vi "Main.vi"(11 "Module Admin":refnum<class "Delacor_lib_QMH_Module Admin.lvclass">) -> ()   [LabVIEW 2025, in "Scripting Server.lvlib"]
doc: "This template is based off of the Queued Message Handler design pattern and the Queued Message Handler project template that ships with LabVIEW.\n\nThe main difference is that the queue is private to this module and communication between modules is performed via Broadcast and Request events.\n\nRequest events are wrapped in public API methods and are handled in the Event Handling Loop (EHL) of this VI. Any module can register for Broadcast events sent by this module. The EHL generates messages based on user interface actions.\n\nThe Message Handling Loop (MHL) processes messages generated by the EHL, or by other messages. The messages are string values, so new messages can be added easily to the Message Cases case structure in the MHL. Each message cluster can also provide an optional value for Message Data, which is a variant that can be converted to whatever message-specific data is required.\n_____\nBased on DQMH Dev Tools: Project Template 7.1.0.1503."
uses:
  Scripting Server.lvlib
  <vilib>/Delacor/Delacor QMH/Libraries/Module Admin_class/Delacor_lib_QMH_Module Admin.lvclass
  <vilib>/Delacor/Delacor QMH/Libraries/Message Queue_class/Delacor_lib_QMH_Message Queue.lvclass
  Module Data--cluster.ctl
  <vilib>/Utility/miscctls.llb/LVPointTypeDef.ctl
  <vilib>/Delacor/Delacor QMH/Libraries/Message Queue_class/Delacor_lib_QMH_Enqueue Message (Single).vi
  Stop Argument--cluster.ctl
  New VI (Reply Payload)--cluster.ctl
  New VI Argument--cluster.ctl
  Add Object Argument--cluster.ctl
  Add Object (Reply Payload)--cluster.ctl
  Connect Objects (Reply Payload)--cluster.ctl
  Connect Objects Argument--cluster.ctl
  Get Object Terminals (Reply Payload)--cluster.ctl
  Get Object Terminals Argument--cluster.ctl
  get vi error list (Reply Payload)--cluster.ctl
  get vi error list Argument--cluster.ctl
  Cleanup VI (Reply Payload)--cluster.ctl
  Cleanup VI Argument--cluster.ctl
  create_control (Reply Payload)--cluster.ctl
  create_control Argument--cluster.ctl
  Run VI (Reply Payload)--cluster.ctl
  Run VI Argument--cluster.ctl
  add_to_selection (Reply Payload)--cluster.ctl
  add_to_selection Argument--cluster.ctl
  clear_selection_list (Reply Payload)--cluster.ctl
  clear_selection_list Argument--cluster.ctl
  remove_from_selection (Reply Payload)--cluster.ctl
  remove_from_selection Argument--cluster.ctl
  enclose_selection (Reply Payload)--cluster.ctl
  enclose_selection Argument--cluster.ctl
  rename_object (Reply Payload)--cluster.ctl
  rename_object Argument--cluster.ctl
  set_value (Reply Payload)--cluster.ctl
  set_value Argument--cluster.ctl
  delete_object (Reply Payload)--cluster.ctl
  delete_object Argument--cluster.ctl
  save_vi (Reply Payload)--cluster.ctl
  save_vi Argument--cluster.ctl
  get_structure_diagram (Reply Payload)--cluster.ctl
  get_structure_diagram Argument--cluster.ctl
  add_subvi (Reply Payload)--cluster.ctl
  add_subvi Argument--cluster.ctl
  connect_to_pane (Reply Payload)--cluster.ctl
  connect_to_pane Argument--cluster.ctl
  get_object_help (Reply Payload)--cluster.ctl
  get_object_help Argument--cluster.ctl
  get_loop_conditional_terminal (Reply Payload)--cluster.ctl
  get_loop_conditional_terminal Argument--cluster.ctl
  show_conditional_terminal (Reply Payload)--cluster.ctl
  show_conditional_terminal Argument--cluster.ctl
  get_loop_iteration_terminal (Reply Payload)--cluster.ctl
  get_loop_iteration_terminal Argument--cluster.ctl
  Config Data.ctl
  Read Config Data Argument--cluster.ctl
  get_allowed_paths (Reply Payload)--cluster.ctl
  get_allowed_paths Argument--cluster.ctl
  create_project (Reply Payload)--cluster.ctl
  create_project Argument--cluster.ctl
  Set Allowed Paths Argument--cluster.ctl
  open_vi (Reply Payload)--cluster.ctl
  open_vi Argument--cluster.ctl
  New MCP RPC Message Argument--cluster.ctl
  <vilib>/jgoebel/LabVIEW MCP Server SDK/MCP Server.lvlib
  <vilib>/jgoebel/LabVIEW MCP Server SDK/onRpc.ctl
  <vilib>/jgoebel/LabVIEW MCP Server SDK/User Events.ctl
  get-available-objects (Reply Payload)--cluster.ctl
  get-available-objects Argument--cluster.ctl
  Get open VIs (Reply Payload)--cluster.ctl
  Get open VIs Argument--cluster.ctl
  Get VI Blockdiagram (Reply Payload)--cluster.ctl
  Get VI Blockdiagram Argument--cluster.ctl
  Get VI Frontpanel Picture (Reply Payload)--cluster.ctl
  Get VI Frontpanel Picture Argument--cluster.ctl
  Get Library (Reply Payload)--cluster.ctl
  Get Library Argument--cluster.ctl
panel:
  out "Log":string
  in  "Ring 2":i32(ring)=2125 items=[".NET Container"=2125, ".NET Refnum"=3441, "2D Picture"=3508, "3D Picture"=23776, "Absolute Value"=1054, "Accept TLS"=1732, "Access Rights"=1412, "ActiveX Container"=2072, "Add"=1050, "Add (with error terminals)"=3915, "Add Array Elements"=1903, "Add Entropy"=1738, "Add Private Key To TLS Configuration"=1735, "Add Trusted Certificate To TLS Configuration"=1736, "Agitator"=3831, "AllSpoll"=1960, "Always Copy"=2400, "And"=1061, "And Array Elements"=1911, "Append True/False String"=1511, "Application Refnum"=3412, "Array (block diagram constant)"=2070, "Array (classic)"=3300, "Array (modern)"=21608, "Array Interface Control"=23777, "Array Max & Min"=1907, "Array of Strings to Path"=1422, "Array Size"=1809, "Array Subset"=2044, "Array To Cluster"=1168, "Array To Spreadsheet String"=1540, "ArrayMemInfo"=2412, "Assert Structural Type Match"=2416, "Assert Structural Type Mismatch"=2464, "Atmospheric Tank (classic)"=3070, "Atmospheric Tank (modern)"=21751, "Automation Close"=8001, "Automation Open"=8000, "Automation Refnum"=3410, "Avogadro Constant (1/mol)"=23520, "Base 10 Logarithm Of e"=23512, "Bin #1"=3073, "Bin #2"=21755, "Bitpack to Array"=3135, "Bluetooth Close Connection"=9148, "Bluetooth Create Listener"=9151, "Bluetooth Discover"=9152, "Bluetooth Network Connection Refnum"=3468, "Bluetooth Open Connection"=9153, "Bluetooth Read"=9149, "Bluetooth Wait On Listener"=9147, "Bluetooth Write"=9150, "Boolean Array To Number"=1815, "Boolean To (0,1)"=1167, "Build Array"=2041, "Build Cluster Array"=2047, "Build Map"=2463, "Build Matrix"=8500, "Build Path"=1419, "Build Set"=2462, "Build Waveform"=2066, "Bundle"=2049, "Bundle By Name"=2057, "Byte Array To String"=1609, "Byte Array To UTF-8 String"=1651, "Byte Stream File Refnum"=3408, "Call By Reference"=3901, "Call Chain"=1999, "Call Library Function Node"=2062, "Call MATLAB Function"=24210, "Call Parent Class Method"=2354, "CAN Channel (block diagram constant)"=2124, "CAN Channel (classic)"=3340, "CAN Channel (modern)"=21817, "CAN Channel (system)"=21966, "CAN Interface (block diagram constant)"=2123, "CAN Interface (classic)"=3339, "CAN Interface (modern)"=21815, "CAN Interface (system)"=21964, "CAN Task (block diagram constant)"=3471, "CAN Task (classic)"=3470, "CAN Task (modern)"=21789, "CAN Task (system)"=21963, "Cancel Button (modern)"=21739, "Cancel Button (system)"=3131, "Cancel Notification"=9107, "Carriage Return Constant"=23500, "Case Structure"=2001, "Cast Unit Bases"=1079, "Check Valve"=3833, "Checkbox (classic)"=3117, "CheckBox (modern)"=21924, "Checkbox (system)"=3132, "Class Specifier Constant"=2094, "Classic Color Box"=3013, "Classic Color Ramp"=3022, "Classic Horizontal Slide Switch"=3114, "Classic Vertical Slide"=3004, "Clear Fixed-Point Overflow Status"=5562, "Close File"=8052, "Close File (deprecated)"=1405, "Close MATLAB Session"=24209, "Close Python Session"=24207, "Close Reference"=8011, "Close TLS Configuration"=1741, "Close Variable Connection"=23783, "Closure Structure"=2372, "Cluster (classic)"=3400, "Cluster (modern)"=21607, "Cluster Constant"=2071, "Cluster To Array"=1169, "Code Interface Node"=2050, "Coerce To Type"=2402, "Collection Size"=2450, "Color Box Constant"=2120, "Color Box Thin Border"=2905, "Colored Rectangle (broken?)"=3625, "Combo Box (classic)"=3304, "Combo Box (modern)"=21604, "Combo Box (system)"=21917, "Combo Box Constant"=2088, "Complex Conjugate"=1048, "Complex To Polar"=1045, "Complex To Re/Im"=1044, "Compound Arithmetic"=2200, "Compressor"=3832, "Concatenate Strings"=2040, "Conditional Disable Structure"=2064, "Constructor Node"=3904, "Control & Simulation Loop"=2099, "Control Help Window"=1353, "Control Online Help"=1355, "Control Refnum"=3419, "Convert Unit"=2059, "Conveyer"=3827, "Copy"=8053, "Copy (deprecated)"=1416, "Cosecant"=1204, "Cosine"=1201, "Cotangent"=1205, "CPU Information"=24130, "Create Folder"=8055, "Create Network Stream Endpoint"=23793, "Create Network Stream Reader Endpoint"=23811, "Create Network Stream Writer Endpoint"=23810, "Create Stream"=23796, "Create Unique Network Stream Endpoint"=23795, "Create Unique Network Stream Reader Endpoint"=23807, "Create Unique Network Stream Writer Endpoint"=23806, "Create User Event"=2073, "Current Processor ID"=24131, "Current VI's Menubar"=9000, "Current VI's Path"=1426, "DAQmx Analog Trigger Source (block diagram constant)"=2119, "DAQmx Analog Trigger Source (classic)"=3336, "DAQmx Analog Trigger Source (modern)"=21774, "DAQmx Analog Trigger Source (system)"=21951, "DAQmx Device Name (block diagram constant)"=2093, "DAQmx Device Name (classic)"=3318, "DAQmx Device Name (modern)"=21773, "DAQmx Device Name (system)"=21950, "DAQmx Global Channel (block diagram constant)"=3430, "DAQmx Global Channel (classic)"=3443, "DAQmx Global Channel (modern)"=21770, "DAQmx Global Channel (system)"=21957, "DAQmx Physical Channel (block diagram constant)"=2118, "DAQmx Physical Channel (classic)"=3335, "DAQmx Physical Channel (modern)"=21777, "DAQmx Physical Channel (system)"=21954, "DAQmx Scale Name (block diagram constant)"=2116, "DAQmx Scale Name (classic)"=3317, "DAQmx Scale Name (modern)"=21775, "DAQmx Scale Name (system)"=21952, "DAQmx Switch (block diagram constant)"=2121, "DAQmx Switch (classic)"=3337, "DAQmx Switch (modern)"=21776, "DAQmx Switch (system)"=21953, "DAQmx Task Name (block diagram constant)"=3434, "DAQmx Task Name (classic)"=3442, "DAQmx Task Name (modern)"=21778, "DAQmx Task Name (system)"=21959, "DAQmx Terminal (block diagram constant)"=2117, "DAQmx Terminal (classic)"=3319, "DAQmx Terminal (modern)"=21781, "DAQmx Terminal (system)"=21955, "Data Cache Size"=24132, "Data Log File Refnum"=3402, "Data Value Reference"=3476, "Data Value Reference Constant"=24134, "DataSocket Close"=1085, "DataSocket Open"=1084, "DataSocket Read"=1086, "DataSocket Refnum"=3417, "DataSocket Write"=1087, "Date/Time To Seconds"=1308, "Decimal Digit?"=1119, "Decimal String To Number"=1184, "Decimate 1D Array"=2046, "DecomposeLockDataValRef"=2406, "DecomposeVariant"=2404, "Decrement"=1058, "Default Directory"=1427, "Delete"=8056, "Delete (deprecated)"=1417, "Delete Data Value Reference"=2409, "Delete From Array"=3912, "Delete Menu Items"=9004, "Delete Variant Attribute"=8206, "Delete Waveform Attribute"=8209, "Deny Access"=8057, "Dequeue Element"=9113, "Destroy Stream Endpoint"=23794, "Destroy User Event"=2075, "DevClear"=1961, "DevClearList"=1962, "Device Control/Status"=1433, "Device Refnum"=3405, "Diagram Disable Structure"=2054, "Dial (classic)"=3050, "Dial (modern)"=21732, "Digital Data (classic)"=3210, "Digital Data (modern)"=21216, "Digital Waveform Graph (classic)"=3511, "Digital Waveform Graph (modern)"=21718, "Direct Variable Read"=23785, "Direct Variable Write"=23788, "Divide"=1053, "Divide (with error terminals)"=3918, "Dlg Horiz Scrollbar"=21905, "Dlg Mac Group Box"=32514, "Dlg Numeric #1"=2100, "Dlg Numeric #2"=3006, "Dlg String"=2110, "Dlg Vert Scrollbar"=21906, "Down Arrow"=3824, "Down Bow Valve (flat)"=3707, "Down Bow Valve (outline)"=3807, "Down Bow Valve (shaded)"=21767, "Down Rect Valve (flat)"=3706, "Down Rect Valve (outline)"=3806, "Down Rect Valve (shaded)"=21766, "Down Tee (flat)"=3818, "Down Tee (shaded)"=3718, "Dynamic FPGA Interface Cast"=5690, "Eased Corner Rectangle"=32513, "Element of Set?"=2454, "Elementary Charge (C)"=23517, "Empty Array?"=23063, "Empty Collection?"=2451, "Empty Path Constant"=23523, "Empty String Constant"=23503, "Empty String/Path?"=1112, "Enable Menu Tracking"=9002, "EnableLocal"=1963, "EnableRemote"=1964, "End of Line Constant"=23525, "Enqueue Element"=9111, "Enqueue Element At Opposite End"=9129, "Enum (classic)"=3023, "Enum (modern)"=21605, "Enum (system)"=3062, "Enum Constant"=2090, "EOF"=1410, "Equal To 0?"=1113, "Equal?"=1102, "Error Ring Constant"=2039, "Event Callback Refnum"=3435, "Event Data Node"=2102, "Event Structure"=2052, "Exchanger"=3828, "Exclusive Or"=1063, "Exponential"=1211, "Exponential (Arg) -1"=1222, "Expression Node"=2201, "False Constant"=2006, "Feedback Node"=2353, "FieldPoint IO Point (block diagram constant)"=3440, "FieldPoint IO Point (classic)"=3439, "FieldPoint IO Point (modern)"=21784, "FIFO Refnum"=3474, "File Dialog"=8058, "File Dialog (deprecated)"=8081, "File Path Control (classic)"=3203, "File Path Control (modern)"=21730, "File Path Control (system)"=21922, "File Path Indicator (classic)"=3204, "File Path Indicator (modern)"=21731, "File/Directory Info"=8082, "File/Directory Info (deprecated)"=1413, "FindLstn"=1965, "FindRQS"=1966, "First Call?"=1083, "Fixed-Point Overflow?"=5565, "Fixed-Point to Integer Cast"=5566, "Flat Box"=3602, "Flat Circle"=3605, "Flat Down Triangle"=3623, "Flat Frame"=3608, "Flat Left Triangle"=3620, "Flat Right Triangle"=3621, "Flat Round Button"=3102, "Flat Rounded Box"=3611, "Flat Sequence Structure"=2069, "Flat Square Button"=3103, "Flat Up Triangle"=3622, "Flatten To JSON"=24201, "Flatten To String"=1164, "Flatten To XML"=8402, "Flattened String To Variant"=8202, "Floating Point Equal?"=23064, "Flush Event Queue"=2135, "Flush File"=8059, "Flush File (deprecated)"=1406, "Flush Queue"=9114, "Flush Stream"=23808, "For Loop"=2002, "Fork"=2194, "Format Date/Time String"=8100, "Format Into File"=2083, "Format Into String"=2081, "Format Value"=1512, "Formula Node"=2004, "FPGA Refnum to Session"=2322, "Fract/Exp String To Number"=1187, "Framed Color Box (classic)"=3008, "Framed Color Box (modern)"=21019, "Free Label"=2321, "Furnace"=3829, "Gauge (classic)"=3040, "Gauge (modern)"=21009, "Gauge for Simon"=32600, "Generate Front Panel Activity"=1329, "Generate Occurrence"=1700, "Generate User Event"=2074, "Generate User-Defined Trace Event"=2250, "Get Control Values by Index"=24204, "Get Datalog Position"=8061, "Get Date/Time In Seconds"=1303, "Get Date/Time String"=1600, "Get Drag Drop Data"=9154, "Get File Position"=8062, "Get File Size"=8063, "Get Fixed-Point Components"=11163, "Get Help Window Status"=1354, "Get Matrix Diagonal"=8501, "Get Matrix Elements"=8502, "Get Menu Item Info"=9005, "Get Menu Selection"=9001, "Get Menu Short Cut Info"=9007, "Get Notifier Status"=9103, "Get Number of Records"=8064, "Get Permissions"=8065, "Get Queue Status"=9110, "Get Submatrix"=8503, "Get Type and Creator"=8066, "Get Variant Attribute"=8205, "Get Volume Info"=8067, "Get Waveform Attribute"=8208, "Get Waveform Components"=2067, "Global Variable"=2060, "GPIB Clear"=1954, "GPIB Initialization"=1957, "GPIB Misc"=1956, "GPIB Read"=1951, "GPIB Serial Poll"=1955, "GPIB Status"=1959, "GPIB Trigger"=1953, "GPIB Wait"=1958, "GPIB Write"=1950, "Gravitational Constant (N m2/kg2)"=23519, "Greater Or Equal To 0?"=1114, "Greater Or Equal?"=1103, "Greater Than 0?"=1117, "Greater?"=1110, "Handle Peek"=1604, "Handle Poke"=1605, "Hex Digit?"=1123, "Hexadecimal String To Number"=1185, "Hopper #1"=21754, "Hopper #2"=3072, "Horiz Line"=3821, "Horiz Pipe (flat)"=3810, "Horiz Pipe (shaded)"=3710, "Horizontal Button Box"=3636, "Horizontal Fill Slide (classic)"=3012, "Horizontal Fill Slide (modern)"=21100, "Horizontal Gradient Oval"=32502, "Horizontal Gradient Rectangle"=32504, "Horizontal Gradient Rounded Rectangle"=32507, "Horizontal Graduated Bar"=21106, "Horizontal Pointer Slide (classic)"=3011, "Horizontal Pointer Slide (modern)"=21101, "Horizontal Pointer Slide (system)"=21902, "Horizontal Progress Bar (modern)"=21102, "Horizontal Progress Bar (system)"=21910, "Horizontal Scrollbar"=21110, "Horizontal Slide (classic)"=3010, "Horizontal Slide (system)"=21904, "Horizontal Smooth Box"=3633, "Horizontal Splitter Bar"=21861, "Horizontal Splitter Bar (Classic)"=21863, "Horizontal Splitter Bar (NXG Style)"=21867, "Horizontal Splitter Bar (System)"=21865, "Horizontal Switch"=3108, "Horizontal Tank"=3071, "Horizontal Toggle Switch (classic)"=3110, "Horizontal Toggle Switch (modern)"=21700, "Hyperbolic Cosecant"=23053, "Hyperbolic Cosine"=1215, "Hyperbolic Cotangent"=23055, "Hyperbolic Secant"=23054, "Hyperbolic Sine"=1214, "Hyperbolic Tangent"=1216, "IMAQ Session"=3415, "Implies"=1080, "In Place Element Structure"=2360, "In Range and Coerce"=1127, "Include Fixed-Point Overflow Status"=5564, "Increment"=1057, "Index & Bundle Cluster Array"=2056, "Index Array"=2042, "Index String Array"=1531, "Initialize Array"=2053, "Inline C Node"=2104, "Insert Into Array"=3911, "Insert Into Map"=2456, "Insert Into Set"=2452, "Insert Menu Items"=9003, "Integer to Fixed-Point Cast"=5567, "Intensity Chart (classic)"=3509, "Intensity Chart (modern)"=21719, "Intensity Graph (classic)"=3510, "Intensity Graph (modern)"=21720, "Interleave 1D Arrays"=2045, "Interpolate 1D Array"=1905, "Inverse Cosecant"=23050, "Inverse Cosine"=1207, "Inverse Cotangent"=23052, "Inverse Hyperbolic Cosecant"=23056, "Inverse Hyperbolic Cosine"=1218, "Inverse Hyperbolic Cotangent"=23058, "Inverse Hyperbolic Secant"=23057, "Inverse Hyperbolic Sine"=1217, "Inverse Hyperbolic Tangent"=1219, "Inverse Secant"=23051, "Inverse Sine"=1206, "Inverse Tangent"=1208, "Inverse Tangent (2 Input)"=1228, "Invoke Node"=3900, "IP To String"=1710, "IrDA Close Connection"=9144, "IrDA Create Listener"=9140, "IrDA Discover"=9141, "IrDA Network Connection Refnum"=3450, "IrDA Open Connection"=9142, "IrDA Read"=9145, "IrDA Wait On Listener"=9143, "IrDA Write"=9146, "IsDebuggingActive"=2403, "IVI Delete Session"=8103, "IVI Logical Name (block diagram constant)"=3420, "IVI Logical Name (classic)"=3414, "IVI Logical Name (modern)"=21736, "IVI New Session"=8102, "Join"=2195, "Join Numbers"=1171, "Junction"=2197, "Knob (classic)"=3005, "Knob (modern)"=21000, "Label (modern)"=21960, "Label (system)"=21961, "Labeled Oblong Button"=3125, "Labeled Rectangular Button"=3124, "Labeled Round Button"=3122, "Labeled Square Button"=3123, "LabVIEW Object"=3457, "Leak Variant Value Reference"=2410, "LED Button"=3116, "Left Arrow"=3826, "Left Bow Valve (flat)"=3701, "Left Bow Valve (outline)"=3801, "Left Bow Valve (shaded)"=21761, "Left Down Elbow (flat)"=3811, "Left Down Elbow (shaded)"=3711, "Left Pump (flat)"=3813, "Left Pump (shaded)"=3713, "Left Rect Valve (flat)"=3700, "Left Rect Valve (outline)"=3800, "Left Rect Valve (shaded)"=21760, "Left Tee (flat)"=3809, "Left Tee (shaded)"=3709, "Left Up Elbow (flat)"=3808, "Left Up Elbow (shaded)"=3708, "Less Or Equal To 0?"=1115, "Less Or Equal?"=1104, "Less Than 0?"=1118, "Less?"=1111, "Lexical Class"=1126, "Line (chiseled, system)"=3632, "Line (chiseled, thick)"=3630, "Line (chiseled, thin)"=3627, "Line (thick)"=3629, "Line (thin)"=3626, "Line Feed Constant"=23501, "Line with Arrow (thick)"=3631, "Line with Arrow (thin)"=3628, "List Directory"=1418, "List Folder"=8083, "Listbox (classic)"=21806, "Listbox (modern)"=21792, "Listbox (system)"=21805, "Listbox Symbol Ring Constant"=2038, "Load Certificates Into Memory"=1734, "Load Private Key Into Memory"=1733, "Local Variable"=2061, "Lock Range"=1411, "Logarithm Base 10"=1210, "Logarithm Base 2"=1225, "Logarithm Base X"=1224, "Logical Shift"=1081, "Look In Map"=2458, "Lookup Channel Probe"=9155, "Lossy Enqueue Element"=9130, "Lowered Box (thick)"=3635, "Lowered Rounded Box"=3638, "Machine Epsilon"=23528, "Make TLS Configuration Immutable"=1737, "MakeAddr"=1967, "Mantissa & Exponent"=1150, "Map"=3488, "Map Constant"=2461, "Match First String"=1532, "Match Pattern"=1535, "Match True/False String"=1533, "MathScript Call By Reference"=3906, "MathScript Node"=2357, "MATLAB script"=9020, "MATLAB Session Refnum"=3490, "Matrix Size"=8507, "Max & Min"=1108, "Menu Refnum"=3413, "Menu Ring (classic)"=3018, "Menu Ring (modern)"=21600, "Menu-Popup Ring"=3017, "Merge Errors"=2147, "Merge Signals"=2350, "Meter (classic)"=3030, "Meter (modern)"=21008, "Mixed Checkbox (system)"=21333, "Mixed Signal Graph"=21721, "Molar Gas Constant (J/(mol K))"=23522, "Motion Resource (block diagram constant)"=3449, "Motion Resource (classic)"=3448, "Motion Resource (modern)"=21787, "Motor (flat)"=3820, "Motor (shaded)"=3720, "Move"=8068, "Move (deprecated)"=1415, "Multi-Segment Pipe"=23780, "Multicolumn Listbox (classic)"=21799, "Multicolumn Listbox (modern)"=21791, "Multicolumn Listbox (system)"=21798, "Multiply"=1052, "Multiply (with error terminals)"=3917, "Multiply Array Elements"=1904, "Multirate Structure"=2199, "Natural Logarithm"=1209, "Natural Logarithm (Arg +1)"=1221, "Natural Logarithm Base"=23510, "Natural Logarithm Of 10"=23513, "Natural Logarithm Of 2"=23514, "Natural Logarithm Of Pi"=23508, "Negate"=1069, "Negative Infinity"=23509, "New Data Value Reference"=2408, "New Directory"=1402, "New File"=1404, "New TLS Configuration"=1730, "New VI"=8014, "New VI Object"=8015, "Not"=1064, "Not A Number/Path/Refnum?"=1128, "Not A Path Constant"=23524, "Not a Refnum Constant"=23526, "Not a Shared Variable"=23527, "Not And"=1071, "Not Equal To 0?"=1116, "Not Equal?"=1105, "Not Exclusive Or"=1073, "Not Or"=1072, "Notifier Refnum"=3423, "Number of Cache Levels"=24133, "Number To Boolean Array"=1814, "Number To Decimal String"=1180, "Number To Engineering String"=1183, "Number To Exponential String"=1505, "Number To Fractional String"=1506, "Number To Hexadecimal String"=1181, "Number To Octal String"=1182, "Numeric Constant"=2005, "Numeric Control (classic)"=3000, "Numeric Control (modern)"=21003, "Numeric Control (system)"=21919, "Numeric Indicator (classic)"=3001, "Numeric Indicator (modern)"=21004, "Obtain Notifier"=9101, "Obtain Queue"=9108, "Occurrence Refnum"=3406, "Octal Digit?"=1129, "Octal String To Number"=1186, "OK Button (modern)"=21738, "OK Button (system)"=3130, "Old VISA Open"=1921, "OLE Variant"=3150, "One Button Dialog"=1340, "Open and Verify Variable Connection"=23790, "Open Application Reference"=8012, "Open Device"=1430, "Open Dynamic Bitfile Reference"=5691, "Open File"=1403, "Open MATLAB Session"=24208, "Open Python Session"=24206, "Open Tank (flat classic)"=21752, "Open Tank (shaded classic)"=3074, "Open Variable Connection"=23779, "Open Variable Connection in Background"=23791, "Open VI Object Reference"=8013, "Open VI Reference"=8010, "Open/Create/Replace Datalog"=8054, "Open/Create/Replace File"=8050, "Or"=1062, "Or Array Elements"=1910, "Oval with Shadow"=32509, "Package Matrix"=23001, "PassControl"=1968, "Path Constant"=2009, "Path to Array of Strings"=1423, "Path To String"=1077, "Path Type"=1421, "Pi"=23504, "Pi Divided By 2"=23506, "Pi Multiplied By 2"=23505, "Pick Line"=1510, "Pict Ring (classic)"=3015, "Pict Ring (modern)"=21602, "Pict Ring (system)"=21925, "PixMap"=3505, "PixMap (warning: dangerous)"=3507, "Planck's Constant (J/Hz)"=23516, "Platform Flat Square Button"=3134, "Plug-In Control"=21820, "Polar To Complex"=1047, "Polar To Re/Im"=23061, "Positive Infinity"=23515, "Power Of 10"=1212, "Power Of 2"=1223, "Power Of X"=1213, "PPoll"=1969, "PPollConfig"=1970, "PPollUnconfig"=1971, "Preallocated Read from Binary File"=24135, "Preserve Run-Time Class"=8018, "Pressure Tank (flat)"=3075, "Pressure Tank (shaded)"=21753, "Preview Queue Element"=9112, "Printable?"=1124, "Property Node"=1920, "Pulldown Menu Ring"=3061, "Push Button"=21001, "Python Node"=24205, "Python Session Refnum"=3486, "Queue Refnum"=3424, "Quit LabVIEW"=1352, "Quotient & Remainder"=1056, "Race Structure"=2371, "Radio Button (system)"=3133, "Radio Buttons (classic)"=22003, "Radio Buttons (modern)"=22001, "Radio Buttons (system)"=22002, "Raised Box (classic)"=3600, "Raised Box (modern)"=3637, "Raised Circle"=3603, "Raised Down Triangle"=3615, "Raised Frame"=3606, "Raised Left Triangle"=3612, "Raised Right Triangle"=3613, "Raised Rounded Box"=3609, "Raised Up Triangle"=3614, "Random Number (0-1)"=1070, "RcvRespMsg"=1972, "Re-accept TLS"=1739, "Re/Im To Complex"=1046, "Re/Im To Polar"=23060, "Read Datalog"=8069, "Read Device"=1432, "Read File"=1407, "Read from Binary File"=8051, "Read from Text File"=8070, "Read Map Max & Min Keys"=2459, "Read Multiple Elements from Stream"=23803, "Read Set Max & Min"=2455, "Read Single Element from Stream"=23797, "Read Variable"=23781, "Read Variable with Timeout"=23786, "ReadStatus"=1973, "Receive"=1974, "ReceiveSetup"=1975, "Recessed Box"=3601, "Recessed Circle"=3604, "Recessed Down Triangle"=3619, "Recessed Frame (modern)"=3607, "Recessed Frame (system)"=3624, "Recessed Left Triangle"=3616, "Recessed Menu Ring"=3019, "Recessed Right Triangle"=3617, "Recessed Rounded Box"=3610, "Recessed Up Triangle"=3618, "Reciprocal"=1059, "Reciprocal Of e"=23511, "Reciprocal Of Pi"=23507, "RecomposeUnlockDataValRef (warning: dangerous)"=2407, "RecomposeVariant (warning: dangerous)"=2405, "Rectangular Stop Button"=3128, "Refnum to Path"=1424, "Refnum to Session"=2306, "Region"=2196, "Register Event Callback"=2078, "Register For Events"=2065, "Register Session"=2319, "Release Notifier"=9102, "Release Queue"=9109, "Remove Fixed-Point Overflow Status"=5563, "Remove From Map"=2457, "Remove From Set"=2453, "Replace Array Subset"=3910, "Replace Substring"=3913, "Request Deallocation"=1610, "ResetSys"=1976, "Reshape Array"=2055, "Resize Matrix"=8508, "Resource Index"=1088, "Reverse 1D Array"=1900, "Reverse String"=1537, "Right Arrow"=3825, "Right Bow Valve (flat)"=3705, "Right Bow Valve (outline)"=3805, "Right Bow Valve (shaded)"=21765, "Right Down Elbow (flat)"=3817, "Right Down Elbow (shaded)"=3717, "Right Pump (flat)"=3819, "Right Pump (shaded)"=3719, "Right Rect Valve (flat)"=3704, "Right Rect Valve (outline)"=3804, "Right Rect Valve (shaded)"=21764, "Right Tee (flat)"=3815, "Right Tee (shaded)"=3715, "Right Up Elbow (flat)"=3814, "Right Up Elbow (shaded)"=3714, "Rocker"=21002, "Rotary Feeder"=3830, "Rotate"=1082, "Rotate 1D Array"=1906, "Rotate Left With Carry"=1606, "Rotate Right With Carry"=1607, "Rotate String"=1536, "Round Button"=3100, "Round LED (classic)"=3120, "Round LED (modern)"=21012, "Round Light"=3104, "Round Push Button"=3118, "Round Push Button (profile)"=3112, "Round Radio Button"=3106, "Round Stop Button"=3127, "Round To Nearest"=1055, "Round Toward +Infinity"=1076, "Round Toward -Infinity"=1075, "Rounded Rectangle with Shadow"=32508, "RT FIFO Create"=24000, "RT FIFO Delete"=24003, "RT FIFO Read"=24001, "RT FIFO Write"=24002, "Rydberg Constant (1/m)"=23521, "Scale By Power Of 2"=1074, "Scan From File"=2082, "Scan From String"=2080, "Scan String For Tokens"=8101, "Scan Value"=1534, "Scanned Variable Read"=23784, "Scanned Variable Write"=23787, "Search 1D Array"=1901, "Search and Replace String"=3914, "Search Variable Container"=23802, "Search/Split String"=1538, "Secant"=1203, "Seconds To Date/Time"=1309, "Seek"=1409, "Select"=1516, "Send"=1977, "Send Notification"=9104, "SendCmds"=1978, "SendDataBytes"=1979, "SendIFC"=1980, "SendList"=1981, "SendLLO"=1982, "SendSetup"=1983, "Session to Refnum"=2307, "Set"=3487, "Set Constant"=2460, "Set Control Values by Index"=24203, "Set Datalog Position"=8072, "Set File Position"=8073, "Set File Size"=8074, "Set Matrix Diagonal"=8504, "Set Matrix Elements"=8505, "Set Menu Item Info"=9006, "Set Number of Records"=8075, "Set Occurrence"=1702, "Set Permissions"=8076, "Set Submatrix"=8506, "Set Type and Creator"=8077, "Set Variant Attribute"=8204, "Set Waveform Attribute"=8207, "SetRWLS"=1984, "SetTimeOut"=1985, "Shared Variable"=23778, "Shared Variable Constant"=3473, "Shared Variable Control (classic)"=3472, "Shared Variable Control (modern)"=21814, "Shared Variable to String"=1831, "Sign"=1049, "Simple Horizontal Slide"=3003, "Simple Numeric"=2900, "Simple String"=2115, "Simple Vertical Slide"=3002, "Sinc"=1227, "Sine"=1200, "Sine & Cosine"=1220, "Size Handle"=1603, "Slide Switch"=21011, "Smoothed Oval"=32500, "Smoothed Rounded Rectangle"=32505, "Sort 1D Array"=1120, "Sort Array of String"=23065, "Speed Of Light In Vacuum (m/sec)"=23518, "Spin Control (system)"=21900, "Split 1D Array"=1908, "Split Button"=21020, "Split Number"=1170, "Split Signals"=2351, "Spreadsheet String To Array"=1539, "Square"=23059, "Square Button"=3101, "Square LED (classic)"=3121, "Square LED (modern)"=21013, "Square Light"=3105, "Square Push Button"=3119, "Square Push Button (profile)"=3113, "Square Radio Button"=3107, "Square Root"=1060, "Stacked Sequence Structure"=2000, "Start TLS"=1731, "State"=2198, "State Diagram"=2051, "Static VI Reference"=2084, "Stop"=1350, "Stop Button"=21230, "String Constant"=2007, "String Control (classic)"=3200, "String Control (modern)"=21701, "String Control (system)"=21920, "String Indicator (classic)"=3201, "String Indicator (modern)"=21702, "String Length"=1502, "String Subset"=1503, "String To Byte Array"=1608, "String To IP"=1711, "String To Path"=1078, "String to Shared Variable"=1830, "Strip Path"=1420, "SubPanel"=21810, "SubPanel (Classic)"=21811, "SubPanel (NXG Style)"=21824, "SubPanel (System)"=21823, "Subtract"=1051, "Subtract (with error terminals)"=3916, "Swap Bytes"=1162, "Swap Values"=2401, "Swap Vector Element"=1912, "Swap Words"=1163, "Tab Constant"=23502, "Tab Control (classic)"=3330, "Tab Control (modern)"=3332, "Tab Control (NXG Style)"=32700, "Tab Control (system)"=3331, "Table (classic)"=21796, "Table (modern)"=21790, "Table (system)"=21797, "Tag Attribute Ring"=2063, "Tangent"=1202, "Tank (classic)"=3020, "Tank (modern)"=21006, "Target Structure"=2370, "TCP Close Connection"=1713, "TCP Create Listener"=1717, "TCP Flattened Read"=1718, "TCP Flattened Write"=1719, "TCP Flex Read"=1720, "TCP Flex Write"=1721, "TCP Network Connection Refnum"=3407, "TCP Open Connection"=1715, "TCP Read"=1716, "TCP Wait On Listener"=1712, "TCP Write"=1714, "TDMS Advanced Asynchronous Read (Data Ref)"=2151, "TDMS Advanced Asynchronous Write (Data Ref)"=2150, "TDMS Close"=24113, "TDMS Configure Asynchronous Reads (Data Ref)"=2153, "TDMS Configure Asynchronous Writes (Data Ref)"=2152, "TDMS Defragment"=24119, "TDMS Delete Data"=2159, "TDMS File"=3477, "TDMS Flush"=24117, "TDMS Get Asynchronous Read Status (Data Ref)"=2155, "TDMS Get Asynchronous Write Status (Data Ref)"=2154, "TDMS Get Properties"=24115, "TDMS In Memory Close"=2157, "TDMS In Memory Open"=2156, "TDMS In Memory Read Bytes"=2158, "TDMS List Contents"=24116, "TDMS Open"=24112, "TDMS Read"=24111, "TDMS Refnum To File ID"=24120, "TDMS Set Properties"=24114, "TDMS Write"=24110, "TDMS Write IP"=24118, "Temporary Directory"=1435, "TestSRQ"=1986, "TestSys"=1987, "Text & Pict Ring (classic)"=3016, "Text & Pict Ring (modern)"=21603, "Text Button"=21015, "Text Ring (block diagram constant)"=2008, "Text Ring (classic)"=3014, "Text Ring (modern)"=21601, "Text Ring (system)"=3060, "Text to UTF-8"=23066, "Thermometer (classic)"=3021, "Thermometer (modern)"=21007, "Threshold 1D Array"=1909, "Tick Count (ms)"=1300, "Time Stamp (block diagram constant)"=2068, "Time Stamp Control (classic)"=5555, "Time Stamp Control (modern)"=21913, "Time Stamp Control (system)"=21967, "Time Stamp Indicator (classic)"=5556, "Time Stamp Indicator (modern)"=21914, "Timed Loop"=5570, "Timed Sequence"=5573, "TLS configuration"=3489, "TLS Connection?"=1740, "To Byte Integer"=1140, "To Double Precision Complex"=1152, "To Double Precision Float"=1147, "To Extended Precision Complex"=1154, "To Extended Precision Float"=1149, "To Fixed-Point"=5561, "To Long Integer"=1142, "To Lower Case"=1189, "To More Generic Class"=8017, "To More Specific Class"=8016, "To OLE Variant"=8002, "To Probe String"=2413, "To Quad Integer"=1155, "To Single Precision Complex"=1151, "To Single Precision Float"=1146, "To Time Stamp"=5560, "To Unsigned Byte Integer"=1143, "To Unsigned Long Integer"=1145, "To Unsigned Quad Integer"=1156, "To Unsigned Word Integer"=1144, "To Upper Case"=1188, "To Variant"=8201, "To Word Integer"=1141, "Traditional DAQ Channel (block diagram constant)"=2085, "Traditional DAQ Channel (classic)"=3320, "Traditional DAQ Channel (modern)"=21733, "Transpose 1D Array"=23068, "Transpose 2D Array"=1902, "Transpose Matrix"=8509, "Tree (classic)"=21819, "Tree (modern)"=21793, "Tree (system)"=21794, "Trigger"=1988, "TriggerList"=1989, "Two Button Dialog"=1341, "Type and Creator"=1434, "Type Cast"=1166, "Type Error"=2415, "Type Must Be Array"=2417, "Type Must Be Cluster"=2418, "Type Of"=2414, "Type Specialization Structure"=2373, "UDP Close"=1726, "UDP Multicast Open"=1727, "UDP Network Connection Refnum"=3418, "UDP Open"=1723, "UDP Read"=1724, "UDP Write"=1725, "Unbitpack from Array"=3136, "Unbundle"=2048, "Unbundle By Name"=2058, "Unflatten From JSON"=24202, "Unflatten From String"=1165, "Unflatten From XML"=8401, "Unleak Variant Value Reference"=2411, "Unpackage Matrix"=23000, "Unregister For Events"=2076, "Unregister Session"=2320, "Up Arrow"=3823, "Up Bow Valve (flat)"=3703, "Up Bow Valve (outline)"=3803, "Up Bow Valve (shaded)"=21763, "Up Rect Valve (flat)"=3702, "Up Rect Valve (outline)"=21762, "Up Rect Valve (shaded)"=3802, "Up Tee (flat)"=3812, "Up Tee (shaded)"=3712, "User Defined Refnum"=3428, "User Defined Refnum Tag (block diagram constant)"=3426, "User Defined Refnum Tag (classic)"=3429, "User Defined Refnum Tag (modern)"=21745, "User Defined Refnum Tag Flatten (classic)"=3454, "User Defined Refnum Tag Flatten (modern)"=21747, "User Defined Tag (block diagram constant)"=2114, "User Defined Tag (classic)"=3329, "User Defined Tag (modern)"=21749, "User Item"=3506, "UTF-8 String To Byte Array"=1650, "UTF-8 to Text"=23067, "Variable Class Specifier Constant"=2106, "Variable Name Constant"=3478, "Variant"=3310, "Variant To Data"=8003, "Variant To Flattened String"=8203, "Vert Line"=3822, "Vert Pipe (flat)"=3816, "Vert Pipe (shaded)"=3716, "Vert Rocker"=21740, "Vertical Fill Slide (classic)"=3009, "Vertical Fill Slide (modern)"=21014, "Vertical Gradient Oval"=32501, "Vertical Gradient Rectangle"=32503, "Vertical Gradient Rounded Rectangle"=32506, "Vertical Graduated Bar"=21107, "Vertical Pointer Slide (classic)"=3007, "Vertical Pointer Slide (modern)"=21017, "Vertical Pointer Slide (system)"=21901, "Vertical Progress Bar (modern)"=21104, "Vertical Progress Bar (system)"=21909, "Vertical Scrollbar"=21111, "Vertical Slide (system)"=21903, "Vertical Slide Switch (classic)"=3115, "Vertical Slide Switch (modern)"=21741, "Vertical Smooth Box"=3634, "Vertical Splitter Bar"=21860, "Vertical Splitter Bar (Classic)"=21862, "Vertical Splitter Bar (NXG Style)"=21866, "Vertical Splitter Bar (System)"=21864, "Vertical Switch"=3109, "Vertical Toggle Switch (classic)"=3111, "Vertical Toggle Switch (modern)"=21005, "VI Library"=1425, "VI Refnum"=3422, "VI Server Reference"=2091, "VISA Assert Interrupt Signal"=2309, "VISA Assert Trigger"=1929, "VISA Assert Utility Signal"=2310, "VISA Clear"=1927, "VISA Close"=1922, "VISA Disable Event"=1940, "VISA Discard Events"=1941, "VISA Enable Event"=1942, "VISA Find Resource"=1923, "VISA Flush I/O Buffer"=2302, "VISA GPIB Command"=2315, "VISA GPIB Control ATN"=2316, "VISA GPIB Control REN"=2304, "VISA GPIB Pass Control"=2317, "VISA GPIB Send IFC"=2318, "VISA In 16"=1930, "VISA In 32"=1944, "VISA In 64"=2140, "VISA In 8"=1936, "VISA Lock"=1993, "VISA Map Address"=1932, "VISA Map Trigger"=2311, "VISA Memory Allocation"=1997, "VISA Memory Allocation Ex"=2146, "VISA Memory Free"=1998, "VISA Move"=2303, "VISA Move In 16"=1948, "VISA Move In 32"=1991, "VISA Move In 64"=2144, "VISA Move In 8"=1946, "VISA Move Out 16"=1949, "VISA Move Out 32"=1992, "VISA Move Out 64"=2145, "VISA Move Out 8"=1947, "VISA Open"=2308, "VISA Out 16"=1931, "VISA Out 32"=1945, "VISA Out 64"=2141, "VISA Out 8"=1937, "VISA Peek 16"=1934, "VISA Peek 32"=1995, "VISA Peek 64"=2142, "VISA Peek 8"=1938, "VISA Poke 16"=1935, "VISA Poke 32"=1996, "VISA Poke 64"=2143, "VISA Poke 8"=1939, "VISA Read"=1925, "VISA Read STB"=1928, "VISA Read To File"=2313, "VISA Refnum to Session"=2300, "VISA Resource Name"=3421, "VISA resource name (classic)"=3409, "VISA resource name (modern)"=21737, "VISA Set I/O Buffer Size"=2301, "VISA Status Description"=1924, "VISA Unlock"=1994, "VISA Unmap Address"=1933, "VISA Unmap Trigger"=2312, "VISA USB Control In"=2086, "VISA USB Control Out"=2087, "VISA VXI Cmd or Query"=2305, "VISA Wait on Event"=1943, "VISA Write"=1926, "VISA Write From File"=2314, "Volume Info"=1414, "Wait (ms)"=1302, "Wait For Activity"=1722, "Wait For Front Panel Activity"=1328, "Wait for GPIB RQS"=1952, "Wait on Notification"=9105, "Wait on Notification from Multiple"=9106, "Wait on Notification from Multiple with Notifier History"=9132, "Wait on Notification with Notifier History"=9131, "Wait on Occurrence"=1701, "Wait Until Next ms Multiple"=1327, "WaitSRQ"=1990, "Waveform Chart"=21010, "Waveform Chart (classic)"=3501, "Waveform Chart (modern)"=21717, "Waveform Graph (classic)"=3504, "Waveform Graph (modern)"=21703, "While Loop #1"=2003, "While Loop #2"=2352, "White Space?"=1125, "Write Datalog"=8079, "Write Device"=1431, "Write File"=1408, "Write Multiple Elements to Stream"=23804, "Write Single Element to Stream"=23798, "Write to Binary File"=8078, "Write to Text File"=8080, "Write Variable"=23782, "Write Variable with Timeout"=23789, "XY Graph (classic)"=3500, "XY Graph (modern)"=21716, "Y-th Root of X"=23062]
  out "error out":errorcluster
  out "Status":string
  in  "Simulate MHL Error":bool
  in  "Simulate EHL Error":bool
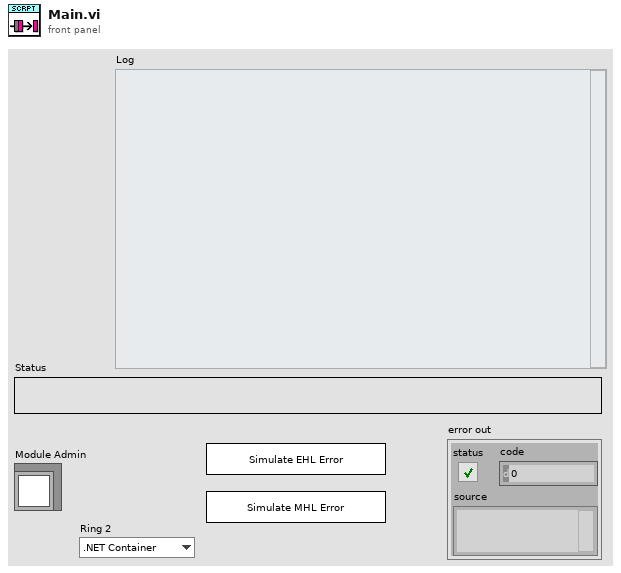
[diagram p1: front panel]
types:
  T1 = typedef "MCP Server.lvlib/User Events.ctl" = cluster{"onError":refnum<user-event>, "onRpc":refnum<user-event>}
  T2 = typedef "Scripting Server.lvlib/Request Events--cluster.ctl" = cluster{"Stop Module":refnum<user-event>, "Show Panel":refnum<user-event>, "Hide Panel":refnum<user-event>, "Get Module Execution Status":refnum<user-event>, "Show Diagram":refnum<user-event>, "New VI":refnum<user-event>, "Add Object":refnum<user-event>, "Connect Objects":refnum<user-event>, "Get Object Terminals":refnum<user-event>, "get vi error list":refnum<user-event>, "Cleanup VI":refnum<user-event>, "create_control":refnum<user-event>, "Run VI":refnum<user-event>, "add_to_selection":refnum<user-event>, "clear_selection_list":refnum<user-event>, "remove_from_selection":refnum<user-event>, "enclose_selection":refnum<user-event>, "rename_object":refnum<user-event>, "set_value":refnum<user-event>, "delete_object":refnum<user-event>, "save_vi":refnum<user-event>, "get_structure_diagram":refnum<user-event>, "add_subvi":refnum<user-event>, "connect_to_pane":refnum<user-event>, "get_object_help":refnum<user-event>, "get_loop_conditional_terminal":refnum<user-event>, "show_conditional_terminal":refnum<user-event>, "get_loop_iteration_terminal":refnum<user-event>, "Read Config Data":refnum<user-event>, "get_allowed_paths":refnum<user-event>, "create_project":refnum<user-event>, "Set Allowed Paths":refnum<user-event>, "open_vi":refnum<user-event>, "Private.Register MCP Events":refnum<user-event>, "New MCP RPC Message":refnum<user-event>, "get-available-objects":refnum<user-event>, "Get open VIs":refnum<user-event>, "Get VI Blockdiagram":refnum<user-event>, "Get VI Frontpanel Picture":refnum<user-event>, "Get Library":refnum<user-event>}
  T3 = typedef "Scripting Server.lvlib/Module Data--cluster.ctl" = cluster{"Status":string, "Current ID":i32, "References":variant, "Config Data":T4, "MCP id":i32, "Log":string}
  T4 = typedef "Scripting Server.lvlib/Config Data.ctl" = cluster{"Allowed Paths":string[]}
  T5 = enum32{"invalid lock state", "Not Locked", "Locked (No Password)", "Password-protected"}
  T6 = typedef "Scripting Server.lvlib/Stop Argument--cluster.ctl" = cluster{"Origin":string, "Exit via Stop Module Req?":bool, "Wait for Module to stop?":bool}
  T7 = typedef "Scripting Server.lvlib/New VI Argument--cluster.ctl" = cluster{"Open Frontpanel":bool, "Wait Notifier":refnum<notifier>, "wait for reply":bool}
  T8 = typedef "Scripting Server.lvlib/Add Object Argument--cluster.ctl" = cluster{"VI Reference":i32, "Object Name":string, "Wait Notifier":refnum<notifier>, "wait for reply":bool, "position_x":i32, "position_y":i32}
  T9 = typedef "Scripting Server.lvlib/Connect Objects Argument--cluster.ctl" = cluster{"vi reference":i32, "from object reference":i32, "to object reference":i32, "from object terminal index":i32, "to object terminal index":i32, "Wait Notifier":refnum<notifier>, "wait for reply":bool}
  T10 = typedef "Scripting Server.lvlib/Get Object Terminals Argument--cluster.ctl" = cluster{"object id":i32, "Wait Notifier":refnum<notifier>, "wait for reply":bool}
  T11 = typedef "Scripting Server.lvlib/get vi error list Argument--cluster.ctl" = cluster{"vi id":i32, "Wait Notifier":refnum<notifier>, "wait for reply":bool}
  T12 = typedef "Scripting Server.lvlib/Cleanup VI Argument--cluster.ctl" = cluster{"vi reference":i32, "Wait Notifier":refnum<notifier>, "wait for reply":bool}
  T13 = typedef "Scripting Server.lvlib/create_control Argument--cluster.ctl" = cluster{"Object ID":i32, "Terminal Index":i32, "Constant":bool, "Wait Notifier":refnum<notifier>, "wait for reply":bool, "Value":string}
  T14 = typedef "Scripting Server.lvlib/Run VI Argument--cluster.ctl" = cluster{"VI ID":i32, "open_frontpanel":bool, "Wait Notifier":refnum<notifier>, "wait for reply":bool}
  T15 = typedef "Scripting Server.lvlib/add_to_selection Argument--cluster.ctl" = cluster{"object_id":i32, "Wait Notifier":refnum<notifier>, "wait for reply":bool, "vi_id":i32}
  T16 = typedef "Scripting Server.lvlib/clear_selection_list Argument--cluster.ctl" = cluster{"Wait Notifier":refnum<notifier>, "wait for reply":bool, "vi_id":i32}
  T17 = typedef "Scripting Server.lvlib/remove_from_selection Argument--cluster.ctl" = cluster{"vi_id":i32, "object_id":i32, "Wait Notifier":refnum<notifier>, "wait for reply":bool}
  T18 = typedef "Scripting Server.lvlib/enclose_selection Argument--cluster.ctl" = cluster{"vi_id":i32, "structure_type":string, "Wait Notifier":refnum<notifier>, "wait for reply":bool}
  T19 = typedef "Scripting Server.lvlib/rename_object Argument--cluster.ctl" = cluster{"new_label_name":string, "label_visible":bool, "Wait Notifier":refnum<notifier>, "wait for reply":bool, "object_id":i32}
  T20 = typedef "Scripting Server.lvlib/set_value Argument--cluster.ctl" = cluster{"object_id":i32, "value":string, "Wait Notifier":refnum<notifier>, "wait for reply":bool}
  T21 = typedef "Scripting Server.lvlib/delete_object Argument--cluster.ctl" = cluster{"object_id":i32, "Wait Notifier":refnum<notifier>, "wait for reply":bool}
  T22 = typedef "Scripting Server.lvlib/save_vi Argument--cluster.ctl" = cluster{"vi_id":i32, "path":string, "Wait Notifier":refnum<notifier>, "wait for reply":bool}
  T23 = typedef "Scripting Server.lvlib/get_structure_diagram Argument--cluster.ctl" = cluster{"structure_id":i32, "index":i32, "Wait Notifier":refnum<notifier>, "wait for reply":bool}
  T24 = typedef "Scripting Server.lvlib/add_subvi Argument--cluster.ctl" = cluster{"diagram_id":i32, "subvi_path":string, "Wait Notifier":refnum<notifier>, "wait for reply":bool, "position_x":i32, "position_y":i32}
  T25 = typedef "Scripting Server.lvlib/connect_to_pane Argument--cluster.ctl" = cluster{"control_id":i32, "connector_pane_index":i32, "Wait Notifier":refnum<notifier>, "wait for reply":bool}
  T26 = typedef "Scripting Server.lvlib/get_object_help Argument--cluster.ctl" = cluster{"object_id":i32, "Wait Notifier":refnum<notifier>, "wait for reply":bool}
  T27 = typedef "Scripting Server.lvlib/get_loop_conditional_terminal Argument--cluster.ctl" = cluster{"loop_id":i32, "Wait Notifier":refnum<notifier>, "wait for reply":bool}
  T28 = typedef "Scripting Server.lvlib/show_conditional_terminal Argument--cluster.ctl" = cluster{"loop_id":i32, "show":bool, "Wait Notifier":refnum<notifier>, "wait for reply":bool}
  T29 = typedef "Scripting Server.lvlib/get_loop_iteration_terminal Argument--cluster.ctl" = cluster{"loop_id":i32, "Wait Notifier":refnum<notifier>, "wait for reply":bool}
  T30 = typedef "Scripting Server.lvlib/Read Config Data Argument--cluster.ctl" = cluster{"Boolean":bool}
  T31 = typedef "Scripting Server.lvlib/get_allowed_paths Argument--cluster.ctl" = cluster{"Wait Notifier":refnum<notifier>, "wait for reply":bool}
  T32 = typedef "Scripting Server.lvlib/create_project Argument--cluster.ctl" = cluster{"File Path":string, "Wait Notifier":refnum<notifier>, "wait for reply":bool}
  T33 = typedef "Scripting Server.lvlib/Set Allowed Paths Argument--cluster.ctl" = cluster{"Working Directory Folder Path":path[]}
  T34 = typedef "Scripting Server.lvlib/open_vi Argument--cluster.ctl" = cluster{"vi_path":string, "Wait Notifier":refnum<notifier>, "wait for reply":bool}
  T35 = typedef "Scripting Server.lvlib/New MCP RPC Message Argument--cluster.ctl" = cluster{"request":string, "response":string}
  T36 = typedef "Scripting Server.lvlib/get-available-objects Argument--cluster.ctl" = cluster{"Wait Notifier":refnum<notifier>, "wait for reply":bool}
  T37 = typedef "Scripting Server.lvlib/Get open VIs Argument--cluster.ctl" = cluster{"Wait Notifier":refnum<notifier>, "wait for reply":bool}
  T38 = typedef "Scripting Server.lvlib/Get VI Blockdiagram Argument--cluster.ctl" = cluster{"VI ID":i32, "Wait Notifier":refnum<notifier>, "wait for reply":bool}
  T39 = typedef "Scripting Server.lvlib/Get VI Frontpanel Picture Argument--cluster.ctl" = cluster{"VI ID":i32, "Wait Notifier":refnum<notifier>, "wait for reply":bool}
  T40 = typedef "Scripting Server.lvlib/Get Library Argument--cluster.ctl" = cluster{"Library Path":string, "Wait Notifier":refnum<notifier>, "wait for reply":bool}
  T41 = typedef "LVPointTypeDef.ctl" = cluster{"Horizontal":i16, "Vertical":i16}
  T42 = enum32{"Invalid", "Standard", "Closed", "Hidden", "Minimized", "Maximized"}
  T43 = typedef "Scripting Server.lvlib/New VI (Reply Payload)--cluster.ctl" = cluster{"VI Reference":i32, "Result":string, "error":errorcluster}
  T44 = typedef "Scripting Server.lvlib/Add Object (Reply Payload)--cluster.ctl" = cluster{"error":errorcluster, "Object ID":i32, "Result":string}
  T45 = typedef "Scripting Server.lvlib/Connect Objects (Reply Payload)--cluster.ctl" = cluster{"result":string, "error":errorcluster}
  T46 = typedef "Scripting Server.lvlib/Get Object Terminals (Reply Payload)--cluster.ctl" = cluster{"terminals description":string, "error":errorcluster}
  T47 = typedef "Scripting Server.lvlib/get vi error list (Reply Payload)--cluster.ctl" = cluster{"error list":string, "error":errorcluster}
  T48 = typedef "Scripting Server.lvlib/create_control (Reply Payload)--cluster.ctl" = cluster{"Object ID":i32, "error":errorcluster}
  T49 = typedef "Scripting Server.lvlib/Run VI (Reply Payload)--cluster.ctl" = cluster{"error":errorcluster}
  T50 = typedef "Scripting Server.lvlib/add_to_selection (Reply Payload)--cluster.ctl" = cluster{"Current Selection":i32[], "error":errorcluster}
  T51 = typedef "Scripting Server.lvlib/clear_selection_list (Reply Payload)--cluster.ctl" = cluster{"error":errorcluster}
  T52 = typedef "Scripting Server.lvlib/remove_from_selection (Reply Payload)--cluster.ctl" = cluster{"current_selection":i32[], "error":errorcluster}
  T53 = typedef "Scripting Server.lvlib/enclose_selection (Reply Payload)--cluster.ctl" = cluster{"object_id":i32, "error":errorcluster}
  T54 = typedef "Scripting Server.lvlib/rename_object (Reply Payload)--cluster.ctl" = cluster{"error":errorcluster}
  T55 = typedef "Scripting Server.lvlib/set_value (Reply Payload)--cluster.ctl" = cluster{"error":errorcluster}
  T56 = typedef "Scripting Server.lvlib/delete_object (Reply Payload)--cluster.ctl" = cluster{"error":errorcluster}
  T57 = typedef "Scripting Server.lvlib/save_vi (Reply Payload)--cluster.ctl" = cluster{"path_out":string, "error":errorcluster}
  T58 = typedef "Scripting Server.lvlib/get_structure_diagram (Reply Payload)--cluster.ctl" = cluster{"diagram_id":i32, "error":errorcluster}
  T59 = typedef "Scripting Server.lvlib/add_subvi (Reply Payload)--cluster.ctl" = cluster{"subvi_id":i32, "error":errorcluster}
  T60 = typedef "Scripting Server.lvlib/connect_to_pane (Reply Payload)--cluster.ctl" = cluster{"error":errorcluster}
  T61 = typedef "Scripting Server.lvlib/get_object_help (Reply Payload)--cluster.ctl" = cluster{"help_string":string, "error":errorcluster}
  T62 = typedef "Scripting Server.lvlib/get_allowed_paths (Reply Payload)--cluster.ctl" = cluster{"Allowed Paths":string, "error":errorcluster}
  T63 = typedef "Scripting Server.lvlib/get-available-objects (Reply Payload)--cluster.ctl" = cluster{"available objects":string, "error":errorcluster}
  T64 = typedef "Scripting Server.lvlib/Cleanup VI (Reply Payload)--cluster.ctl" = cluster{"result":string, "error":errorcluster}
  T65 = typedef "Scripting Server.lvlib/get_loop_conditional_terminal (Reply Payload)--cluster.ctl" = cluster{"conditional_terminal_id":i32, "error":errorcluster}
  T66 = typedef "Scripting Server.lvlib/show_conditional_terminal (Reply Payload)--cluster.ctl" = cluster{"error":errorcluster}
  T67 = typedef "Scripting Server.lvlib/get_loop_iteration_terminal (Reply Payload)--cluster.ctl" = cluster{"iteration_terminal_id":i32, "error":errorcluster}
  T68 = typedef "Scripting Server.lvlib/create_project (Reply Payload)--cluster.ctl" = cluster{"project_id":i32, "error":errorcluster}
  T69 = typedef "Scripting Server.lvlib/open_vi (Reply Payload)--cluster.ctl" = cluster{"vi_id":string, "error":errorcluster}
  T70 = typedef "Scripting Server.lvlib/Get Library (Reply Payload)--cluster.ctl" = cluster{"Library Content":string, "error":errorcluster}
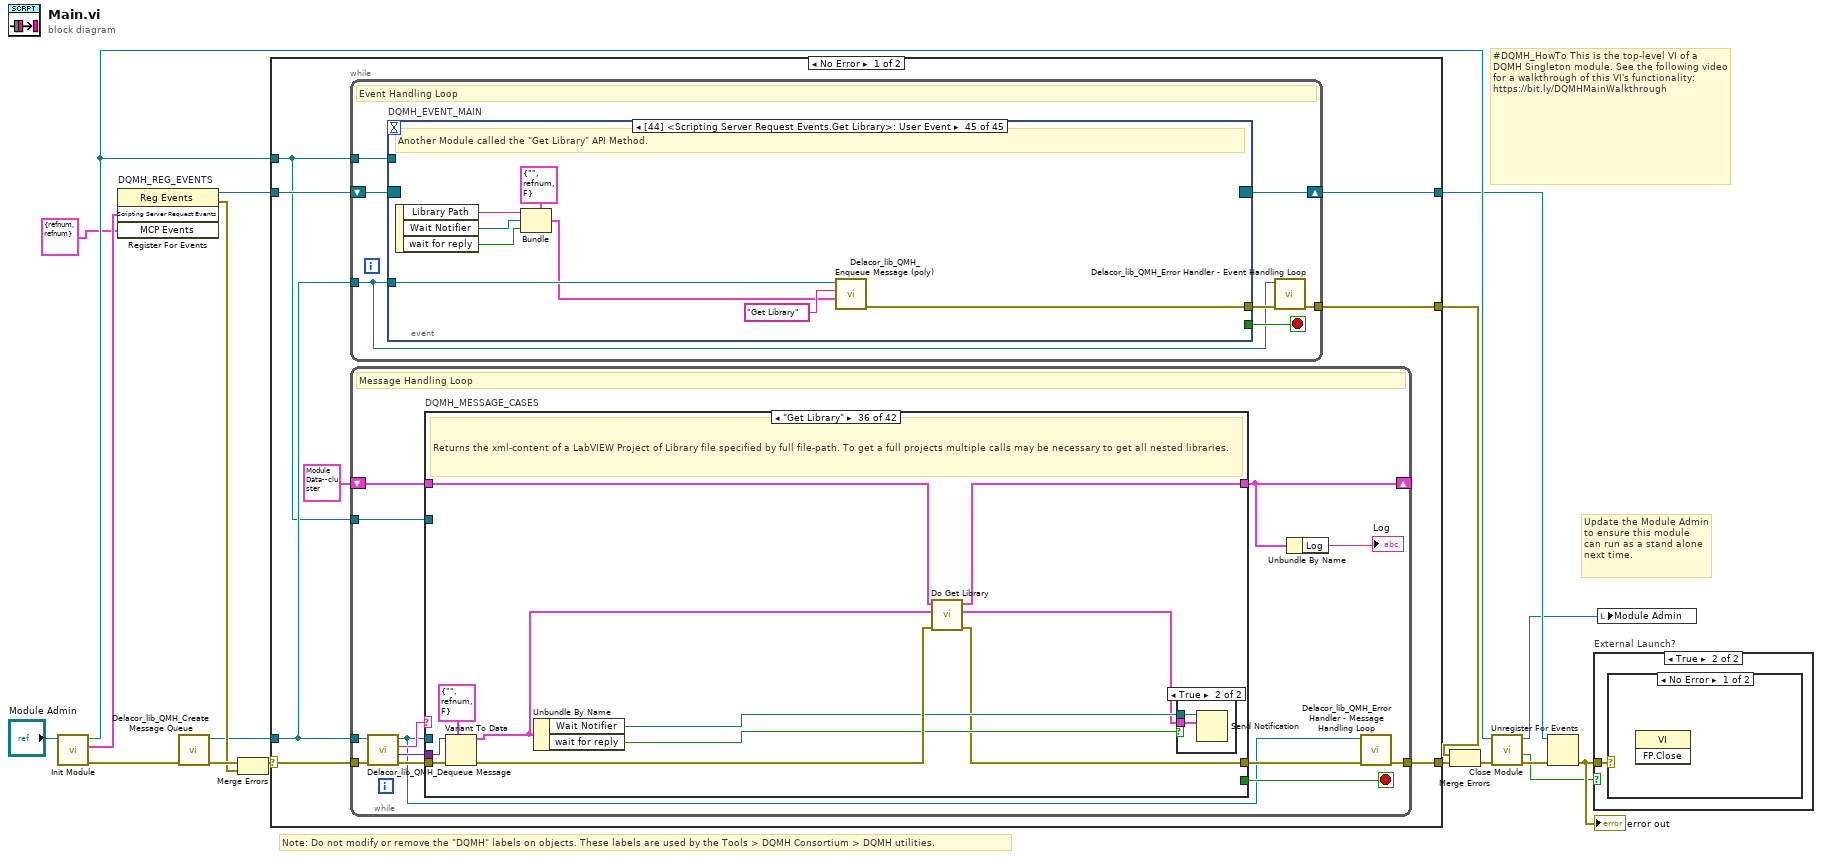
[diagram p0: block diagram]
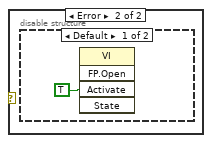
[diagram p3: hidden frame]
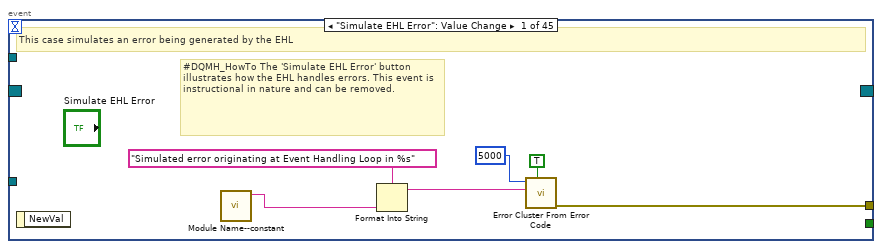
[diagram p5: hidden frame]
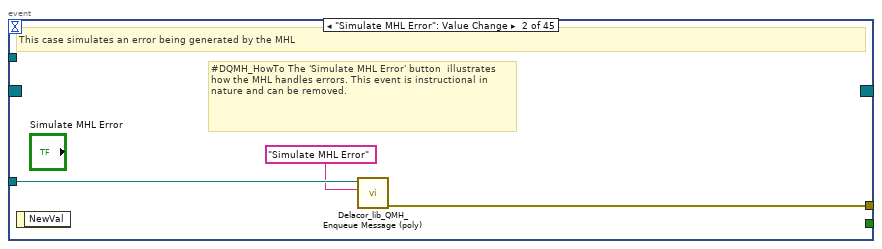
[diagram p6: hidden frame]
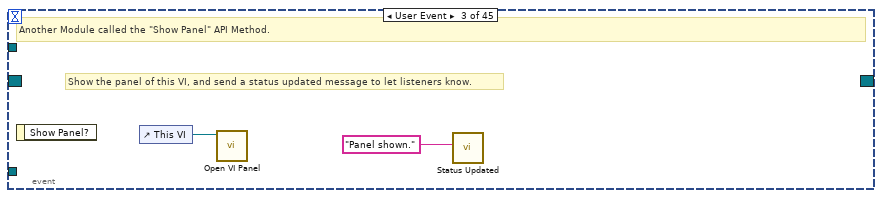
[diagram p7: hidden frame]
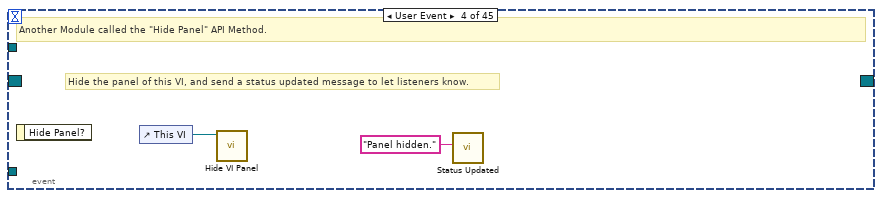
[diagram p8: hidden frame]
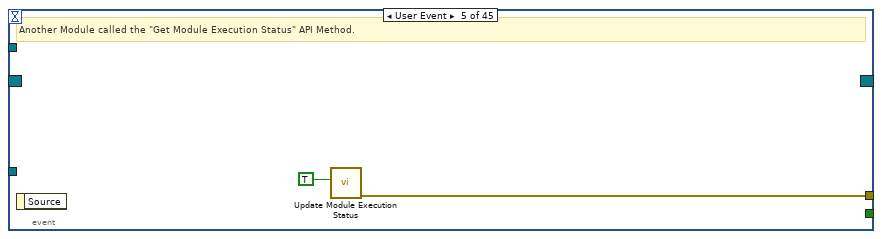
[diagram p9: hidden frame]
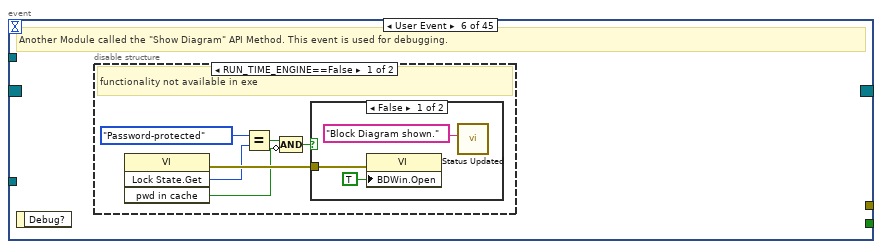
[diagram p10: hidden frame]
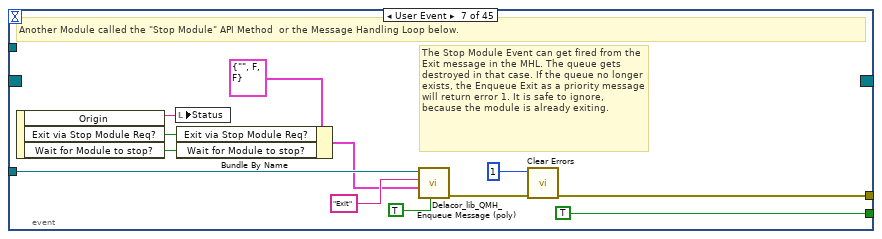
[diagram p13: hidden frame]
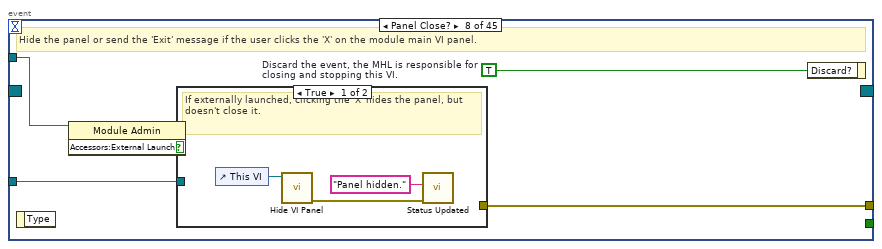
[diagram p14: hidden frame]
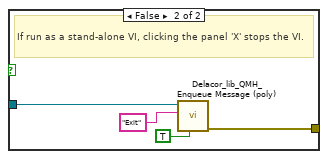
[diagram p15: hidden frame]
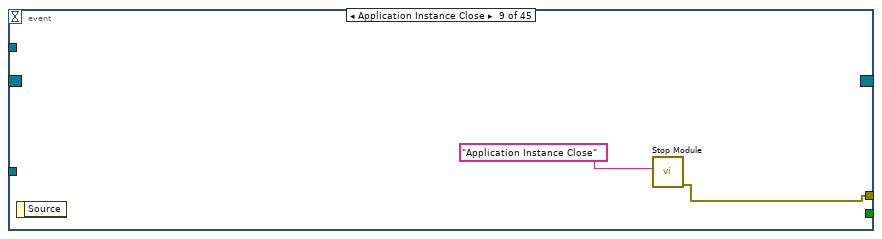
[diagram p16: hidden frame]
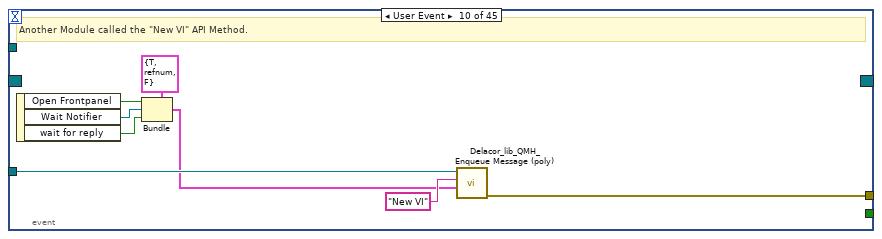
[diagram p17: hidden frame]
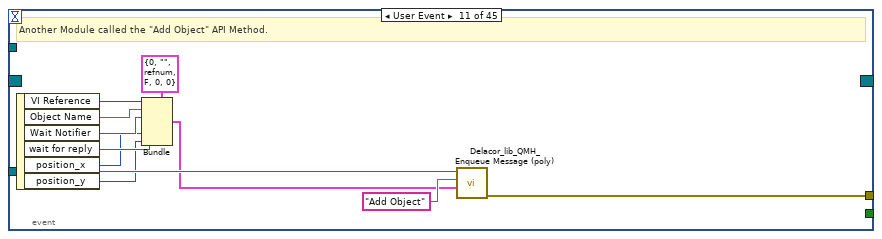
[diagram p18: hidden frame]
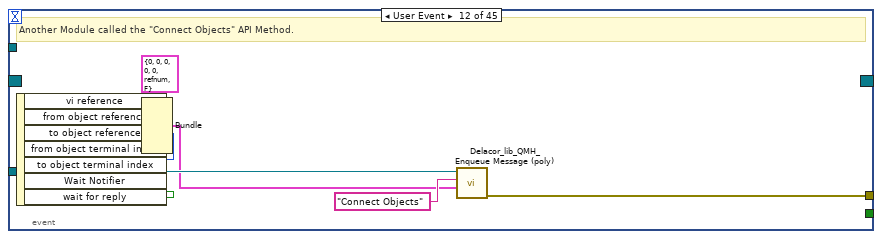
[diagram p19: hidden frame]
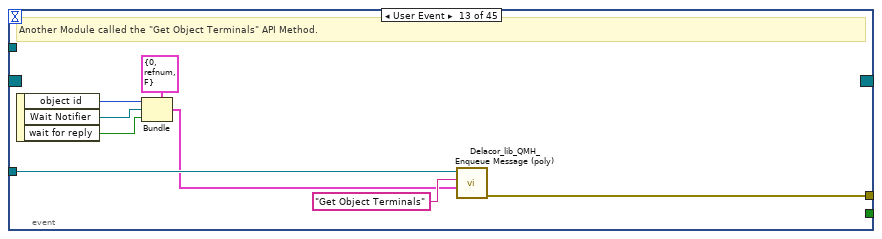
[diagram p20: hidden frame]
diagram:
  # "#DQMH_HowTo This is the top-level VI of a DQMH Singleton module. See the following video for a walkthrough of this VI's functionality: https://bit.ly/DQMHMainWalkthrough"
  # "Note: Do not modify or remove the \"DQMH\" labels on objects. These labels are used by the Tools > DQMH Consortium > DQMH utilities."
  # "Update the Module Admin to ensure this module can run as a stand alone next time."
  n1 = call "Init Module.vi"("Singleton Module Admin in"="Module Admin") -> ("error out"=w17:errorcluster, "Scripting Server Request Events"=w6:T2, "Singleton Module Admin out"=w9:refnum<class "Delacor_lib_QMH_Module Admin.lvclass">)  [unwired: 8 in]
  n2 = register-events "DQMH_REG_EVENTS"(w6, T1 {"onError"=refnum, "onRpc"=refnum} ("MCP Events")) -> (reference out=w7:refnum<event-registration>, error out=w10:errorcluster)  [unwired: 2 in]
  n3 = call <vilib>:"Delacor_lib_QMH_Create Message Queue.vi"("error in"=w17) -> ("error out"=w12:errorcluster, "Message Queue"=w5:refnum<class "Delacor_lib_QMH_Message Queue.lvclass">)  [unwired: 9 in]
  n4 = Merge Errors(w12, w10) -> (w11:errorcluster)
  n5 = case shown="No Error" w11 {
    selector: w11 -> [w24 w943]
    tunnel: [w26 w942] -> w18
    tunnel: [w23 w941] -> w8
    tunnel: w7 -> [w21 w941]
    tunnel: w5 -> [w20 w936]
    tunnel: [w25 _] -> w15
    tunnel: w9 -> [w19 w937]
    frame No Error {
      n6 = while {
        tunnel: w20 -> [w27]
        shift-right: [w30] -> w23
        shift-left: w21 -> [w31]
        tunnel: [w32] -> w25
        tunnel: w19 -> [w28]
        stop <- w29 stop-if-true
        # "Event Handling Loop"
        n7 = event "DQMH_EVENT_MAIN" shown="[44] <Scripting Server Request Events.Get Library>: User Event" {
          selector: w31 -> [_ _ _ _ _ _ _ _ _ _ _ _ _ _ _ _ _ _ _ _ _ _ _ _ _ _ _ _ _ _ _ _ _ _ _ _ _ w327 _ _ _ _ _ _ _]
          dyn-events: [_ _ _ _ _ _ _ _ _ _ _ _ _ _ _ _ _ _ _ _ _ _ _ _ _ _ _ _ _ _ _ _ _ _ _ _ _ w326 _ _ _ _ _ _ _] -> w30
          timeout: _ -> [_ _ _ _ _ _ _ _ _ _ _ _ _ _ _ _ _ _ _ _ _ _ _ _ _ _ _ _ _ _ _ _ _ _ _ _ _ _ _ _ _ _ _ _ _]
          tunnel: [_ _ _ _ _ _ TRUE ("Discard?") _ _ _ _ _ _ _ _ _ _ _ _ _ _ _ _ _ _ _ _ _ _ _ _ _ _ _ _ _ _ _ _ _ _ _ _ _ _] -> w29
          tunnel: w27 -> [_ w41 _ _ _ _ w65 w72 _ w91 w102 w114 w122 w130 w138 w148 w157 w166 w174 w183 w192 w202 w211 w219 w228 w237 w246 w255 w263 w271 w280 w288 w294 w301 w309 w315 w323 _ w334 w341 w348 w355 w363 w371 w379]
          tunnel: [w39 w42 _ _ w48 _ w68 w74 w83 w84 w96 w103 w115 w123 w131 w139 w149 w159 w168 w175 w184 w194 w203 w212 w220 w229 w238 w247 w256 w264 w272 w281 w289 w295 w302 w310 w316 w325 w328 w335 w342 w349 w356 w364 w372] -> w33
          tunnel: w28 -> [_ _ _ _ _ _ _ w71 _ _ _ _ _ _ _ _ _ _ _ _ _ _ _ _ _ _ _ _ _ _ _ _ _ _ _ _ _ _ _ _ _ _ _ _ _]
          event "Simulate EHL Error": Value Change {
            # "#DQMH_HowTo The 'Simulate EHL Error' button  illustrates how the EHL handles errors. This event is instructional in nature and can be removed."
            # "This case simulates an error being generated by the EHL"
            n8 = event-data() -> ()  [unwired: 1 in, 1 out]
            n9 = call "Module Name--constant.vi"() -> ("Module Name"=w36:string)  [unwired: 11 in]
            n10 = Format Into String(format string="Simulated error originating at Event Handling Loop in %s", w36) -> (resulting string=w37:string)  [unwired: 2 in, 1 out]
            n11 = call <vilib>:"Error Cluster From Error Code.vi"("show call chain? (False)"=TRUE, "error message (\"\")"=w37, "error code (0)"=5000) -> ("error out"=w39:errorcluster)  [unwired: 6 in]
          }
          event "Simulate MHL Error": Value Change {
            # "#DQMH_HowTo The 'Simulate MHL Error' button  illustrates how the MHL handles errors. This event is instructional in nature and can be removed."
            # "This case simulates an error being generated by the MHL"
            n12 = event-data() -> ()  [unwired: 1 in, 1 out]
            n13 = call-poly <vilib>:"Delacor_lib_QMH_Enqueue Message (poly).vi"("Message"="Simulate MHL Error", "Message Queue in"=w41) -> ("error out"=w42:errorcluster)  [unwired: 8 in, 1 out]
          }
          event User Event {
            # "Show the panel of this VI, and send a status updated message to let listeners know."
            # "Another Module called the \"Show Panel\" API Method."
            n14 = event-data() -> ()  [unwired: 1 in, 1 out]
            n15 = control-ref of="This VI"() -> (w44:refnum<vi>)
            n16 = call "Open VI Panel.vi"("VI"=w44) -> ()  [unwired: 10 in, 1 out]
            n17 = call "Status Updated.vi"("Status"="Panel shown." ("format string")) -> ()  [unwired: 10 in, 1 out]
          }
          event User Event {
            # "Hide the panel of this VI, and send a status updated message to let listeners know."
            # "Another Module called the \"Hide Panel\" API Method."
            n18 = event-data() -> ()  [unwired: 1 in, 1 out]
            n19 = control-ref of="This VI"() -> (w46:refnum<vi>)
            n20 = call "Hide VI Panel.vi"("VI"=w46) -> ()  [unwired: 10 in, 1 out]
            n21 = call "Status Updated.vi"("Status"="Panel hidden." ("format string")) -> ()  [unwired: 10 in, 1 out]
          }
          event User Event {
            # "Another Module called the \"Get Module Execution Status\" API Method."
            n22 = event-data() -> ()  [unwired: 1 in, 1 out]
            n23 = call "Update Module Execution Status.vi"("Running?"=TRUE) -> ("error out"=w48:errorcluster)  [unwired: 10 in]
          }
          event User Event {
            # "Another Module called the \"Show Diagram\" API Method. This event is used for debugging."
            n24 = event-data() -> ()  [unwired: 1 in, 1 out]
            n25 = disable-structure shown="RUN_TIME_ENGINE==False" {
              frame condition #0 (active) {
                # "functionality not available in exe"
                n26 = invoke on="Invoke Node" class="VI" method="Lock State.Get"() -> (error out=w54:errorcluster, "Get Lock State"=w53:T5, "pwd in cache"=w50:bool)  [unwired: 4 in, 1 out]
                n27 = Equal?(x=T5."Password-protected", y=w53) -> (x = y?=w51:bool)
                n28 = Compound Arithmetic op=AND(w51, invert w50) -> (w49:bool)
                n29 = case shown="False" w49 {
                  tunnel: w54 -> [w57 _]
                  frame False {
                    n30 = property on="Property Node" class="VI"(error in=w57, "BDWin.Open"=TRUE ("Block Diagram Window:Open")) -> ()  [unwired: 1 in, 2 out]
                    n31 = call "Status Updated.vi"("Status"="Block Diagram shown." ("format string")) -> ()  [unwired: 10 in, 1 out]
                  }
                  frame True {
                    # "Password-protected VI, and the password is not in the cache. Do not show the diagram."
                  }
                }
              }
              frame condition #1 {
              }
            }
          }
          event User Event {
            # "The Stop Module Event can get fired from the Exit message in the MHL. The queue gets destroyed in that case. If the queue no longer exists, the Enqueue Exit as a priority message will return error 1. It is safe to ignore, because the module is already exiting."
            # "Another Module called the \"Stop Module\" API Method  or the Message Handling Loop below."
            n32 = event-data() -> ("Origin"=w64:string, "Exit via Stop Module Req?"=w60:bool, "Wait for Module to stop?"=w59:bool)  [unwired: 1 in]
            n33 = local write "Status"(w64) -> ()
            n34 = Bundle By Name(cluster=T6 {"Origin"="", "Exit via Stop Module Req?"=FALSE, "Wait for Module to stop?"=FALSE} ("Stop Argument"), "Exit via Stop Module Req?"=w60, "Wait for Module to stop?"=w59) -> (w58:T6)
            n35 = call-poly <vilib>:"Delacor_lib_QMH_Enqueue Message (poly).vi"("Priority Message? (F)"=TRUE, "Message Data"=w58, "Message"="Exit", "Message Queue in"=w65) -> ("error out"=w69:errorcluster)  [unwired: 6 in, 1 out]
            n36 = call <vilib>:"Clear Errors.vi"("error in (no error)"=w69, "specific error code to clear (0: all)"=1) -> ("error out"=w68:errorcluster)  [unwired: 4 in, 1 out]
          }
          event Panel Close? {
            w73 = TRUE  # Discard the event, the MHL is responsible for closing and stopping this VI.
            # "Hide the panel or send the 'Exit' message if the user clicks the 'X' on the module main VI panel."
            n37 = event-data() -> ()  [unwired: 1 in, 1 out]
            n38 = property on="Property Node" class="Module Admin"(reference=w71) -> ("Accessors:External Launch"=w70:bool)  [unwired: 1 in, 2 out]
            n39 = case shown="True" w70 {
              tunnel: w72 -> [_ w80]
              tunnel: [_ w81] -> w74
              frame True {
                # "If externally launched, clicking the 'X' hides the panel, but doesn't close it."
                n40 = control-ref of="This VI"() -> (w77:refnum<vi>)
                n41 = call "Hide VI Panel.vi"("VI"=w77) -> ("error out"=w75:errorcluster)  [unwired: 10 in]
                n42 = call "Status Updated.vi"("error in"=w75, "Status"="Panel hidden." ("format string")) -> ()  [unwired: 9 in, 1 out]
              }
              frame False {
                # "If run as a stand-alone VI, clicking the panel 'X' stops the VI."
                n43 = call-poly <vilib>:"Delacor_lib_QMH_Enqueue Message (poly).vi"("Priority Message? (F)"=TRUE, "Message"="Exit", "Message Queue in"=w80) -> ("error out"=w81:errorcluster)  [unwired: 7 in, 1 out]
              }
            }
            n44 = event-data ("Event Filter Node")("Discard?"=w73) -> ()  [unwired: 1 in, 1 out]
          }
          event Application Instance Close {
            n45 = event-data() -> ()  [unwired: 1 in, 1 out]
            n46 = call "Stop Module.vi"("Origin"="Application Instance Close") -> ("error out"=w83:errorcluster)  [unwired: 10 in]
          }
          event User Event {
            # "Another Module called the \"New VI\" API Method."
            n47 = event-data() -> ("Open Frontpanel"=w87:bool, "Wait Notifier"=w86:refnum<notifier>, "wait for reply"=w85:bool)  [unwired: 1 in]
            n48 = Bundle(cluster=T7 {"Open Frontpanel"=TRUE, "Wait Notifier"=refnum, "wait for reply"=FALSE} ("New VI Argument"), "Open Frontpanel"=w87, "Wait Notifier"=w86, "wait for reply"=w85) -> (w88:T7)
            n49 = call-poly <vilib>:"Delacor_lib_QMH_Enqueue Message (poly).vi"("Message Data"=w88, "Message"="New VI", "Message Queue in"=w91) -> ("error out"=w84:errorcluster)  [unwired: 7 in, 1 out]
          }
          event User Event {
            # "Another Module called the \"Add Object\" API Method."
            n50 = event-data() -> ("VI Reference"=w98:i32, "Object Name"=w97:string, "Wait Notifier"=w95:refnum<notifier>, "wait for reply"=w94:bool, "position_x"=w93:i32, "position_y"=w92:i32)  [unwired: 1 in]
            n51 = Bundle(cluster=T8 {"VI Reference"=0, "Object Name"="", "Wait Notifier"=refnum, "wait for reply"=FALSE, "position_x"=0, "position_y"=0} ("Add Object Argument"), "VI Reference"=w98, "Object Name"=w97, "Wait Notifier"=w95, "wait for reply"=w94, "position_x"=w93, "position_y"=w92) -> (w99:T8)
            n52 = call-poly <vilib>:"Delacor_lib_QMH_Enqueue Message (poly).vi"("Message Data"=w99, "Message"="Add Object", "Message Queue in"=w102) -> ("error out"=w96:errorcluster)  [unwired: 7 in, 1 out]
          }
          event User Event {
            # "Another Module called the \"Connect Objects\" API Method."
            n53 = event-data() -> ("vi reference"=w110:i32, "from object reference"=w109:i32, "to object reference"=w108:i32, "from object terminal index"=w107:i32, "to object terminal index"=w106:i32, "Wait Notifier"=w105:refnum<notifier>, "wait for reply"=w104:bool)  [unwired: 1 in]
            n54 = Bundle(cluster=T9 {"vi reference"=0, "from object reference"=0, "to object reference"=0, "from object terminal index"=0, "to object terminal index"=0, "Wait Notifier"=refnum, "wait for reply"=FALSE} ("Connect Objects Argument"), "vi reference"=w110, "from object reference"=w109, "to object reference"=w108, "from object terminal index"=w107, "to object terminal index"=w106, "Wait Notifier"=w105, "wait for reply"=w104) -> (w111:T9)
            n55 = call-poly <vilib>:"Delacor_lib_QMH_Enqueue Message (poly).vi"("Message Data"=w111, "Message"="Connect Objects", "Message Queue in"=w114) -> ("error out"=w103:errorcluster)  [unwired: 7 in, 1 out]
          }
          event User Event {
            # "Another Module called the \"Get Object Terminals\" API Method."
            n56 = event-data() -> ("object id"=w118:i32, "Wait Notifier"=w117:refnum<notifier>, "wait for reply"=w116:bool)  [unwired: 1 in]
            n57 = Bundle(cluster=T10 {"object id"=0, "Wait Notifier"=refnum, "wait for reply"=FALSE} ("Get Object Terminals Argument"), "object id"=w118, "Wait Notifier"=w117, "wait for reply"=w116) -> (w119:T10)
            n58 = call-poly <vilib>:"Delacor_lib_QMH_Enqueue Message (poly).vi"("Message Data"=w119, "Message"="Get Object Terminals", "Message Queue in"=w122) -> ("error out"=w115:errorcluster)  [unwired: 7 in, 1 out]
          }
          event User Event {
            # "Another Module called the \"get vi error list\" API Method."
            n59 = event-data() -> ("vi id"=w126:i32, "Wait Notifier"=w125:refnum<notifier>, "wait for reply"=w124:bool)  [unwired: 1 in]
            n60 = Bundle(cluster=T11 {"vi id"=0, "Wait Notifier"=refnum, "wait for reply"=FALSE} ("get vi error list Argument"), "vi id"=w126, "Wait Notifier"=w125, "wait for reply"=w124) -> (w127:T11)
            n61 = call-poly <vilib>:"Delacor_lib_QMH_Enqueue Message (poly).vi"("Message Data"=w127, "Message"="get vi error list", "Message Queue in"=w130) -> ("error out"=w123:errorcluster)  [unwired: 7 in, 1 out]
          }
          event User Event {
            # "Another Module called the \"Cleanup VI\" API Method."
            n62 = event-data() -> ("vi reference"=w134:i32, "Wait Notifier"=w133:refnum<notifier>, "wait for reply"=w132:bool)  [unwired: 1 in]
            n63 = Bundle(cluster=T12 {"vi reference"=0, "Wait Notifier"=refnum, "wait for reply"=FALSE} ("Cleanup VI Argument"), "vi reference"=w134, "Wait Notifier"=w133, "wait for reply"=w132) -> (w135:T12)
            n64 = call-poly <vilib>:"Delacor_lib_QMH_Enqueue Message (poly).vi"("Message Data"=w135, "Message"="Cleanup VI", "Message Queue in"=w138) -> ("error out"=w131:errorcluster)  [unwired: 7 in, 1 out]
          }
          event User Event {
            # "Another Module called the \"create_control\" API Method."
            n65 = event-data() -> ("Object ID"=w144:i32, "Terminal Index"=w143:i32, "Constant"=w142:bool, "Wait Notifier"=w141:refnum<notifier>, "wait for reply"=w140:bool)  [unwired: 1 in]
            n66 = Bundle(cluster=T13 {"Object ID"=0, "Terminal Index"=0, "Constant"=FALSE, "Wait Notifier"=refnum, "wait for reply"=FALSE, "Value"=""} ("create_control Argument"), "Object ID"=w144, "Terminal Index"=w143, "Constant"=w142, "Wait Notifier"=w141, "wait for reply"=w140) -> (w145:T13)  [unwired: 1 in]
            n67 = call-poly <vilib>:"Delacor_lib_QMH_Enqueue Message (poly).vi"("Message Data"=w145, "Message"="create_control", "Message Queue in"=w148) -> ("error out"=w139:errorcluster)  [unwired: 7 in, 1 out]
          }
          event User Event {
            # "Another Module called the \"Run VI\" API Method."
            n68 = event-data() -> ("VI ID"=w153:i32, "open_frontpanel"=w152:bool, "Wait Notifier"=w151:refnum<notifier>, "wait for reply"=w150:bool)  [unwired: 1 in]
            n69 = Bundle(cluster=T14 {"VI ID"=0, "open_frontpanel"=FALSE, "Wait Notifier"=refnum, "wait for reply"=FALSE} ("Run VI Argument"), "VI ID"=w153, "open_frontpanel"=w152, "Wait Notifier"=w151, "wait for reply"=w150) -> (w154:T14)
            n70 = call-poly <vilib>:"Delacor_lib_QMH_Enqueue Message (poly).vi"("Message Data"=w154, "Message"="Run VI", "Message Queue in"=w157) -> ("error out"=w149:errorcluster)  [unwired: 7 in, 1 out]
          }
          event User Event {
            # "Another Module called the \"add_to_selection\" API Method."
            n71 = event-data() -> ("object_id"=w162:i32, "Wait Notifier"=w161:refnum<notifier>, "wait for reply"=w160:bool, "vi_id"=w158:i32)  [unwired: 1 in]
            n72 = Bundle(cluster=T15 {"object_id"=0, "Wait Notifier"=refnum, "wait for reply"=FALSE, "vi_id"=0} ("add_to_selection Argument"), "object_id"=w162, "Wait Notifier"=w161, "wait for reply"=w160, "vi_id"=w158) -> (w163:T15)
            n73 = call-poly <vilib>:"Delacor_lib_QMH_Enqueue Message (poly).vi"("Message Data"=w163, "Message"="add_to_selection", "Message Queue in"=w166) -> ("error out"=w159:errorcluster)  [unwired: 7 in, 1 out]
          }
          event User Event {
            # "Another Module called the \"clear_selection_list\" API Method."
            n74 = event-data() -> ("Wait Notifier"=w170:refnum<notifier>, "wait for reply"=w169:bool, "vi_id"=w167:i32)  [unwired: 1 in]
            n75 = Bundle(cluster=T16 {"Wait Notifier"=refnum, "wait for reply"=FALSE, "vi_id"=0} ("clear_selection_list Argument"), "Wait Notifier"=w170, "wait for reply"=w169, "vi_id"=w167) -> (w171:T16)
            n76 = call-poly <vilib>:"Delacor_lib_QMH_Enqueue Message (poly).vi"("Message Data"=w171, "Message"="clear_selection_list", "Message Queue in"=w174) -> ("error out"=w168:errorcluster)  [unwired: 7 in, 1 out]
          }
          event User Event {
            # "Another Module called the \"remove_from_selection\" API Method."
            n77 = event-data() -> ("vi_id"=w179:i32, "object_id"=w178:i32, "Wait Notifier"=w177:refnum<notifier>, "wait for reply"=w176:bool)  [unwired: 1 in]
            n78 = Bundle(cluster=T17 {"vi_id"=0, "object_id"=0, "Wait Notifier"=refnum, "wait for reply"=FALSE} ("remove_from_selection Argument"), "vi_id"=w179, "object_id"=w178, "Wait Notifier"=w177, "wait for reply"=w176) -> (w180:T17)
            n79 = call-poly <vilib>:"Delacor_lib_QMH_Enqueue Message (poly).vi"("Message Data"=w180, "Message"="remove_from_selection", "Message Queue in"=w183) -> ("error out"=w175:errorcluster)  [unwired: 7 in, 1 out]
          }
          event User Event {
            # "Another Module called the \"enclose_selection\" API Method."
            n80 = event-data() -> ("vi_id"=w188:i32, "structure_type"=w187:string, "Wait Notifier"=w186:refnum<notifier>, "wait for reply"=w185:bool)  [unwired: 1 in]
            n81 = Bundle(cluster=T18 {"vi_id"=0, "structure_type"="", "Wait Notifier"=refnum, "wait for reply"=FALSE} ("enclose_selection Argument"), "vi_id"=w188, "structure_type"=w187, "Wait Notifier"=w186, "wait for reply"=w185) -> (w189:T18)
            n82 = call-poly <vilib>:"Delacor_lib_QMH_Enqueue Message (poly).vi"("Message Data"=w189, "Message"="enclose_selection", "Message Queue in"=w192) -> ("error out"=w184:errorcluster)  [unwired: 7 in, 1 out]
          }
          event User Event {
            # "Another Module called the \"rename_object\" API Method."
            n83 = event-data() -> ("new_label_name"=w198:string, "label_visible"=w197:bool, "Wait Notifier"=w196:refnum<notifier>, "wait for reply"=w195:bool, "object_id"=w193:i32)  [unwired: 1 in]
            n84 = Bundle(cluster=T19 {"new_label_name"="", "label_visible"=FALSE, "Wait Notifier"=refnum, "wait for reply"=FALSE, "object_id"=0} ("rename_object Argument"), "new_label_name"=w198, "label_visible"=w197, "Wait Notifier"=w196, "wait for reply"=w195, "object_id"=w193) -> (w199:T19)
            n85 = call-poly <vilib>:"Delacor_lib_QMH_Enqueue Message (poly).vi"("Message Data"=w199, "Message"="rename_object", "Message Queue in"=w202) -> ("error out"=w194:errorcluster)  [unwired: 7 in, 1 out]
          }
          event User Event {
            # "Another Module called the \"set_value\" API Method."
            n86 = event-data() -> ("object_id"=w207:i32, "value"=w206:string, "Wait Notifier"=w205:refnum<notifier>, "wait for reply"=w204:bool)  [unwired: 1 in]
            n87 = Bundle(cluster=T20 {"object_id"=0, "value"="", "Wait Notifier"=refnum, "wait for reply"=FALSE} ("set_value Argument"), "object_id"=w207, "value"=w206, "Wait Notifier"=w205, "wait for reply"=w204) -> (w208:T20)
            n88 = call-poly <vilib>:"Delacor_lib_QMH_Enqueue Message (poly).vi"("Message Data"=w208, "Message"="set_value", "Message Queue in"=w211) -> ("error out"=w203:errorcluster)  [unwired: 7 in, 1 out]
          }
          event User Event {
            # "Another Module called the \"delete_object\" API Method."
            n89 = event-data() -> ("object_id"=w215:i32, "Wait Notifier"=w214:refnum<notifier>, "wait for reply"=w213:bool)  [unwired: 1 in]
            n90 = Bundle(cluster=T21 {"object_id"=0, "Wait Notifier"=refnum, "wait for reply"=FALSE} ("delete_object Argument"), "object_id"=w215, "Wait Notifier"=w214, "wait for reply"=w213) -> (w216:T21)
            n91 = call-poly <vilib>:"Delacor_lib_QMH_Enqueue Message (poly).vi"("Message Data"=w216, "Message"="delete_object", "Message Queue in"=w219) -> ("error out"=w212:errorcluster)  [unwired: 7 in, 1 out]
          }
          event User Event {
            # "Another Module called the \"save_vi\" API Method."
            n92 = event-data() -> ("vi_id"=w224:i32, "path"=w223:string, "Wait Notifier"=w222:refnum<notifier>, "wait for reply"=w221:bool)  [unwired: 1 in]
            n93 = Bundle(cluster=T22 {"vi_id"=0, "path"="", "Wait Notifier"=refnum, "wait for reply"=FALSE} ("save_vi Argument"), "vi_id"=w224, "path"=w223, "Wait Notifier"=w222, "wait for reply"=w221) -> (w225:T22)
            n94 = call-poly <vilib>:"Delacor_lib_QMH_Enqueue Message (poly).vi"("Message Data"=w225, "Message"="save_vi", "Message Queue in"=w228) -> ("error out"=w220:errorcluster)  [unwired: 7 in, 1 out]
          }
          event User Event {
            # "Another Module called the \"get_structure_diagram\" API Method."
            n95 = event-data() -> ("structure_id"=w233:i32, "index"=w232:i32, "Wait Notifier"=w231:refnum<notifier>, "wait for reply"=w230:bool)  [unwired: 1 in]
            n96 = Bundle(cluster=T23 {"structure_id"=0, "index"=0, "Wait Notifier"=refnum, "wait for reply"=FALSE} ("get_structure_diagram Argument"), "structure_id"=w233, "index"=w232, "Wait Notifier"=w231, "wait for reply"=w230) -> (w234:T23)
            n97 = call-poly <vilib>:"Delacor_lib_QMH_Enqueue Message (poly).vi"("Message Data"=w234, "Message"="get_structure_diagram", "Message Queue in"=w237) -> ("error out"=w229:errorcluster)  [unwired: 7 in, 1 out]
          }
          event User Event {
            # "Another Module called the \"add_subvi\" API Method."
            n98 = event-data() -> ("diagram_id"=w242:i32, "subvi_path"=w241:string, "Wait Notifier"=w240:refnum<notifier>, "wait for reply"=w239:bool)  [unwired: 1 in]
            n99 = Bundle(cluster=T24 {"diagram_id"=0, "subvi_path"="", "Wait Notifier"=refnum, "wait for reply"=FALSE, "position_x"=0, "position_y"=0} ("add_subvi Argument"), "diagram_id"=w242, "subvi_path"=w241, "Wait Notifier"=w240, "wait for reply"=w239) -> (w243:T24)  [unwired: 2 in]
            n100 = call-poly <vilib>:"Delacor_lib_QMH_Enqueue Message (poly).vi"("Message Data"=w243, "Message"="add_subvi", "Message Queue in"=w246) -> ("error out"=w238:errorcluster)  [unwired: 7 in, 1 out]
          }
          event User Event {
            # "Another Module called the \"connect_to_pane\" API Method."
            n101 = event-data() -> ("control_id"=w251:i32, "connector_pane_index"=w250:i32, "Wait Notifier"=w249:refnum<notifier>, "wait for reply"=w248:bool)  [unwired: 1 in]
            n102 = Bundle(cluster=T25 {"control_id"=0, "connector_pane_index"=0, "Wait Notifier"=refnum, "wait for reply"=FALSE} ("connect_to_pane Argument"), "control_id"=w251, "connector_pane_index"=w250, "Wait Notifier"=w249, "wait for reply"=w248) -> (w252:T25)
            n103 = call-poly <vilib>:"Delacor_lib_QMH_Enqueue Message (poly).vi"("Message Data"=w252, "Message"="connect_to_pane", "Message Queue in"=w255) -> ("error out"=w247:errorcluster)  [unwired: 7 in, 1 out]
          }
          event User Event {
            # "Another Module called the \"get_object_help\" API Method."
            n104 = event-data() -> ("object_id"=w259:i32, "Wait Notifier"=w258:refnum<notifier>, "wait for reply"=w257:bool)  [unwired: 1 in]
            n105 = Bundle(cluster=T26 {"object_id"=0, "Wait Notifier"=refnum, "wait for reply"=FALSE} ("get_object_help Argument"), "object_id"=w259, "Wait Notifier"=w258, "wait for reply"=w257) -> (w260:T26)
            n106 = call-poly <vilib>:"Delacor_lib_QMH_Enqueue Message (poly).vi"("Message Data"=w260, "Message"="get_object_help", "Message Queue in"=w263) -> ("error out"=w256:errorcluster)  [unwired: 7 in, 1 out]
          }
          event User Event {
            # "Another Module called the \"get_loop_conditional_terminal\" API Method."
            n107 = event-data() -> ("loop_id"=w267:i32, "Wait Notifier"=w266:refnum<notifier>, "wait for reply"=w265:bool)  [unwired: 1 in]
            n108 = Bundle(cluster=T27 {"loop_id"=0, "Wait Notifier"=refnum, "wait for reply"=FALSE} ("get_loop_conditional_terminal Argument"), "loop_id"=w267, "Wait Notifier"=w266, "wait for reply"=w265) -> (w268:T27)
            n109 = call-poly <vilib>:"Delacor_lib_QMH_Enqueue Message (poly).vi"("Message Data"=w268, "Message"="get_loop_conditional_terminal", "Message Queue in"=w271) -> ("error out"=w264:errorcluster)  [unwired: 7 in, 1 out]
          }
          event User Event {
            # "Another Module called the \"show_conditional_terminal\" API Method."
            n110 = event-data() -> ("loop_id"=w276:i32, "show"=w275:bool, "Wait Notifier"=w274:refnum<notifier>, "wait for reply"=w273:bool)  [unwired: 1 in]
            n111 = Bundle(cluster=T28 {"loop_id"=0, "show"=FALSE, "Wait Notifier"=refnum, "wait for reply"=FALSE} ("show_conditional_terminal Argument"), "loop_id"=w276, "show"=w275, "Wait Notifier"=w274, "wait for reply"=w273) -> (w277:T28)
            n112 = call-poly <vilib>:"Delacor_lib_QMH_Enqueue Message (poly).vi"("Message Data"=w277, "Message"="show_conditional_terminal", "Message Queue in"=w280) -> ("error out"=w272:errorcluster)  [unwired: 7 in, 1 out]
          }
          event User Event {
            # "Another Module called the \"get_loop_iteration_terminal\" API Method."
            n113 = event-data() -> ("loop_id"=w284:i32, "Wait Notifier"=w283:refnum<notifier>, "wait for reply"=w282:bool)  [unwired: 1 in]
            n114 = Bundle(cluster=T29 {"loop_id"=0, "Wait Notifier"=refnum, "wait for reply"=FALSE} ("get_loop_iteration_terminal Argument"), "loop_id"=w284, "Wait Notifier"=w283, "wait for reply"=w282) -> (w285:T29)
            n115 = call-poly <vilib>:"Delacor_lib_QMH_Enqueue Message (poly).vi"("Message Data"=w285, "Message"="get_loop_iteration_terminal", "Message Queue in"=w288) -> ("error out"=w281:errorcluster)  [unwired: 7 in, 1 out]
          }
          event User Event {
            # "Another Module called the \"Read Config Data\" API Method."
            n116 = event-data() -> ("Boolean"=w290:bool)  [unwired: 1 in]
            n117 = Bundle(cluster=T30 {"Boolean"=FALSE} ("Read Config Data Argument"), "Boolean"=w290) -> (w291:T30)
            n118 = call-poly <vilib>:"Delacor_lib_QMH_Enqueue Message (poly).vi"("Message Data"=w291, "Message"="Read Config Data", "Message Queue in"=w294) -> ("error out"=w289:errorcluster)  [unwired: 7 in, 1 out]
          }
          event User Event {
            # "Another Module called the \"get_allowed_paths\" API Method."
            n119 = event-data() -> ("Wait Notifier"=w297:refnum<notifier>, "wait for reply"=w296:bool)  [unwired: 1 in]
            n120 = Bundle(cluster=T31 {"Wait Notifier"=refnum, "wait for reply"=FALSE} ("get_allowed_paths Argument"), "Wait Notifier"=w297, "wait for reply"=w296) -> (w298:T31)
            n121 = call-poly <vilib>:"Delacor_lib_QMH_Enqueue Message (poly).vi"("Message Data"=w298, "Message"="get_allowed_paths", "Message Queue in"=w301) -> ("error out"=w295:errorcluster)  [unwired: 7 in, 1 out]
          }
          event User Event {
            # "Another Module called the \"create_project\" API Method."
            n122 = event-data() -> ("File Path"=w305:string, "Wait Notifier"=w304:refnum<notifier>, "wait for reply"=w303:bool)  [unwired: 1 in]
            n123 = Bundle(cluster=T32 {"File Path"="", "Wait Notifier"=refnum, "wait for reply"=FALSE} ("create_project Argument"), "File Path"=w305, "Wait Notifier"=w304, "wait for reply"=w303) -> (w306:T32)
            n124 = call-poly <vilib>:"Delacor_lib_QMH_Enqueue Message (poly).vi"("Message Data"=w306, "Message"="create_project", "Message Queue in"=w309) -> ("error out"=w302:errorcluster)  [unwired: 7 in, 1 out]
          }
          event User Event {
            # "Another Module called the \"Set Allowed Paths\" API Method."
            n125 = event-data() -> ("Working Directory Folder Path"=w311:path[])  [unwired: 1 in]
            n126 = Bundle(cluster=T33 {"Working Directory Folder Path"=[]} ("Set Working Directory Argument"), "Working Directory Folder Path"=w311) -> (w312:T33)
            n127 = call-poly <vilib>:"Delacor_lib_QMH_Enqueue Message (poly).vi"("Message Data"=w312, "Message"="Set Working Directory", "Message Queue in"=w315) -> ("error out"=w310:errorcluster)  [unwired: 7 in, 1 out]
          }
          event User Event {
            # "Another Module called the \"open_vi\" API Method."
            n128 = event-data() -> ("vi_path"=w319:string, "Wait Notifier"=w318:refnum<notifier>, "wait for reply"=w317:bool)  [unwired: 1 in]
            n129 = Bundle(cluster=T34 {"vi_path"="", "Wait Notifier"=refnum, "wait for reply"=FALSE} ("open_vi Argument"), "vi_path"=w319, "Wait Notifier"=w318, "wait for reply"=w317) -> (w320:T34)
            n130 = call-poly <vilib>:"Delacor_lib_QMH_Enqueue Message (poly).vi"("Message Data"=w320, "Message"="open_vi", "Message Queue in"=w323) -> ("error out"=w316:errorcluster)  [unwired: 7 in, 1 out]
          }
          event User Event {
            # "This module called the \"Private.Register MCP Events\" private request."
            n131 = event-data() -> ("MCP Events"=w324:T1)  [unwired: 1 in]
            n132 = register-events(reference=w327, w324) -> (reference out=w326:refnum<event-registration>, error out=w325:errorcluster)  [unwired: 2 in]
          }
          event User Event {
            # "Another Module called the \"New MCP RPC Message\" API Method."
            n133 = event-data() -> ("request"=w330:string, "response"=w329:string)  [unwired: 1 in]
            n134 = Bundle(cluster=T35 {"request"="", "response"=""} ("New MCP RPC Message Argument"), "request"=w330, "response"=w329) -> (w331:T35)
            n135 = call-poly <vilib>:"Delacor_lib_QMH_Enqueue Message (poly).vi"("Message Data"=w331, "Message"="New MCP RPC Message", "Message Queue in"=w334) -> ("error out"=w328:errorcluster)  [unwired: 7 in, 1 out]
          }
          event User Event {
            # "Another Module called the \"New MCP RPC Message\" API Method."
            n136 = event-data() -> ("request"=w337:string, "response"=w336:string)  [unwired: 1 in]
            n137 = Bundle(cluster=T35 {"request"="", "response"=""} ("New MCP RPC Message Argument"), "request"=w337, "response"=w336) -> (w338:T35)
            n138 = call-poly <vilib>:"Delacor_lib_QMH_Enqueue Message (poly).vi"("Message Data"=w338, "Message"="New MCP RPC Message", "Message Queue in"=w341) -> ("error out"=w335:errorcluster)  [unwired: 7 in, 1 out]
          }
          event User Event {
            # "Another Module called the \"get-available-objects\" API Method."
            n139 = event-data() -> ("Wait Notifier"=w344:refnum<notifier>, "wait for reply"=w343:bool)  [unwired: 1 in]
            n140 = Bundle(cluster=T36 {"Wait Notifier"=refnum, "wait for reply"=FALSE} ("get-available-objects Argument"), "Wait Notifier"=w344, "wait for reply"=w343) -> (w345:T36)
            n141 = call-poly <vilib>:"Delacor_lib_QMH_Enqueue Message (poly).vi"("Message Data"=w345, "Message"="get-available-objects", "Message Queue in"=w348) -> ("error out"=w342:errorcluster)  [unwired: 7 in, 1 out]
          }
          event User Event {
            # "Another Module called the \"Get open VIs\" API Method."
            n142 = event-data() -> ("Wait Notifier"=w351:refnum<notifier>, "wait for reply"=w350:bool)  [unwired: 1 in]
            n143 = Bundle(cluster=T37 {"Wait Notifier"=refnum, "wait for reply"=FALSE} ("Get open VIs Argument"), "Wait Notifier"=w351, "wait for reply"=w350) -> (w352:T37)
            n144 = call-poly <vilib>:"Delacor_lib_QMH_Enqueue Message (poly).vi"("Message Data"=w352, "Message"="Get open VIs", "Message Queue in"=w355) -> ("error out"=w349:errorcluster)  [unwired: 7 in, 1 out]
          }
          event User Event {
            # "Another Module called the \"Get VI Blockdiagram\" API Method."
            n145 = event-data() -> ("VI ID"=w359:i32, "Wait Notifier"=w358:refnum<notifier>, "wait for reply"=w357:bool)  [unwired: 1 in]
            n146 = Bundle(cluster=T38 {"VI ID"=0, "Wait Notifier"=refnum, "wait for reply"=FALSE} ("Get VI Blockdiagram Argument"), "VI ID"=w359, "Wait Notifier"=w358, "wait for reply"=w357) -> (w360:T38)
            n147 = call-poly <vilib>:"Delacor_lib_QMH_Enqueue Message (poly).vi"("Message Data"=w360, "Message"="Get VI Blockdiagram", "Message Queue in"=w363) -> ("error out"=w356:errorcluster)  [unwired: 7 in, 1 out]
          }
          event User Event {
            # "Another Module called the \"Get VI Frontpanel Picture\" API Method."
            n148 = event-data() -> ("VI ID"=w367:i32, "Wait Notifier"=w366:refnum<notifier>, "wait for reply"=w365:bool)  [unwired: 1 in]
            n149 = Bundle(cluster=T39 {"VI ID"=0, "Wait Notifier"=refnum, "wait for reply"=FALSE} ("Get VI Frontpanel Picture Argument"), "VI ID"=w367, "Wait Notifier"=w366, "wait for reply"=w365) -> (w368:T39)
            n150 = call-poly <vilib>:"Delacor_lib_QMH_Enqueue Message (poly).vi"("Message Data"=w368, "Message"="Get VI Frontpanel Picture", "Message Queue in"=w371) -> ("error out"=w364:errorcluster)  [unwired: 7 in, 1 out]
          }
          event User Event {
            # "Another Module called the \"Get Library\" API Method."
            n151 = event-data() -> ("Library Path"=w375:string, "Wait Notifier"=w374:refnum<notifier>, "wait for reply"=w373:bool)  [unwired: 1 in]
            n152 = Bundle(cluster=T40 {"Library Path"="", "Wait Notifier"=refnum, "wait for reply"=FALSE} ("Get Library Argument"), "Library Path"=w375, "Wait Notifier"=w374, "wait for reply"=w373) -> (w376:T40)
            n153 = call-poly <vilib>:"Delacor_lib_QMH_Enqueue Message (poly).vi"("Message Data"=w376, "Message"="Get Library", "Message Queue in"=w379) -> ("error out"=w372:errorcluster)  [unwired: 7 in, 1 out]
          }
        }
        n154 = call-dynamic "Delacor_lib_QMH_Error Handler - Event Handling Loop.vi"("error in"=w33, "Message Queue in"=w27) -> ("dup error in"=w32:errorcluster)  [unwired: 8 in, 1 out]
      }
      n155 = while {
        tunnel: w20 -> [w382]
        shift-right: [w381] -> _
        shift-left: T3 {"Status"="", "Current ID"=0, "References"=variant, "Config Data"={"Allowed Paths"=[]}, "MCP id"=0, "Log"=""} ("Data Cluster") -> [w390]
        tunnel: w24 -> [w392]
        tunnel: [w385] -> w26
        tunnel: w19 -> [w386]
        stop <- w389 stop-if-true
        # "Message Handling Loop"
        n156 = call-dynamic "Delacor_lib_QMH_Dequeue Message.vi"("error in"=w392, "Message Queue in"=w382) -> ("error out"=w391:errorcluster, "Message Data"=w387:variant, "Message"=w388:string, "Message Queue out"=w383:refnum<class "Delacor_lib_QMH_Message Queue.lvclass">)  [unwired: 6 in]
        n157 = case "DQMH_MESSAGE_CASES" shown="\"Get Library\"" w388 {
          selector: w388 -> [_ _ _ _ _ _ _ _ _ _ _ _ _ _ _ _ _ _ _ _ _ _ _ _ _ _ _ _ _ _ _ _ _ _ _ _ _ _ _ _ _ w931]
          tunnel: w383 -> [_ _ _ _ _ _ _ _ _ _ _ _ _ _ _ _ _ _ _ _ _ _ _ _ _ _ _ _ _ _ _ _ _ _ _ _ _ _ _ w895 w920 _]
          tunnel: w391 -> [w413 w417 w432 w449 w463 w478 w493 w505 w520 w534 w548 w562 w576 w591 w605 w619 w633 w649 w664 w679 w693 w708 w721 w734 w747 w760 w772 w788 w799 w810 w826 w838 w848 w856 w864 w875 w880 w882 w891 w902 w925 w934]
          tunnel: [w411 w417 w423 w437 w452 w466 w481 w496 w508 w523 w537 w551 w565 w581 w594 w608 w622 w638 w652 w667 w682 w697 w713 w726 w739 w755 w761 w780 w797 w802 w825 w828 w844 w850 w858 w869 w879 w882 w890 w898 w909 w935] -> w384
          tunnel: w390 -> [w402 w416 w421 w438 w453 w477 w492 w504 w519 w533 w547 w561 w575 w590 w604 w618 w632 w648 w663 w678 w692 w707 w720 w733 w746 w753 w764 w787 w798 w809 w820 w837 w842 w855 w863 w866 w878 w881 w888 w897 w912 w932]
          tunnel: [w393 w416 w422 w442 w456 w469 w484 w498 w512 w525 w540 w554 w567 w580 w597 w610 w625 w639 w656 w671 w685 w700 w711 w724 w737 w751 w764 w779 w793 w801 w821 w837 w843 w849 w857 w865 w878 w881 w888 w897 w912 w932] -> w381
          tunnel: [_ _ _ _ _ _ _ _ _ _ _ _ _ _ _ _ _ _ _ _ _ _ _ _ _ _ _ _ _ _ _ _ _ _ _ _ _ _ _ _ w919 _] -> w389
          tunnel: w387 -> [_ _ w430 w448 w462 w476 w491 w503 w518 w532 w546 w560 w574 w589 w603 w617 w631 w646 w662 w677 w691 w706 w718 w731 w744 _ w771 w785 w796 w807 w824 w835 w846 w853 w861 w873 _ _ _ w896 w918 _]
          tunnel: w386 -> [w403 _ _ _ _ _ _ _ _ _ _ _ _ _ _ _ _ _ _ _ _ _ _ _ _ _ _ _ _ _ _ _ _ _ _ _ _ _ _ w894 w913 _]
          frame "Initialize" {
            w397 = "Initial Message" ("Initial Message")
            # "Initialize - Any operation that needs to be done before the module can receive messages. Synchronize Caller Events.vi will inform Start Module.vi that the module has launched and is ready to receive messages. Module Did Init.vi will broadcast that the module initialized."
            n158 = call "Synchronize Caller Events.vi"("error in"=w413, "Singleton Module Admin in"=w403) -> ("error out"=w412:errorcluster, "Singleton Module Admin out"=w398:refnum<class "Delacor_lib_QMH_Module Admin.lvclass">)  [unwired: 8 in]
            n159 = property on="Property Node" class="Module Admin"(reference=w398) -> ("Accessors:External Launch"=w407:bool)  [unwired: 1 in, 2 out]
            n160 = Select(t=T42."Hidden" ("State"), s=w407, f=T42."Standard" ("State")) -> (s? t:f=w404:T42)
            n161 = call "Module Name--constant.vi"() -> ("Module Name"=w410:string)  [unwired: 11 in]
            n162 = property on="Property Node" class="VI"("Front Panel.Title"=w410) -> (reference out=w409:refnum<vi>, error out=w415:errorcluster)  [unwired: 2 in]
            n163 = invoke on="Invoke Node" class="VI" method="FP.Open"(reference=w409, error in=w415, "State"=w404) -> (reference out=w408:refnum<vi>, error out=w414:errorcluster)  [unwired: 2 in, 3 out]
            n164 = Bundle By Name(cluster=w402, "Status"=w397) -> (w401:T3)
            n165 = invoke on="Invoke Node" class="VI" method="FP.Center"(reference=w408, error in=w414) -> ()  [unwired: 1 in, 3 out]
            n166 = property on="Pane" class="Pane"("Origin"=T41 {"Horizontal"=0, "Vertical"=0}) -> ()  [unwired: 2 in, 2 out]
            n167 = call "Init MCP.vi"("error in (no error)"=w412, "Data Cluster in"=w401) -> ("error out"=w394:errorcluster, "Data Cluster out"=w393:T3)  [unwired: 8 in]
            n168 = call "Read Config Data.vi"("error in"=w394) -> ("error out"=w395:errorcluster)  [unwired: 10 in]
            n169 = call "Module Name--constant.vi"() -> ("Module Name"=w399:string)  [unwired: 11 in]
            n170 = call "Module Did Init.vi"("error in"=w395, "Initialized?"=TRUE, "Origin"=w399) -> ("error out"=w411:errorcluster)  [unwired: 8 in]
            "Status" <- w397
          }
          frame "---Module Specific---" {
            # "Separator -- The following cases handle messages specific to this Module."
          }
          frame "New VI" {
            # "Creates a new VI in the LabVIEW IDE. The VI Reference is stored and returned. This Reference can later be used to e.g. add modifications to the VI."
            n171 = Variant To Data(error in=w432, type=T7 {"Open Frontpanel"=TRUE, "Wait Notifier"=refnum, "wait for reply"=FALSE} ("New VI Argument"), Variant=w430) -> (data=w428:T7, error out=w431:errorcluster)
            n172 = Unbundle By Name(w428) -> ("Open Frontpanel"=w419:bool, "Wait Notifier"=w427:refnum<notifier>, "wait for reply"=w426:bool)
            n173 = call "Create New VI.vi"("Open Frontpanel"=w419, "Data Cluster in"=w421) -> ("message"=w420:string, "ID"=w418:i32, "Data Cluster out"=w422:T3)  [unwired: 7 in]
            n174 = Bundle By Name(cluster=T43 {"VI Reference"=0, "Result"="", "error"={"status"=FALSE, "code"=0, "source"=""}} ("New VI (Reply Payload)"), "Result"=w420, "VI Reference"=w418) -> (w425:T43)
            n175 = Merge Errors(w431) -> (w423:errorcluster)
            n176 = case "DQMH_FIRE_NOTIFIER" shown="True" w426 {
              tunnel: w427 -> [_ w434]
              tunnel: w425 -> [_ w433]
              frame False {
              }
              frame True {
                n177 = Send Notification(notification=w433, notifier=w434) -> ()  [unwired: 1 in, 2 out]
              }
            }
          }
          frame "Add Object" {
            # "Adds an object to the block diagram or frontpanel of the referenced vi. Get a VI reference from \"New VI\".\nAllowed object names are:\n.NET Container\n.NET Refnum\n2D Picture\n3D Picture\nAbsolute Value\nAccept TLS\nAccess Rights\nActiveX Container\nAdd\nAdd (with error terminals)\nAdd Array Elements\nAdd Entropy\nAdd Private Key To TLS Configuration\nAdd Trusted Certificate To TLS Configuration\nAgitator\nAllSpoll\nAlways Copy\nAnd\nAnd Array Elements\nAppend True/False String\nApplication Refnum\nArray (block diagram constant)\nArray (classic)\nArray (modern)\nArray Interface Control\nArray Max & Min\nArray of Strings to Path\nArray Size\nArray Subset\nArray To Cluster\nArray To Spreadsheet String\nArrayMemInfo\nAssert Structural Type Match\nAssert Structural Type Mismatch\nAtmospheric Tank (classic)\nAtmospheric Tank (modern)\nAutomation Close\nAutomation Open\nAutomation Refnum\nAvogadro Constant (1/mol)\nBase 10 Logarithm Of e\nBin #1\nBin #2\nBitpack to Array\nBluetooth Close Connection\nBluetooth Create Listener\nBluetooth Discover\nBluetooth Network Connection Refnum\nBluetooth Open Connection\nBluetooth Read\nBluetooth Wait On Listener\nBluetooth Write\nBoolean Array To Number\nBoolean To (0,1)\nBuild Array\nBuild Cluster Array\nBuild Map\nBuild Matrix\nBuild Path\nBuild Set\nBuild Waveform\nBundle\nBundle By Name\nByte Array To String\nByte Array To UTF-8 String\nByte Stream File Refnum\nCall By Reference\nCall Chain\nCall Library Function Node\nCall MATLAB Function\nCall Parent Class Method\nCAN Channel (block diagram constant)\nCAN Channel (classic)\nCAN Channel (modern)\nCAN Channel (system)\nCAN Interface (block diagram constant)\nCAN Interface (classic)\nCAN Interface (modern)\nCAN Interface (system)\nCAN Task (block diagram constant)\nCAN Task (classic)\nCAN Task (modern)\nCAN Task (system)\nCancel Button (modern)\nCancel Button (system)\nCancel Notification\nCarriage Return Constant\nCase Structure\nCast Unit Bases\nCheck Valve\nCheckbox (classic)\nCheckBox (modern)\nCheckbox (system)\nClass Specifier Constant\nClassic Color Box\nClassic Color Ramp\nClassic Horizontal Slide Switch\nClassic Vertical Slide\nClear Fixed-Point Overflow Status\nClose File\nClose File (deprecated)\nClose MATLAB Session\nClose Python Session\nClose Reference\nClose TLS Configuration\nClose Variable Connection\nClosure Structure\nCluster (classic)\nCluster (modern)\nCluster Constant\nCluster To Array\nCode Interface Node\nCoerce To Type\nCollection Size\nColor Box Constant\nColor Box Thin Border\nColored Rectangle (broken?)\nCombo Box (classic)\nCombo Box (modern)\nCombo Box (system)\nCombo Box Constant\nComplex Conjugate\nComplex To Polar\nComplex To Re/Im\nCompound Arithmetic\nCompressor\nConcatenate Strings\nConditional Disable Structure\nConstructor Node\nControl & Simulation Loop\nControl Help Window\nControl Online Help\nControl Refnum\nConvert Unit\nConveyer\nCopy\nCopy (deprecated)\nCosecant\nCosine\nCotangent\nCPU Information\nCreate Folder\nCreate Network Stream Endpoint\nCreate Network Stream Reader Endpoint\nCreate Network Stream Writer Endpoint\nCreate Stream\nCreate Unique Network Stream Endpoint\nCreate Unique Network Stream Reader Endpoint\nCreate Unique Network Stream Writer Endpoint\nCreate User Event\nCurrent Processor ID\nCurrent VI's Menubar\nCurrent VI's Path\nDAQmx Analog Trigger Source (block diagram constant)\nDAQmx Analog Trigger Source (classic)\nDAQmx Analog Trigger Source (modern)\nDAQmx Analog Trigger Source (system)\nDAQmx Device Name (block diagram constant)\nDAQmx Device Name (classic)\nDAQmx Device Name (modern)\nDAQmx Device Name (system)\nDAQmx Global Channel (block diagram constant)\nDAQmx Global Channel (classic)\nDAQmx Global Channel (modern)\nDAQmx Global Channel (system)\nDAQmx Physical Channel (block diagram constant)\nDAQmx Physical Channel (classic)\nDAQmx Physical Channel (modern)\nDAQmx Physical Channel (system)\nDAQmx Scale Name (block diagram constant)\nDAQmx Scale Name (classic)\nDAQmx Scale Name (modern)\nDAQmx Scale Name (system)\nDAQmx Switch (block diagram constant)\nDAQmx Switch (classic)\nDAQmx Switch (modern)\nDAQmx Switch (system)\nDAQmx Task Name (block diagram constant)\nDAQmx Task Name (classic)\nDAQmx Task Name (modern)\nDAQmx Task Name (system)\nDAQmx Terminal (block diagram constant)\nDAQmx Terminal (classic)\nDAQmx Terminal (modern)\nDAQmx Terminal (system)\nData Cache Size\nData Log File Refnum\nData Value Reference\nData Value Reference Constant\nDataSocket Close\nDataSocket Open\nDataSocket Read\nDataSocket Refnum\nDataSocket Write\nDate/Time To Seconds\nDecimal Digit?\nDecimal String To Number\nDecimate 1D Array\nDecomposeLockDataValRef\nDecomposeVariant\nDecrement\nDefault Directory\nDelete\nDelete (deprecated)\nDelete Data Value Reference\nDelete From Array\nDelete Menu Items\nDelete Variant Attribute\nDelete Waveform Attribute\nDeny Access\nDequeue Element\nDestroy Stream Endpoint\nDestroy User Event\nDevClear\nDevClearList\nDevice Control/Status\nDevice Refnum\nDiagram Disable Structure\nDial (classic)\nDial (modern)\nDigital Data (classic)\nDigital Data (modern)\nDigital Waveform Graph (classic)\nDigital Waveform Graph (modern)\nDirect Variable Read\nDirect Variable Write\nDivide\nDivide (with error terminals)\nDlg Horiz Scrollbar\nDlg Mac Group Box\nDlg Numeric #1\nDlg Numeric #2\nDlg String\nDlg Vert Scrollbar\nDown Arrow\nDown Bow Valve (flat)\nDown Bow Valve (outline)\nDown Bow Valve (shaded)\nDown Rect Valve (flat)\nDown Rect Valve (outline)\nDown Rect Valve (shaded)\nDown Tee (flat)\nDown Tee (shaded)\nDynamic FPGA Interface Cast\nEased Corner Rectangle\nElement of Set?\nElementary Charge (C)\nEmpty Array?\nEmpty Collection?\nEmpty Path Constant\nEmpty String Constant\nEmpty String/Path?\nEnable Menu Tracking\nEnableLocal\nEnableRemote\nEnd of Line Constant\nEnqueue Element\nEnqueue Element At Opposite End\nEnum (classic)\nEnum (modern)\nEnum (system)\nEnum Constant\nEOF\nEqual To 0?\nEqual?\nError Ring Constant\nEvent Callback Refnum\nEvent Data Node\nEvent Structure\nExchanger\nExclusive Or\nExponential\nExponential (Arg) -1\nExpression Node\nFalse Constant\nFeedback Node\nFieldPoint IO Point (block diagram constant)\nFieldPoint IO Point (classic)\nFieldPoint IO Point (modern)\nFIFO Refnum\nFile Dialog\nFile Dialog (deprecated)\nFile Path Control (classic)\nFile Path Control (modern)\nFile Path Control (system)\nFile Path Indicator (classic)\nFile Path Indicator (modern)\nFile/Directory Info\nFile/Directory Info (deprecated)\nFindLstn\nFindRQS\nFirst Call?\nFixed-Point Overflow?\nFixed-Point to Integer Cast\nFlat Box\nFlat Circle\nFlat Down Triangle\nFlat Frame\nFlat Left Triangle\nFlat Right Triangle\nFlat Round Button\nFlat Rounded Box\nFlat Sequence Structure\nFlat Square Button\nFlat Up Triangle\nFlatten To JSON\nFlatten To String\nFlatten To XML\nFlattened String To Variant\nFloating Point Equal?\nFlush Event Queue\nFlush File\nFlush File (deprecated)\nFlush Queue\nFlush Stream\nFor Loop\nFork\nFormat Date/Time String\nFormat Into File\nFormat Into String\nFormat Value\nFormula Node\nFPGA Refnum to Session\nFract/Exp String To Number\nFramed Color Box (classic)\nFramed Color Box (modern)\nFree Label\nFurnace\nGauge (classic)\nGauge (modern)\nGauge for Simon\nGenerate Front Panel Activity\nGenerate Occurrence\nGenerate User Event\nGenerate User-Defined Trace Event\nGet Control Values by Index\nGet Datalog Position\nGet Date/Time In Seconds\nGet Date/Time String\nGet Drag Drop Data\nGet File Position\nGet File Size\nGet Fixed-Point Components\nGet Help Window Status\nGet Matrix Diagonal\nGet Matrix Elements\nGet Menu Item Info\nGet Menu Selection\nGet Menu Short Cut Info\nGet Notifier Status\nGet Number of Records\nGet Permissions\nGet Queue Status\nGet Submatrix\nGet Type and Creator\nGet Variant Attribute\nGet Volume Info\nGet Waveform Attribute\nGet Waveform Components\nGlobal Variable\nGPIB Clear\nGPIB Initialization\nGPIB Misc\nGPIB Read\nGPIB Serial Poll\nGPIB Status\nGPIB Trigger\nGPIB Wait\nGPIB Write\nGravitational Constant (N m2/kg2)\nGreater Or Equal To 0?\nGreater Or Equal?\nGreater Than 0?\nGreater?\nHandle Peek\nHandle Poke\nHex Digit?\nHexadecimal String To Number\nHopper #1\nHopper #2\nHoriz Line\nHoriz Pipe (flat)\nHoriz Pipe (shaded)\nHorizontal Button Box\nHorizontal Fill Slide (classic)\nHorizontal Fill Slide (modern)\nHorizontal Gradient Oval\nHorizontal Gradient Rectangle\nHorizontal Gradient Rounded Rectangle\nHorizontal Graduated Bar\nHorizontal Pointer Slide (classic)\nHorizontal Pointer Slide (modern)\nHorizontal Pointer Slide (system)\nHorizontal Progress Bar (modern)\nHorizontal Progress Bar (system)\nHorizontal Scrollbar\nHorizontal Slide (classic)\nHorizontal Slide (system)\nHorizontal Smooth Box\nHorizontal Splitter Bar\nHorizontal Splitter Bar (Classic)\nHorizontal Splitter Bar (NXG Style)\nHorizontal Splitter Bar (System)\nHorizontal Switch\nHorizontal Tank\nHorizontal Toggle Switch (classic)\nHorizontal Toggle Switch (modern)\nHyperbolic Cosecant\nHyperbolic Cosine\nHyperbolic Cotangent\nHyperbolic Secant\nHyperbolic Sine\nHyperbolic Tangent\nIMAQ Session\nImplies\nIn Place Element Structure\nIn Range and Coerce\nInclude Fixed-Point Overflow Status\nIncrement\nIndex & Bundle Cluster Array\nIndex Array\nIndex String Array\nInitialize Array\nInline C Node\nInsert Into Array\nInsert Into Map\nInsert Into Set\nInsert Menu Items\nInteger to Fixed-Point Cast\nIntensity Chart (classic)\nIntensity Chart (modern)\nIntensity Graph (classic)\nIntensity Graph (modern)\nInterleave 1D Arrays\nInterpolate 1D Array\nInverse Cosecant\nInverse Cosine\nInverse Cotangent\nInverse Hyperbolic Cosecant\nInverse Hyperbolic Cosine\nInverse Hyperbolic Cotangent\nInverse Hyperbolic Secant\nInverse Hyperbolic Sine\nInverse Hyperbolic Tangent\nInverse Secant\nInverse Sine\nInverse Tangent\nInverse Tangent (2 Input)\nInvoke Node\nIP To String\nIrDA Close Connection\nIrDA Create Listener\nIrDA Discover\nIrDA Network Connection Refnum\nIrDA Open Connection\nIrDA Read\nIrDA Wait On Listener\nIrDA Write\nIsDebuggingActive\nIVI Delete Session\nIVI Logical Name (block diagram constant)\nIVI Logical Name (classic)\nIVI Logical Name (modern)\nIVI New Session\nJoin\nJoin Numbers\nJunction\nKnob (classic)\nKnob (modern)\nLabel (modern)\nLabel (system)\nLabeled Oblong Button\nLabeled Rectangular Button\nLabeled Round Button\nLabeled Square Button\nLabVIEW Object\nLeak Variant Value Reference\nLED Button\nLeft Arrow\nLeft Bow Valve (flat)\nLeft Bow Valve (outline)\nLeft Bow Valve (shaded)\nLeft Down Elbow (flat)\nLeft Down Elbow (shaded)\nLeft Pump (flat)\nLeft Pump (shaded)\nLeft Rect Valve (flat)\nLeft Rect Valve (outline)\nLeft Rect Valve (shaded)\nLeft Tee (flat)\nLeft Tee (shaded)\nLeft Up Elbow (flat)\nLeft Up Elbow (shaded)\nLess Or Equal To 0?\nLess Or Equal?\nLess Than 0?\nLess?\nLexical Class\nLine (chiseled, system)\nLine (chiseled, thick)\nLine (chiseled, thin)\nLine (thick)\nLine (thin)\nLine Feed Constant\nLine with Arrow (thick)\nLine with Arrow (thin)\nList Directory\nList Folder\nListbox (classic)\nListbox (modern)\nListbox (system)\nListbox Symbol Ring Constant\nLoad Certificates Into Memory\nLoad Private Key Into Memory\nLocal Variable\nLock Range\nLogarithm Base 10\nLogarithm Base 2\nLogarithm Base X\nLogical Shift\nLook In Map\nLookup Channel Probe\nLossy Enqueue Element\nLowered Box (thick)\nLowered Rounded Box\nMachine Epsilon\nMake TLS Configuration Immutable\nMakeAddr\nMantissa & Exponent\nMap\nMap Constant\nMatch First String\nMatch Pattern\nMatch True/False String\nMathScript Call By Reference\nMathScript Node\nMATLAB script\nMATLAB Session Refnum\nMatrix Size\nMax & Min\nMenu Refnum\nMenu Ring (classic)\nMenu Ring (modern)\nMenu-Popup Ring\nMerge Errors\nMerge Signals\nMeter (classic)\nMeter (modern)\nMixed Checkbox (system)\nMixed Signal Graph\nMolar Gas Constant (J/(mol K))\nMotion Resource (block diagram constant)\nMotion Resource (classic)\nMotion Resource (modern)\nMotor (flat)\nMotor (shaded)\nMove\nMove (deprecated)\nMulti-Segment Pipe\nMulticolumn Listbox (classic)\nMulticolumn Listbox (modern)\nMulticolumn Listbox (system)\nMultiply\nMultiply (with error terminals)\nMultiply Array Elements\nMultirate Structure\nNatural Logarithm\nNatural Logarithm (Arg +1)\nNatural Logarithm Base\nNatural Logarithm Of 10\nNatural Logarithm Of 2\nNatural Logarithm Of Pi\nNegate\nNegative Infinity\nNew Data Value Reference\nNew Directory\nNew File\nNew TLS Configuration\nNew VI\nNew VI Object\nNot\nNot A Number/Path/Refnum?\nNot A Path Constant\nNot a Refnum Constant\nNot a Shared Variable\nNot And\nNot Equal To 0?\nNot Equal?\nNot Exclusive Or\nNot Or\nNotifier Refnum\nNumber of Cache Levels\nNumber To Boolean Array\nNumber To Decimal String\nNumber To Engineering String\nNumber To Exponential String\nNumber To Fractional String\nNumber To Hexadecimal String\nNumber To Octal String\nNumeric Constant\nNumeric Control (classic)\nNumeric Control (modern)\nNumeric Control (system)\nNumeric Indicator (classic)\nNumeric Indicator (modern)\nObtain Notifier\nObtain Queue\nOccurrence Refnum\nOctal Digit?\nOctal String To Number\nOK Button (modern)\nOK Button (system)\nOld VISA Open\nOLE Variant\nOne Button Dialog\nOpen and Verify Variable Connection\nOpen Application Reference\nOpen Device\nOpen Dynamic Bitfile Reference\nOpen File\nOpen MATLAB Session\nOpen Python Session\nOpen Tank (flat classic)\nOpen Tank (shaded classic)\nOpen Variable Connection\nOpen Variable Connection in Background\nOpen VI Object Reference\nOpen VI Reference\nOpen/Create/Replace Datalog\nOpen/Create/Replace File\nOr\nOr Array Elements\nOval with Shadow\nPackage Matrix\nPassControl\nPath Constant\nPath to Array of Strings\nPath To String\nPath Type\nPi\nPi Divided By 2\nPi Multiplied By 2\nPick Line\nPict Ring (classic)\nPict Ring (modern)\nPict Ring (system)\nPixMap\nPixMap (warning: dangerous)\nPlanck's Constant (J/Hz)\nPlatform Flat Square Button\nPlug-In Control\nPolar To Complex\nPolar To Re/Im\nPositive Infinity\nPower Of 10\nPower Of 2\nPower Of X\nPPoll\nPPollConfig\nPPollUnconfig\nPreallocated Read from Binary File\nPreserve Run-Time Class\nPressure Tank (flat)\nPressure Tank (shaded)\nPreview Queue Element\nPrintable?\nProperty Node\nPulldown Menu Ring\nPush Button\nPython Node\nPython Session Refnum\nQueue Refnum\nQuit LabVIEW\nQuotient & Remainder\nRace Structure\nRadio Button (system)\nRadio Buttons (classic)\nRadio Buttons (modern)\nRadio Buttons (system)\nRaised Box (classic)\nRaised Box (modern)\nRaised Circle\nRaised Down Triangle\nRaised Frame\nRaised Left Triangle\nRaised Right Triangle\nRaised Rounded Box\nRaised Up Triangle\nRandom Number (0-1)\nRcvRespMsg\nRe-accept TLS\nRe/Im To Complex\nRe/Im To Polar\nRead Datalog\nRead Device\nRead File\nRead from Binary File\nRead from Text File\nRead Map Max & Min Keys\nRead Multiple Elements from Stream\nRead Set Max & Min\nRead Single Element from Stream\nRead Variable\nRead Variable with Timeout\nReadStatus\nReceive\nReceiveSetup\nRecessed Box\nRecessed Circle\nRecessed Down Triangle\nRecessed Frame (modern)\nRecessed Frame (system)\nRecessed Left Triangle\nRecessed Menu Ring\nRecessed Right Triangle\nRecessed Rounded Box\nRecessed Up Triangle\nReciprocal\nReciprocal Of e\nReciprocal Of Pi\nRecomposeUnlockDataValRef (warning: dangerous)\nRecomposeVariant (warning: dangerous)\nRectangular Stop Button\nRefnum to Path\nRefnum to Session\nRegion\nRegister Event Callback\nRegister For Events\nRegister Session\nRelease Notifier\nRelease Queue\nRemove Fixed-Point Overflow Status\nRemove From Map\nRemove From Set\nReplace Array Subset\nReplace Substring\nRequest Deallocation\nResetSys\nReshape Array\nResize Matrix\nResource Index\nReverse 1D Array\nReverse String\nRight Arrow\nRight Bow Valve (flat)\nRight Bow Valve (outline)\nRight Bow Valve (shaded)\nRight Down Elbow (flat)\nRight Down Elbow (shaded)\nRight Pump (flat)\nRight Pump (shaded)\nRight Rect Valve (flat)\nRight Rect Valve (outline)\nRight Rect Valve (shaded)\nRight Tee (flat)\nRight Tee (shaded)\nRight Up Elbow (flat)\nRight Up Elbow (shaded)\nRocker\nRotary Feeder\nRotate\nRotate 1D Array\nRotate Left With Carry\nRotate Right With Carry\nRotate String\nRound Button\nRound LED (classic)\nRound LED (modern)\nRound Light\nRound Push Button\nRound Push Button (profile)\nRound Radio Button\nRound Stop Button\nRound To Nearest\nRound Toward +Infinity\nRound Toward -Infinity\nRounded Rectangle with Shadow\nRT FIFO Create\nRT FIFO Delete\nRT FIFO Read\nRT FIFO Write\nRydberg Constant (1/m)\nScale By Power Of 2\nScan From File\nScan From String\nScan String For Tokens\nScan Value\nScanned Variable Read\nScanned Variable Write\nSearch 1D Array\nSearch and Replace String\nSearch Variable Container\nSearch/Split String\nSecant\nSeconds To Date/Time\nSeek\nSelect\nSend\nSend Notification\nSendCmds\nSendDataBytes\nSendIFC\nSendList\nSendLLO\nSendSetup\nSession to Refnum\nSet\nSet Constant\nSet Control Values by Index\nSet Datalog Position\nSet File Position\nSet File Size\nSet Matrix Diagonal\nSet Matrix Elements\nSet Menu Item Info\nSet Number of Records\nSet Occurrence\nSet Permissions\nSet Submatrix\nSet Type and Creator\nSet Variant Attribute\nSet Waveform Attribute\nSetRWLS\nSetTimeOut\nShared Variable\nShared Variable Constant\nShared Variable Control (classic)\nShared Variable Control (modern)\nShared Variable to String\nSign\nSimple Horizontal Slide\nSimple Numeric\nSimple String\nSimple Vertical Slide\nSinc\nSine\nSine & Cosine\nSize Handle\nSlide Switch\nSmoothed Oval\nSmoothed Rounded Rectangle\nSort 1D Array\nSort Array of String\nSpeed Of Light In Vacuum (m/sec)\nSpin Control (system)\nSplit 1D Array\nSplit Button\nSplit Number\nSplit Signals\nSpreadsheet String To Array\nSquare\nSquare Button\nSquare LED (classic)\nSquare LED (modern)\nSquare Light\nSquare Push Button\nSquare Push Button (profile)\nSquare Radio Button\nSquare Root\nStacked Sequence Structure\nStart TLS\nState\nState Diagram\nStatic VI Reference\nStop\nStop Button\nString Constant\nString Control (classic)\nString Control (modern)\nString Control (system)\nString Indicator (classic)\nString Indicator (modern)\nString Length\nString Subset\nString To Byte Array\nString To IP\nString To Path\nString to Shared Variable\nStrip Path\nSubPanel\nSubPanel (Classic)\nSubPanel (NXG Style)\nSubPanel (System)\nSubtract\nSubtract (with error terminals)\nSwap Bytes\nSwap Values\nSwap Vector Element\nSwap Words\nTab Constant\nTab Control (classic)\nTab Control (modern)\nTab Control (NXG Style)\nTab Control (system)\nTable (classic)\nTable (modern)\nTable (system)\nTag Attribute Ring\nTangent\nTank (classic)\nTank (modern)\nTarget Structure\nTCP Close Connection\nTCP Create Listener\nTCP Flattened Read\nTCP Flattened Write\nTCP Flex Read\nTCP Flex Write\nTCP Network Connection Refnum\nTCP Open Connection\nTCP Read\nTCP Wait On Listener\nTCP Write\nTDMS Advanced Asynchronous Read (Data Ref)\nTDMS Advanced Asynchronous Write (Data Ref)\nTDMS Close\nTDMS Configure Asynchronous Reads (Data Ref)\nTDMS Configure Asynchronous Writes (Data Ref)\nTDMS Defragment\nTDMS Delete Data\nTDMS File\nTDMS Flush\nTDMS Get Asynchronous Read Status (Data Ref)\nTDMS Get Asynchronous Write Status (Data Ref)\nTDMS Get Properties\nTDMS In Memory Close\nTDMS In Memory Open\nTDMS In Memory Read Bytes\nTDMS List Contents\nTDMS Open\nTDMS Read\nTDMS Refnum To File ID\nTDMS Set Properties\nTDMS Write\nTDMS Write IP\nTemporary Directory\nTestSRQ\nTestSys\nText & Pict Ring (classic)\nText & Pict Ring (modern)\nText Button\nText Ring (block diagram constant)\nText Ring (classic)\nText Ring (modern)\nText Ring (system)\nText to UTF-8\nThermometer (classic)\nThermometer (modern)\nThreshold 1D Array\nTick Count (ms)\nTime Stamp (block diagram constant)\nTime Stamp Control (classic)\nTime Stamp Control (modern)\nTime Stamp Control (system)\nTime Stamp Indicator (classic)\nTime Stamp Indicator (modern)\nTimed Loop\nTimed Sequence\nTLS configuration\nTLS Connection?\nTo Byte Integer\nTo Double Precision Complex\nTo Double Precision Float\nTo Extended Precision Complex\nTo Extended Precision Float\nTo Fixed-Point\nTo Long Integer\nTo Lower Case\nTo More Generic Class\nTo More Specific Class\nTo OLE Variant\nTo Probe String\nTo Quad Integer\nTo Single Precision Complex\nTo Single Precision Float\nTo Time Stamp\nTo Unsigned Byte Integer\nTo Unsigned Long Integer\nTo Unsigned Quad Integer\nTo Unsigned Word Integer\nTo Upper Case\nTo Variant\nTo Word Integer\nTraditional DAQ Channel (block diagram constant)\nTraditional DAQ Channel (classic)\nTraditional DAQ Channel (modern)\nTranspose 1D Array\nTranspose 2D Array\nTranspose Matrix\nTree (classic)\nTree (modern)\nTree (system)\nTrigger\nTriggerList\nTwo Button Dialog\nType and Creator\nType Cast\nType Error\nType Must Be Array\nType Must Be Cluster\nType Of\nType Specialization Structure\nUDP Close\nUDP Multicast Open\nUDP Network Connection Refnum\nUDP Open\nUDP Read\nUDP Write\nUnbitpack from Array\nUnbundle\nUnbundle By Name\nUnflatten From JSON\nUnflatten From String\nUnflatten From XML\nUnleak Variant Value Reference\nUnpackage Matrix\nUnregister For Events\nUnregister Session\nUp Arrow\nUp Bow Valve (flat)\nUp Bow Valve (outline)\nUp Bow Valve (shaded)\nUp Rect Valve (flat)\nUp Rect Valve (outline)\nUp Rect Valve (shaded)\nUp Tee (flat)\nUp Tee (shaded)\nUser Defined Refnum\nUser Defined Refnum Tag (block diagram constant)\nUser Defined Refnum Tag (classic)\nUser Defined Refnum Tag (modern)\nUser Defined Refnum Tag Flatten (classic)\nUser Defined Refnum Tag Flatten (modern)\nUser Defined Tag (block diagram constant)\nUser Defined Tag (classic)\nUser Defined Tag (modern)\nUser Item\nUTF-8 String To Byte Array\nUTF-8 to Text\nVariable Class Specifier Constant\nVariable Name Constant\nVariant\nVariant To Data\nVariant To Flattened String\nVert Line\nVert Pipe (flat)\nVert Pipe (shaded)\nVert Rocker\nVertical Fill Slide (classic)\nVertical Fill Slide (modern)\nVertical Gradient Oval\nVertical Gradient Rectangle\nVertical Gradient Rounded Rectangle\nVertical Graduated Bar\nVertical Pointer Slide (classic)\nVertical Pointer Slide (modern)\nVertical Pointer Slide (system)\nVertical Progress Bar (modern)\nVertical Progress Bar (system)\nVertical Scrollbar\nVertical Slide (system)\nVertical Slide Switch (classic)\nVertical Slide Switch (modern)\nVertical Smooth Box\nVertical Splitter Bar\nVertical Splitter Bar (Classic)\nVertical Splitter Bar (NXG Style)\nVertical Splitter Bar (System)\nVertical Switch\nVertical Toggle Switch (classic)\nVertical Toggle Switch (modern)\nVI Library\nVI Refnum\nVI Server Reference\nVISA Assert Interrupt Signal\nVISA Assert Trigger\nVISA Assert Utility Signal\nVISA Clear\nVISA Close\nVISA Disable Event\nVISA Discard Events\nVISA Enable Event\nVISA Find Resource\nVISA Flush I/O Buffer\nVISA GPIB Command\nVISA GPIB Control ATN\nVISA GPIB Control REN\nVISA GPIB Pass Control\nVISA GPIB Send IFC\nVISA In 16\nVISA In 32\nVISA In 64\nVISA In 8\nVISA Lock\nVISA Map Address\nVISA Map Trigger\nVISA Memory Allocation\nVISA Memory Allocation Ex\nVISA Memory Free\nVISA Move\nVISA Move In 16\nVISA Move In 32\nVISA Move In 64\nVISA Move In 8\nVISA Move Out 16\nVISA Move Out 32\nVISA Move Out 64\nVISA Move Out 8\nVISA Open\nVISA Out 16\nVISA Out 32\nVISA Out 64\nVISA Out 8\nVISA Peek 16\nVISA Peek 32\nVISA Peek 64\nVISA Peek 8\nVISA Poke 16\nVISA Poke 32\nVISA Poke 64\nVISA Poke 8\nVISA Read\nVISA Read STB\nVISA Read To File\nVISA Refnum to Session\nVISA Resource Name\nVISA resource name (classic)\nVISA resource name (modern)\nVISA Set I/O Buffer Size\nVISA Status Description\nVISA Unlock\nVISA Unmap Address\nVISA Unmap Trigger\nVISA USB Control In\nVISA USB Control Out\nVISA VXI Cmd or Query\nVISA Wait on Event\nVISA Write\nVISA Write From File\nVolume Info\nWait (ms)\nWait For Activity\nWait For Front Panel Activity\nWait for GPIB RQS\nWait on Notification\nWait on Notification from Multiple\nWait on Notification from Multiple with Notifier History\nWait on Notification with Notifier History\nWait on Occurrence\nWait Until Next ms Multiple\nWaitSRQ\nWaveform Chart\nWaveform Chart (classic)\nWaveform Chart (modern)\nWaveform Graph (classic)\nWaveform Graph (modern)\nWhile Loop #1\nWhile Loop #2\nWhite Space?\nWrite Datalog\nWrite Device\nWrite File\nWrite Multiple Elements to Stream\nWrite Single Element to Stream\nWrite to Binary File\nWrite to Text File\nWrite Variable\nWrite Variable with Timeout\nXY Graph (classic)\nXY Graph (modern)\nY-th Root of X"
            n178 = Variant To Data(error in=w449, type=T8 {"VI Reference"=0, "Object Name"="", "Wait Notifier"=refnum, "wait for reply"=FALSE, "position_x"=0, "position_y"=0} ("Add Object Argument"), Variant=w448) -> (data=w435:T8, error out=w437:errorcluster)
            n179 = Unbundle By Name(w435) -> ("Wait Notifier"=w446:refnum<notifier>, "wait for reply"=w445:bool)
            n180 = control-ref of="Ring 2"() -> (w439:refnum<vi>)
            n181 = call "add vi object.vi"("Ring in"=w439, "error in (no error)"=w437, "Add Object Argument"=w435, "Data Cluster in"=w438) -> ("error out"=w441:errorcluster, "Result"=w440:string, "object_id"=w436:i32, "Data Cluster out"=w442:T3)  [unwired: 4 in]
            n182 = Bundle By Name(cluster=T44 {"error"={"status"=FALSE, "code"=0, "source"=""}, "Object ID"=0, "Result"=""} ("Add Object (Reply Payload)"), "error"=w441, "Result"=w440, "Object ID"=w436) -> (w444:T44)
            n183 = case "DQMH_FIRE_NOTIFIER" shown="True" w445 {
              tunnel: w446 -> [_ w451]
              tunnel: w444 -> [_ w450]
              frame False {
              }
              frame True {
                n184 = Send Notification(notification=w450, notifier=w451) -> ()  [unwired: 1 in, 2 out]
              }
            }
          }
          frame "Connect Objects" {
            # "Connects two terminals of two objects with a wire on the block diagram of a labview vi. To get a new VI use \"new vi\" to add objects to a vi use \"add object\"."
            n185 = Variant To Data(error in=w463, type=T9 {"vi reference"=0, "from object reference"=0, "to object reference"=0, "from object terminal index"=0, "to object terminal index"=0, "Wait Notifier"=refnum, "wait for reply"=FALSE} ("Connect Objects Argument"), Variant=w462) -> (data=w454:T9, error out=w452:errorcluster)
            n186 = Unbundle By Name(w454) -> ("Wait Notifier"=w460:refnum<notifier>, "wait for reply"=w459:bool)
            n187 = call "Wire Two Objects.vi"("error in (no error)"=w452, "input cluster"=w454, "Data Cluster in"=w453) -> ("error out"=w455:errorcluster, "Data Cluster out"=w456:T3)  [unwired: 7 in]
            n188 = Bundle By Name(cluster=T45 {"result"="", "error"={"status"=FALSE, "code"=0, "source"=""}} ("Connect Objects (Reply Payload)"), "error"=w455) -> (w458:T45)
            n189 = case "DQMH_FIRE_NOTIFIER" shown="True" w459 {
              tunnel: w460 -> [_ w465]
              tunnel: w458 -> [_ w464]
              frame False {
              }
              frame True {
                n190 = Send Notification(notification=w464, notifier=w465) -> ()  [unwired: 1 in, 2 out]
              }
            }
          }
          frame "Get Object Terminals" {
            # "Returns the Terminals Names and/or descriptions as a string as well as their Index to be used in other functions like connect objects."
            n191 = Variant To Data(error in=w478, type=T10 {"object id"=0, "Wait Notifier"=refnum, "wait for reply"=FALSE} ("Get Object Terminals Argument"), Variant=w476) -> (data=w470:T10, error out=w466:errorcluster)
            n192 = Unbundle By Name(w470) -> ("Wait Notifier"=w474:refnum<notifier>, "wait for reply"=w473:bool)
            n193 = call "get terminal info.vi"("error in (no error)"=w466, "Get Object Terminals Argument"=w470, "Data Cluster in"=w477) -> ("error out"=w468:errorcluster, "String"=w467:string, "Data Cluster out"=w469:T3)  [unwired: 6 in]
            n194 = Bundle By Name(cluster=T46 {"terminals description"="", "error"={"status"=FALSE, "code"=0, "source"=""}} ("Get Object Terminals (Reply Payload)"), "terminals description"=w467, "error"=w468) -> (w472:T46)
            n195 = case "DQMH_FIRE_NOTIFIER" shown="True" w473 {
              tunnel: w474 -> [_ w480]
              tunnel: w472 -> [_ w479]
              frame False {
              }
              frame True {
                n196 = Send Notification(notification=w479, notifier=w480) -> ()  [unwired: 1 in, 2 out]
              }
            }
          }
          frame "get vi error list" {
            # "Returns the current error list (list you see when clicking the run arrow) in a text format giving information about what on the block diagram needs to be fixed. Use this to see if your actions worked."
            n197 = Variant To Data(error in=w493, type=T11 {"vi id"=0, "Wait Notifier"=refnum, "wait for reply"=FALSE} ("get vi error list Argument"), Variant=w491) -> (data=w485:T11, error out=w481:errorcluster)
            n198 = Unbundle By Name(w485) -> ("Wait Notifier"=w489:refnum<notifier>, "wait for reply"=w488:bool)  [unwired: 1 out]
            n199 = call "generate vi error list.vi"("error in (no error)"=w481, "get vi error list Argument"=w485, "Data Cluster in"=w492) -> ("error out"=w482:errorcluster, "Error Description"=w483:string, "Data Cluster out"=w484:T3)  [unwired: 6 in]
            n200 = Bundle By Name(cluster=T47 {"error list"="", "error"={"status"=FALSE, "code"=0, "source"=""}} ("get vi error list (Reply Payload)"), "error list"=w483, "error"=w482) -> (w487:T47)
            n201 = case "DQMH_FIRE_NOTIFIER" shown="True" w488 {
              tunnel: w489 -> [_ w495]
              tunnel: w487 -> [_ w494]
              frame False {
              }
              frame True {
                n202 = Send Notification(notification=w494, notifier=w495) -> ()  [unwired: 1 in, 2 out]
              }
            }
          }
          frame "Cleanup VI" {
            # "Cleans up the block diagram of a vi referenced by reference number."
            n203 = Variant To Data(error in=w505, type=T12 {"vi reference"=0, "Wait Notifier"=refnum, "wait for reply"=FALSE} ("Cleanup VI Argument"), Variant=w503) -> (data=w497:T12, error out=w496:errorcluster)
            n204 = Unbundle By Name(w497) -> ("Wait Notifier"=w501:refnum<notifier>, "wait for reply"=w500:bool)
            n205 = call "clean up vis blockdiagram.vi"("error in (no error)"=w496, "Cleanup VI Argument"=w497, "Data Cluster in"=w504) -> ("Cleanup VI (Reply Payload)"=w499:T64, "Data Cluster out"=w498:T3)  [unwired: 6 in, 1 out]
            n206 = case "DQMH_FIRE_NOTIFIER" shown="True" w500 {
              tunnel: w501 -> [_ w507]
              tunnel: w499 -> [_ w506]
              frame False {
              }
              frame True {
                n207 = Send Notification(notification=w506, notifier=w507) -> ()  [unwired: 1 in, 2 out]
              }
            }
          }
          frame "create_control" {
            # "Creates a control or indicator on the terminal specified by Object ID and Terminal Index, depending on if it's a in- or output of the node. If Constant is set to True, it can only be used on node inputs and will create a constant.\nIt will return the reference to the created control or indicator, that is a reference to the frontpanel element. If constant is True it returns a reference to the block diagram object (constant)."
            n208 = Variant To Data(error in=w520, type=T13 {"Object ID"=0, "Terminal Index"=0, "Constant"=FALSE, "Wait Notifier"=refnum, "wait for reply"=FALSE, "Value"=""} ("create_control Argument"), Variant=w518) -> (data=w511:T13, error out=w508:errorcluster)
            n209 = Unbundle By Name(w511) -> ("Wait Notifier"=w516:refnum<notifier>, "wait for reply"=w515:bool)  [unwired: 3 out]
            n210 = call "Do Create Control.vi"("error in (no error)"=w508, "create_control Argument"=w511, "Data Cluster in"=w519) -> ("error out"=w509:errorcluster, "new reference"=w510:i32, "Data Cluster out"=w512:T3)  [unwired: 6 in]
            n211 = Bundle By Name(cluster=T48 {"Object ID"=0, "error"={"status"=FALSE, "code"=0, "source"=""}} ("create_control (Reply Payload)"), "Object ID"=w510, "error"=w509) -> (w514:T48)
            n212 = case "DQMH_FIRE_NOTIFIER" shown="True" w515 {
              tunnel: w516 -> [_ w522]
              tunnel: w514 -> [_ w521]
              frame False {
              }
              frame True {
                n213 = Send Notification(notification=w521, notifier=w522) -> ()  [unwired: 1 in, 2 out]
              }
            }
          }
          frame "Run VI" {
            # "Runs a VI specified by VI ID and brings the frontpanel to foreground if open_frontpanel is set to True."
            n214 = Variant To Data(error in=w534, type=T14 {"VI ID"=0, "open_frontpanel"=FALSE, "Wait Notifier"=refnum, "wait for reply"=FALSE} ("Run VI Argument"), Variant=w532) -> (data=w526:T14, error out=w523:errorcluster)
            n215 = Unbundle By Name(w526) -> ("Wait Notifier"=w530:refnum<notifier>, "wait for reply"=w529:bool)
            n216 = call "Do Run VI.vi"("error in (no error)"=w523, "Run VI Argument"=w526, "Data Cluster in"=w533) -> ("error out"=w524:errorcluster, "Data Cluster out"=w525:T3)  [unwired: 7 in]
            n217 = Bundle By Name(cluster=T49 {"error"={"status"=FALSE, "code"=0, "source"=""}} ("Run VI (Reply Payload)"), "error"=w524) -> (w528:T49)
            n218 = case "DQMH_FIRE_NOTIFIER" shown="True" w529 {
              tunnel: w530 -> [_ w536]
              tunnel: w528 -> [_ w535]
              frame False {
              }
              frame True {
                n219 = Send Notification(notification=w535, notifier=w536) -> ()  [unwired: 1 in, 2 out]
              }
            }
          }
          frame "add_to_selection" {
            # "Adds an object specified by object_id to the selection list. Use this to copy & paste or enclose a selection. Use clear_selection or remove_from_selection to remove the object from the list. Make sure to check if the selection list looks good."
            n220 = Variant To Data(error in=w548, type=T15 {"object_id"=0, "Wait Notifier"=refnum, "wait for reply"=FALSE, "vi_id"=0} ("add_to_selection Argument"), Variant=w546) -> (data=w539:T15, error out=w537:errorcluster)
            n221 = Unbundle By Name(w539) -> ("Wait Notifier"=w544:refnum<notifier>, "wait for reply"=w543:bool)
            n222 = call "Do Add To Selection.vi"("error in (no error)"=w537, "add_to_selection Argument"=w539, "Data Cluster in"=w547) -> ("error out"=w538:errorcluster, "Data Cluster out"=w540:T3)  [unwired: 7 in]
            n223 = Bundle By Name(cluster=T50 {"Current Selection"=[], "error"={"status"=FALSE, "code"=0, "source"=""}} ("add_to_selection (Reply Payload)"), "error"=w538) -> (w542:T50)
            n224 = case "DQMH_FIRE_NOTIFIER" shown="True" w543 {
              tunnel: w544 -> [_ w550]
              tunnel: w542 -> [_ w549]
              frame False {
              }
              frame True {
                n225 = Send Notification(notification=w549, notifier=w550) -> ()  [unwired: 1 in, 2 out]
              }
            }
          }
          frame "clear_selection_list" {
            # "Clears all elements in the selection list. Use this before making a new selection."
            n226 = Variant To Data(error in=w562, type=T16 {"Wait Notifier"=refnum, "wait for reply"=FALSE, "vi_id"=0} ("clear_selection_list Argument"), Variant=w560) -> (data=w553:T16, error out=w551:errorcluster)
            n227 = Unbundle By Name(w553) -> ("Wait Notifier"=w558:refnum<notifier>, "wait for reply"=w557:bool)
            n228 = call "Do Clear Selection List.vi"("error in (no error)"=w551, "input cluster"=w553, "Data Cluster in"=w561) -> ("error out"=w552:errorcluster, "Data Cluster out"=w554:T3)  [unwired: 7 in]
            n229 = Bundle By Name(cluster=T51 {"error"={"status"=FALSE, "code"=0, "source"=""}} ("clear_selection_list (Reply Payload)"), "error"=w552) -> (w556:T51)
            n230 = case "DQMH_FIRE_NOTIFIER" shown="True" w557 {
              tunnel: w558 -> [_ w564]
              tunnel: w556 -> [_ w563]
              frame False {
              }
              frame True {
                n231 = Send Notification(notification=w563, notifier=w564) -> ()  [unwired: 1 in, 2 out]
              }
            }
          }
          frame "remove_from_selection" {
            # "Removes the object specified by object_id from the current selection list and returns the resulting new list."
            n232 = Variant To Data(error in=w576, type=T17 {"vi_id"=0, "object_id"=0, "Wait Notifier"=refnum, "wait for reply"=FALSE} ("remove_from_selection Argument"), Variant=w574) -> (data=w568:T17, error out=w565:errorcluster)
            n233 = Unbundle By Name(w568) -> ("Wait Notifier"=w572:refnum<notifier>, "wait for reply"=w571:bool)
            n234 = call "Do Remove From Selection.vi"("error in (no error)"=w565, "remove_from_selection Argument"=w568, "Data Cluster in"=w575) -> ("error out"=w566:errorcluster, "Data Cluster out"=w567:T3)  [unwired: 7 in]
            n235 = Bundle By Name(cluster=T52 {"current_selection"=[], "error"={"status"=FALSE, "code"=0, "source"=""}} ("remove_from_selection (Reply Payload)"), "error"=w566) -> (w570:T52)
            n236 = case "DQMH_FIRE_NOTIFIER" shown="True" w571 {
              tunnel: w572 -> [_ w578]
              tunnel: w570 -> [_ w577]
              frame False {
              }
              frame True {
                n237 = Send Notification(notification=w577, notifier=w578) -> ()  [unwired: 1 in, 2 out]
              }
            }
          }
          frame "enclose_selection" {
            # "Use this function to efficiently generate Loops or other structures around existing code. This is the quickest way to create loops including tunnles and wiring, wire the objects first, then create a loop around them, tunnles will be there automatically. Use the add_to_selection, remove_from_selection and clear_selection_list tools to change the current selection, connect_objects to connect them, then call this tool to create a structure around them.\nAllowed values for structure_type are:\nWhile Loop\nFor Loop\nCase Structure\nSequence Structure\nEvent Structure"
            n238 = Variant To Data(error in=w591, type=T18 {"vi_id"=0, "structure_type"="", "Wait Notifier"=refnum, "wait for reply"=FALSE} ("enclose_selection Argument"), Variant=w589) -> (data=w579:T18, error out=w581:errorcluster)
            n239 = Unbundle By Name(w579) -> ("Wait Notifier"=w587:refnum<notifier>, "wait for reply"=w586:bool)  [unwired: 2 out]
            n240 = call "Do Enclose Selection.vi"("error in (no error)"=w581, "enclose_selection Argument"=w579, "Data Cluster in"=w590) -> ("error out"=w582:errorcluster, "object_id"=w583:i32, "Data Cluster out"=w580:T3)  [unwired: 6 in]
            n241 = Bundle By Name(cluster=T53 {"object_id"=0, "error"={"status"=FALSE, "code"=0, "source"=""}} ("enclose_selection (Reply Payload)"), "object_id"=w583, "error"=w582) -> (w585:T53)
            n242 = case "DQMH_FIRE_NOTIFIER" shown="True" w586 {
              tunnel: w587 -> [_ w593]
              tunnel: w585 -> [_ w592]
              frame False {
              }
              frame True {
                n243 = Send Notification(notification=w592, notifier=w593) -> ()  [unwired: 1 in, 2 out]
              }
            }
          }
          frame "rename_object" {
            # "Use this to change an objects Label.Text property. Usually used for frontpanel objects. Use the label_visible True/False to decide if the label is displayed afterwards."
            n244 = Variant To Data(error in=w605, type=T19 {"new_label_name"="", "label_visible"=FALSE, "Wait Notifier"=refnum, "wait for reply"=FALSE, "object_id"=0} ("rename_object Argument"), Variant=w603) -> (data=w596:T19, error out=w594:errorcluster)
            n245 = Unbundle By Name(w596) -> ("Wait Notifier"=w601:refnum<notifier>, "wait for reply"=w600:bool)
            n246 = call "Do Rename Object.vi"("error in (no error)"=w594, "rename_object Argument"=w596, "Data Cluster in"=w604) -> ("error out"=w595:errorcluster, "Data Cluster out"=w597:T3)  [unwired: 7 in]
            n247 = Bundle By Name(cluster=T54 {"error"={"status"=FALSE, "code"=0, "source"=""}} ("rename_object (Reply Payload)"), "error"=w595) -> (w599:T54)
            n248 = case "DQMH_FIRE_NOTIFIER" shown="True" w600 {
              tunnel: w601 -> [_ w607]
              tunnel: w599 -> [_ w606]
              frame False {
              }
              frame True {
                n249 = Send Notification(notification=w606, notifier=w607) -> ()  [unwired: 1 in, 2 out]
              }
            }
          }
          frame "set_value" {
            # "Sets the value of a constant or control/indicator. The value is transferred as a string, but can be also a number."
            n250 = Variant To Data(error in=w619, type=T20 {"object_id"=0, "value"="", "Wait Notifier"=refnum, "wait for reply"=FALSE} ("set_value Argument"), Variant=w617) -> (data=w611:T20, error out=w608:errorcluster)
            n251 = Unbundle By Name(w611) -> ("Wait Notifier"=w615:refnum<notifier>, "wait for reply"=w614:bool)
            n252 = call "Do Set Value.vi"("error in (no error)"=w608, "set_value Argument"=w611, "Data Cluster in"=w618) -> ("error out"=w609:errorcluster, "Data Cluster out"=w610:T3)  [unwired: 7 in]
            n253 = Bundle By Name(cluster=T55 {"error"={"status"=FALSE, "code"=0, "source"=""}} ("set_value (Reply Payload)"), "error"=w609) -> (w613:T55)
            n254 = case "DQMH_FIRE_NOTIFIER" shown="True" w614 {
              tunnel: w615 -> [_ w621]
              tunnel: w613 -> [_ w620]
              frame False {
              }
              frame True {
                n255 = Send Notification(notification=w620, notifier=w621) -> ()  [unwired: 1 in, 2 out]
              }
            }
          }
          frame "delete_object" {
            # "removes the object from the blockdiagram or frontpanel."
            n256 = Variant To Data(error in=w633, type=T21 {"object_id"=0, "Wait Notifier"=refnum, "wait for reply"=FALSE} ("delete_object Argument"), Variant=w631) -> (data=w624:T21, error out=w622:errorcluster)
            n257 = Unbundle By Name(w624) -> ("Wait Notifier"=w629:refnum<notifier>, "wait for reply"=w628:bool)
            n258 = call "Do Delete Object.vi"("error in (no error)"=w622, "delete_object Argument"=w624, "Data Cluster in"=w632) -> ("error out"=w623:errorcluster, "Data Cluster out"=w625:T3)  [unwired: 7 in]
            n259 = Bundle By Name(cluster=T56 {"error"={"status"=FALSE, "code"=0, "source"=""}} ("delete_object (Reply Payload)"), "error"=w623) -> (w627:T56)
            n260 = case "DQMH_FIRE_NOTIFIER" shown="True" w628 {
              tunnel: w629 -> [_ w635]
              tunnel: w627 -> [_ w634]
              frame False {
              }
              frame True {
                n261 = Send Notification(notification=w634, notifier=w635) -> ()  [unwired: 1 in, 2 out]
              }
            }
          }
          frame "save_vi" {
            # "Saves a VI to the specified path. If Path is empty and vi was saved before, it saves to same location"
            n262 = Variant To Data(error in=w649, type=T22 {"vi_id"=0, "path"="", "Wait Notifier"=refnum, "wait for reply"=FALSE} ("save_vi Argument"), Variant=w646) -> (data=w640:T22, error out=w647:errorcluster)
            n263 = Unbundle By Name(w640) -> ("Wait Notifier"=w644:refnum<notifier>, "wait for reply"=w643:bool)
            n264 = call "Do Save VI.vi"("error in (no error)"=w647, "save_vi Argument"=w640, "Data Cluster in"=w648) -> ("error out"=w638:errorcluster, "VI Path"=w637:path, "Data Cluster out"=w639:T3)  [unwired: 6 in]
            n265 = Path To String(path=w637) -> (string=w636:string)
            n266 = Bundle By Name(cluster=T57 {"path_out"="", "error"={"status"=FALSE, "code"=0, "source"=""}} ("save_vi (Reply Payload)"), "path_out"=w636, "error"=w638) -> (w642:T57)
            n267 = case "DQMH_FIRE_NOTIFIER" shown="True" w643 {
              tunnel: w644 -> [_ w651]
              tunnel: w642 -> [_ w650]
              frame False {
              }
              frame True {
                n268 = Send Notification(notification=w650, notifier=w651) -> ()  [unwired: 1 in, 2 out]
              }
            }
          }
          frame "get_structure_diagram" {
            # "Returns the id of a sub-diagram of a structure (the inside of a loop or case-structure). Use this to add objects to a structure instead of to the top level blockdiagram. For Case-Structures, use the index option to iterate through them, for loops ignore index. Also consider using the \"enclose_selection\" tool if you work with structures to make wiring easier."
            n269 = Variant To Data(error in=w664, type=T23 {"structure_id"=0, "index"=0, "Wait Notifier"=refnum, "wait for reply"=FALSE} ("get_structure_diagram Argument"), Variant=w662) -> (data=w655:T23, error out=w652:errorcluster)
            n270 = Unbundle By Name(w655) -> ("Wait Notifier"=w660:refnum<notifier>, "wait for reply"=w659:bool)  [unwired: 2 out]
            n271 = call "Do Get Structure Diagram.vi"("error in (no error)"=w652, "get_structure_diagram Argument"=w655, "Data Cluster in"=w663) -> ("error out"=w653:errorcluster, "diagram_id"=w654:i32, "Data Cluster out"=w656:T3)  [unwired: 6 in]
            n272 = Bundle By Name(cluster=T58 {"diagram_id"=0, "error"={"status"=FALSE, "code"=0, "source"=""}} ("get_structure_diagram (Reply Payload)"), "diagram_id"=w654, "error"=w653) -> (w658:T58)
            n273 = case "DQMH_FIRE_NOTIFIER" shown="True" w659 {
              tunnel: w660 -> [_ w666]
              tunnel: w658 -> [_ w665]
              frame False {
              }
              frame True {
                n274 = Send Notification(notification=w665, notifier=w666) -> ()  [unwired: 1 in, 2 out]
              }
            }
          }
          frame "add_subvi" {
            # "Adds a SubVI to a blockdiagram or sturcture subdiagram similar to the add_object method."
            n275 = Variant To Data(error in=w679, type=T24 {"diagram_id"=0, "subvi_path"="", "Wait Notifier"=refnum, "wait for reply"=FALSE, "position_x"=0, "position_y"=0} ("add_subvi Argument"), Variant=w677) -> (data=w670:T24, error out=w667:errorcluster)
            n276 = Unbundle By Name(w670) -> ("Wait Notifier"=w675:refnum<notifier>, "wait for reply"=w674:bool)  [unwired: 2 out]
            n277 = call "Do Add Subvi.vi"("error in (no error)"=w667, "add_subvi Argument"=w670, "Data Cluster in"=w678) -> ("error out"=w668:errorcluster, "object_id"=w669:i32, "Data Cluster out"=w671:T3)  [unwired: 6 in]
            n278 = Bundle By Name(cluster=T59 {"subvi_id"=0, "error"={"status"=FALSE, "code"=0, "source"=""}} ("add_subvi (Reply Payload)"), "subvi_id"=w669, "error"=w668) -> (w673:T59)
            n279 = case "DQMH_FIRE_NOTIFIER" shown="True" w674 {
              tunnel: w675 -> [_ w681]
              tunnel: w673 -> [_ w680]
              frame False {
              }
              frame True {
                n280 = Send Notification(notification=w680, notifier=w681) -> ()  [unwired: 1 in, 2 out]
              }
            }
          }
          frame "connect_to_pane" {
            # "takes a control_id and connects the corresponding frontpanel control or indicator to the connector pane of the subvi. Do this to all necessary fronpanel controls/indicators to use the VI as a SubVI. The subvis by default have 4 fields on the left and right, and two on top/bottom. Their index starts at the bottom right, and goes counter clockwise."
            n281 = Variant To Data(error in=w693, type=T25 {"control_id"=0, "connector_pane_index"=0, "Wait Notifier"=refnum, "wait for reply"=FALSE} ("connect_to_pane Argument"), Variant=w691) -> (data=w684:T25, error out=w682:errorcluster)
            n282 = Unbundle By Name(w684) -> ("Wait Notifier"=w689:refnum<notifier>, "wait for reply"=w688:bool)  [unwired: 2 out]
            n283 = call "do connect to pane.vi"("error in (no error)"=w682, "connect_to_pane Argument"=w684, "Data Cluster in"=w692) -> ("error out"=w683:errorcluster, "Data Cluster out"=w685:T3)  [unwired: 7 in]
            n284 = Bundle By Name(cluster=T60 {"error"={"status"=FALSE, "code"=0, "source"=""}} ("connect_to_pane (Reply Payload)"), "error"=w683) -> (w687:T60)
            n285 = case "DQMH_FIRE_NOTIFIER" shown="True" w688 {
              tunnel: w689 -> [_ w695]
              tunnel: w687 -> [_ w694]
              frame False {
              }
              frame True {
                n286 = Send Notification(notification=w694, notifier=w695) -> ()  [unwired: 1 in, 2 out]
              }
            }
          }
          frame "get_object_help" {
            # "returns the labview detailed help article including termina descriptions. To get the exact indexes of the terminals use the get terminal info."
            n287 = Variant To Data(error in=w708, type=T26 {"object_id"=0, "Wait Notifier"=refnum, "wait for reply"=FALSE} ("get_object_help Argument"), Variant=w706) -> (data=w699:T26, error out=w697:errorcluster)
            n288 = Unbundle By Name(w699) -> ("Wait Notifier"=w704:refnum<notifier>, "wait for reply"=w703:bool)  [unwired: 1 out]
            n289 = call "Do Get Object Help.vi"("error in (no error)"=w697, "get_object_help Argument"=w699, "Data Cluster in"=w707) -> ("error out"=w696:errorcluster, "help_string"=w698:string, "Data Cluster out"=w700:T3)  [unwired: 6 in]
            n290 = Bundle By Name(cluster=T61 {"help_string"="", "error"={"status"=FALSE, "code"=0, "source"=""}} ("get_object_help (Reply Payload)"), "help_string"=w698, "error"=w696) -> (w702:T61)
            n291 = case "DQMH_FIRE_NOTIFIER" shown="True" w703 {
              tunnel: w704 -> [_ w710]
              tunnel: w702 -> [_ w709]
              frame False {
              }
              frame True {
                n292 = Send Notification(notification=w709, notifier=w710) -> ()  [unwired: 1 in, 2 out]
              }
            }
          }
          frame "get_loop_conditional_terminal" {
            # "Returns the conditional terminal of a while- or for-loop (if enabled), to be used with connect_objects (as to_object_id, with index 0)."
            n293 = Variant To Data(error in=w721, type=T27 {"loop_id"=0, "Wait Notifier"=refnum, "wait for reply"=FALSE} ("get_loop_conditional_terminal Argument"), Variant=w718) -> (data=w712:T27, error out=w719:errorcluster)
            n294 = Unbundle By Name(w712) -> ("Wait Notifier"=w716:refnum<notifier>, "wait for reply"=w715:bool)  [unwired: 1 out]
            n295 = call "Do Get Cond Terminal.vi"("error in (no error)"=w719, "get_loop_conditional_terminal Argument"=w712, "Data Cluster in"=w720) -> ("error out"=w713:errorcluster, "get_loop_conditional_terminal (Reply Payload)"=w714:T65, "Data Cluster out"=w711:T3)  [unwired: 6 in]
            n296 = case "DQMH_FIRE_NOTIFIER" shown="True" w715 {
              tunnel: w716 -> [_ w723]
              tunnel: w714 -> [_ w722]
              frame False {
              }
              frame True {
                n297 = Send Notification(notification=w722, notifier=w723) -> ()  [unwired: 1 in, 2 out]
              }
            }
          }
          frame "show_conditional_terminal" {
            # "Shows or hides the conditional terminal of a for loop."
            n298 = Variant To Data(error in=w734, type=T28 {"loop_id"=0, "show"=FALSE, "Wait Notifier"=refnum, "wait for reply"=FALSE} ("show_conditional_terminal Argument"), Variant=w731) -> (data=w725:T28, error out=w732:errorcluster)
            n299 = Unbundle By Name(w725) -> ("Wait Notifier"=w729:refnum<notifier>, "wait for reply"=w728:bool)  [unwired: 2 out]
            n300 = call "do show conditional terminal.vi"("error in (no error)"=w732, "show_conditional_terminal Argument"=w725, "Data Cluster in"=w733) -> ("error out"=w726:errorcluster, "show_conditional_terminal (Reply Payload)"=w727:T66, "Data Cluster out"=w724:T3)  [unwired: 6 in]
            n301 = case "DQMH_FIRE_NOTIFIER" shown="True" w728 {
              tunnel: w729 -> [_ w736]
              tunnel: w727 -> [_ w735]
              frame False {
              }
              frame True {
                n302 = Send Notification(notification=w735, notifier=w736) -> ()  [unwired: 1 in, 2 out]
              }
            }
          }
          frame "get_loop_iteration_terminal" {
            # "Returns the loops iteration terminal to be used for wiring."
            n303 = Variant To Data(error in=w747, type=T29 {"loop_id"=0, "Wait Notifier"=refnum, "wait for reply"=FALSE} ("get_loop_iteration_terminal Argument"), Variant=w744) -> (data=w738:T29, error out=w745:errorcluster)
            n304 = Unbundle By Name(w738) -> ("Wait Notifier"=w742:refnum<notifier>, "wait for reply"=w741:bool)  [unwired: 1 out]
            n305 = call "do get loop iteration terminal.vi"("error in (no error)"=w745, "get_loop_iteration_terminal Argument"=w738, "Data Cluster in"=w746) -> ("error out"=w739:errorcluster, "get_loop_iteration_terminal (Reply Payload)"=w740:T67, "Data Cluster out"=w737:T3)  [unwired: 6 in]
            n306 = case "DQMH_FIRE_NOTIFIER" shown="True" w741 {
              tunnel: w742 -> [_ w749]
              tunnel: w740 -> [_ w748]
              frame False {
              }
              frame True {
                n307 = Send Notification(notification=w748, notifier=w749) -> ()  [unwired: 1 in, 2 out]
              }
            }
          }
          frame "Read Config Data" {
            # "Reads the config data from the config file."
            n308 = call <vilib>:"Application Directory.vi"() -> ("Application Directory"=w758:path)
            n309 = Build Path(base path=w758, name or relative path="config.json") -> (appended path=w756:path)
            n310 = Unbundle By Name(w753) -> ("Config Data"=w752:T4)
            n311 = Read from Text File(file (use dialog)=w756, error in=w760) -> (text=w754:string, error out=w759:errorcluster)  [unwired: 2 in, 2 out]
            n312 = Unflatten From JSON(JSON string=w754, type and defaults=w752, error in (no error)=w759) -> (value=w750:T4, error out=w755:errorcluster)  [unwired: 4 in]
            n313 = Bundle By Name(cluster=w753, "Config Data"=w750) -> (w751:T3)
          }
          frame "get_allowed_paths" {
            # "Returns the Directories that the Server can write files/folders to. If you try to write to other locations you will receive an error. If asked to save to a relative path, use this function to build the full path."
            n314 = Variant To Data(error in=w772, type=T31 {"Wait Notifier"=refnum, "wait for reply"=FALSE} ("get_allowed_paths Argument"), Variant=w771) -> (data=w769:T31, error out=w761:errorcluster)
            n315 = Unbundle By Name(w764) -> ("Config Data.Allowed Paths"=w763:string[])
            n316 = Unbundle By Name(w769) -> ("Wait Notifier"=w768:refnum<notifier>, "wait for reply"=w767:bool)
            n317 = for {
              tunnel: w763 -> [w775] mode=indexing
              tunnel: [w773] -> w762 mode=concatenating
              n318 = Format Into String(format string="\"%s\", ", w775) -> (resulting string=w773:string)  [unwired: 2 in, 1 out]
            }
            n319 = Bundle By Name(cluster=T62 {"Allowed Paths"="", "error"={"status"=FALSE, "code"=0, "source"=""}} ("get_allowed_paths (Reply Payload)"), "Allowed Paths"=w762, "error"=w761) -> (w766:T62)
            n320 = case "DQMH_FIRE_NOTIFIER" shown="True" w767 {
              tunnel: w768 -> [_ w777]
              tunnel: w766 -> [_ w776]
              frame False {
              }
              frame True {
                n321 = Send Notification(notification=w776, notifier=w777) -> ()  [unwired: 1 in, 2 out]
              }
            }
          }
          frame "create_project" {
            # "Creates a new Project at the specified location"
            n322 = Variant To Data(error in=w788, type=T32 {"File Path"="", "Wait Notifier"=refnum, "wait for reply"=FALSE} ("create_project Argument"), Variant=w785) -> (data=w778:T32, error out=w786:errorcluster)
            n323 = Unbundle By Name(w778) -> ("Wait Notifier"=w783:refnum<notifier>, "wait for reply"=w782:bool)
            n324 = call "Do create project.vi"("error in (no error)"=w786, "create_project Argument"=w778, "Data Cluster in"=w787) -> ("error out"=w780:errorcluster, "create_project (Reply Payload)"=w781:T68, "Data Cluster out"=w779:T3)  [unwired: 6 in]
            n325 = case "DQMH_FIRE_NOTIFIER" shown="True" w782 {
              tunnel: w783 -> [_ w790]
              tunnel: w781 -> [_ w789]
              frame False {
              }
              frame True {
                n326 = Send Notification(notification=w789, notifier=w790) -> ()  [unwired: 1 in, 2 out]
              }
            }
          }
          frame "Set Working Directory" {
            # "Sets the allowed directory for the AI. This function shall not be exposed to the LLM."
            n327 = Variant To Data(error in=w799, type=T33 {"Working Directory Folder Path"=[]} ("Set Working Directory Argument"), Variant=w796) -> (data=w794:T33, error out=w797:errorcluster)
            n328 = Unbundle By Name(w794) -> ("Working Directory Folder Path"=w792:path[])
            n329 = Path To String(path=w792) -> (string=w791:string[])
            n330 = Bundle By Name(cluster=w798, "Config Data.Allowed Paths"=w791) -> (w793:T3)
          }
          frame "open_vi" {
            # "Opens a vi from inside the allowed paths and returns an id to further use it, similar to the new_vi tool."
            n331 = Variant To Data(error in=w810, type=T34 {"vi_path"="", "Wait Notifier"=refnum, "wait for reply"=FALSE} ("open_vi Argument"), Variant=w807) -> (data=w800:T34, error out=w808:errorcluster)
            n332 = Unbundle By Name(w800) -> ("Wait Notifier"=w805:refnum<notifier>, "wait for reply"=w804:bool)  [unwired: 1 out]
            n333 = call "Do Open Vi.vi"("error in (no error)"=w808, "open_vi Argument"=w800, "Data Cluster in"=w809) -> ("error out"=w802:errorcluster, "open_vi (Reply Payload)"=w803:T69, "Data Cluster out"=w801:T3)  [unwired: 6 in]
            n334 = case "DQMH_FIRE_NOTIFIER" shown="True" w804 {
              tunnel: w805 -> [_ w812]
              tunnel: w803 -> [_ w811]
              frame False {
              }
              frame True {
                n335 = Send Notification(notification=w811, notifier=w812) -> ()  [unwired: 1 in, 2 out]
              }
            }
          }
          frame "New MCP RPC Message" {
            # "New call from MCP client, returns request and server response. Server response may contain error for further debugging."
            n336 = Variant To Data(error in=w826, type=T35 {"request"="", "response"=""} ("New MCP RPC Message Argument"), Variant=w824) -> (data=w822:T35, error out=w825:errorcluster)
            n337 = Unbundle By Name(w822) -> ("request"=w818:string, "response"=w817:string)
            n338 = Get Date/Time In Seconds() -> (seconds since 1Jan1904=w813:timestamp)
            n339 = Unbundle By Name(w820) -> ("Log"=w816:string)
            n340 = Format Into String(format string="------------------\nNew Message:\nTimestamp: %T\nRequest:\n%s\n\n\n\nResponse:\n%s\n\n", w813, w818, w817) -> (resulting string=w814:string)  [unwired: 2 in, 1 out]
            n341 = Concatenate Strings(w816, w814) -> (w815:string)
            n342 = Bundle By Name(cluster=w820, "Log"=w815) -> (w821:T3)
          }
          frame "get-available-objects" {
            # "Returns a list of objects that can be created with the \"add object\" tool. List is mixed with frontpanel and blockdiagram objects"
            n343 = Variant To Data(error in=w838, type=T36 {"Wait Notifier"=refnum, "wait for reply"=FALSE} ("get-available-objects Argument"), Variant=w835) -> (data=w833:T36, error out=w836:errorcluster)
            n344 = Unbundle By Name(w833) -> ("Wait Notifier"=w832:refnum<notifier>, "wait for reply"=w831:bool)
            n345 = Bundle By Name(cluster=T63 {"available objects"="", "error"={"status"=FALSE, "code"=0, "source"=""}} ("get-available-objects (Reply Payload)"), "available objects"="Allowed object names are:\n.NET Container, .NET Refnum, 2D Picture, 3D Picture, Absolute Value, Accept TLS, Access Rights, ActiveX Container, Add, Add (with error terminals), Add Array Elements, Add Entropy, Add Private Key To TLS Configuration, Add Trusted Certificate To TLS Configuration, Agitator, AllSpoll, Always Copy, And, And Array Elements, Append True/False String, Application Refnum, Array (block diagram constant), Array (classic), Array (modern), Array Interface Control, Array Max & Min, Array of Strings to Path, Array Size, Array Subset, Array To Cluster, Array To Spreadsheet String, ArrayMemInfo, Assert Structural Type Match, Assert Structural Type Mismatch, Atmospheric Tank (classic), Atmospheric Tank (modern), Automation Close, Automation Open, Automation Refnum, Avogadro Constant (1/mol), Base 10 Logarithm Of e, Bin #1, Bin #2, Bitpack to Array, Bluetooth Close Connection, Bluetooth Create Listener, Bluetooth Discover, Bluetooth Network Connection Refnum, Bluetooth Open Connection, Bluetooth Read, Bluetooth Wait On Listener, Bluetooth Write, Boolean Array To Number, Boolean To (0,1), Build Array, Build Cluster Array, Build Map, Build Matrix, Build Path, Build Set, Build Waveform, Bundle, Bundle By Name, Byte Array To String, Byte Array To UTF-8 String, Byte Stream File Refnum, Call By Reference, Call Chain, Call Library Function Node, Call MATLAB Function, Call Parent Class Method, CAN Channel (block diagram constant), CAN Channel (classic), CAN Channel (modern), CAN Channel (system), CAN Interface (block diagram constant), CAN Interface (classic), CAN Interface (modern), CAN Interface (system), CAN Task (block diagram constant), CAN Task (classic), CAN Task (modern), CAN Task (system), Cancel Button (modern), Cancel Button (system), Cancel Notification, Carriage Return Constant, Case Structure, Cast Unit Bases, Check Valve, Checkbox (classic), CheckBox (modern), Checkbox (system), Class Specifier Constant, Classic Color Box, Classic Color Ramp, Classic Horizontal Slide Switch, Classic Vertical Slide, Clear Fixed-Point Overflow Status, Close File, Close File (deprecated), Close MATLAB Session, Close Python Session, Close Reference, Close TLS Configuration, Close Variable Connection, Closure Structure, Cluster (classic), Cluster (modern), Cluster Constant, Cluster To Array, Code Interface Node, Coerce To Type, Collection Size, Color Box Constant, Color Box Thin Border, Colored Rectangle (broken?), Combo Box (classic), Combo Box (modern), Combo Box (system), Combo Box Constant, Complex Conjugate, Complex To Polar, Complex To Re/Im, Compound Arithmetic, Compressor, Concatenate Strings, Conditional Disable Structure, Constructor Node, Control & Simulation Loop, Control Help Window, Control Online Help, Control Refnum, Convert Unit, Conveyer, Copy, Copy (deprecated), Cosecant, Cosine, Cotangent, CPU Information, Create Folder, Create Network Stream Endpoint, Create Network Stream Reader Endpoint, Create Network Stream Writer Endpoint, Create Stream, Create Unique Network Stream Endpoint, Create Unique Network Stream Reader Endpoint, Create Unique Network Stream Writer Endpoint, Create User Event, Current Processor ID, Current VI's Menubar, Current VI's Path, DAQmx Analog Trigger Source (block diagram constant), DAQmx Analog Trigger Source (classic), DAQmx Analog Trigger Source (modern), DAQmx Analog Trigger Source (system), DAQmx Device Name (block diagram constant), DAQmx Device Name (classic), DAQmx Device Name (modern), DAQmx Device Name (system), DAQmx Global Channel (block diagram constant), DAQmx Global Channel (classic), DAQmx Global Channel (modern), DAQmx Global Channel (system), DAQmx Physical Channel (block diagram constant), DAQmx Physical Channel (classic), DAQmx Physical Channel (modern), DAQmx Physical Channel (system), DAQmx Scale Name (block diagram constant), DAQmx Scale Name (classic), DAQmx Scale Name (modern), DAQmx Scale Name (system), DAQmx Switch (block diagram constant), DAQmx Switch (classic), DAQmx Switch (modern), DAQmx Switch (system), DAQmx Task Name (block diagram constant), DAQmx Task Name (classic), DAQmx Task Name (modern), DAQmx Task Name (system), DAQmx Terminal (block diagram constant), DAQmx Terminal (classic), DAQmx Terminal (modern), DAQmx Terminal (system), Data Cache Size, Data Log File Refnum, Data Value Reference, Data Value Reference Constant, DataSocket Close, DataSocket Open, DataSocket Read, DataSocket Refnum, DataSocket Write, Date/Time To Seconds, Decimal Digit?, Decimal String To Number, Decimate 1D Array, DecomposeLockDataValRef, DecomposeVariant, Decrement, Default Directory, Delete, Delete (deprecated), Delete Data Value Reference, Delete From Array, Delete Menu Items, Delete Variant Attribute, Delete Waveform Attribute, Deny Access, Dequeue Element, Destroy Stream Endpoint, Destroy User Event, DevClear, DevClearList, Device Control/Status, Device Refnum, Diagram Disable Structure, Dial (classic), Dial (modern), Digital Data (classic), Digital Data (modern), Digital Waveform Graph (classic), Digital Waveform Graph (modern), Direct Variable Read, Direct Variable Write, Divide, Divide (with error terminals), Dlg Horiz Scrollbar, Dlg Mac Group Box, Dlg Numeric #1, Dlg Numeric #2, Dlg String, Dlg Vert Scrollbar, Down Arrow, Down Bow Valve (flat), Down Bow Valve (outline), Down Bow Valve (shaded), Down Rect Valve (flat), Down Rect Valve (outline), Down Rect Valve (shaded), Down Tee (flat), Down Tee (shaded), Dynamic FPGA Interface Cast, Eased Corner Rectangle, Element of Set?, Elementary Charge (C), Empty Array?, Empty Collection?, Empty Path Constant, Empty String Constant, Empty String/Path?, Enable Menu Tracking, EnableLocal, EnableRemote, End of Line Constant, Enqueue Element, Enqueue Element At Opposite End, Enum (classic), Enum (modern), Enum (system), Enum Constant, EOF, Equal To 0?, Equal?, Error Ring Constant, Event Callback Refnum, Event Data Node, Event Structure, Exchanger, Exclusive Or, Exponential, Exponential (Arg) -1, Expression Node, False Constant, Feedback Node, FieldPoint IO Point (block diagram constant), FieldPoint IO Point (classic), FieldPoint IO Point (modern), FIFO Refnum, File Dialog, File Dialog (deprecated), File Path Control (classic), File Path Control (modern), File Path Control (system), File Path Indicator (classic), File Path Indicator (modern), File/Directory Info, File/Directory Info (deprecated), FindLstn, FindRQS, First Call?, Fixed-Point Overflow?, Fixed-Point to Integer Cast, Flat Box, Flat Circle, Flat Down Triangle, Flat Frame, Flat Left Triangle, Flat Right Triangle, Flat Round Button, Flat Rounded Box, Flat Sequence Structure, Flat Square Button, Flat Up Triangle, Flatten To JSON, Flatten To String, Flatten To XML, Flattened String To Variant, Floating Point Equal?, Flush Event Queue, Flush File, Flush File (deprecated), Flush Queue, Flush Stream, For Loop, Fork, Format Date/Time String, Format Into File, Format Into String, Format Value, Formula Node, FPGA Refnum to Session, Fract/Exp String To Number, Framed Color Box (classic), Framed Color Box (modern), Free Label, Furnace, Gauge (classic), Gauge (modern), Gauge for Simon, Generate Front Panel Activity, Generate Occurrence, Generate User Event, Generate User-Defined Trace Event, Get Control Values by Index, Get Datalog Position, Get Date/Time In Seconds, Get Date/Time String, Get Drag Drop Data, Get File Position, Get File Size, Get Fixed-Point Components, Get Help Window Status, Get Matrix Diagonal, Get Matrix Elements, Get Menu Item Info, Get Menu Selection, Get Menu Short Cut Info, Get Notifier Status, Get Number of Records, Get Permissions, Get Queue Status, Get Submatrix, Get Type and Creator, Get Variant Attribute, Get Volume Info, Get Waveform Attribute, Get Waveform Components, Global Variable, GPIB Clear, GPIB Initialization, GPIB Misc, GPIB Read, GPIB Serial Poll, GPIB Status, GPIB Trigger, GPIB Wait, GPIB Write, Gravitational Constant (N m2/kg2), Greater Or Equal To 0?, Greater Or Equal?, Greater Than 0?, Greater?, Handle Peek, Handle Poke, Hex Digit?, Hexadecimal String To Number, Hopper #1, Hopper #2, Horiz Line, Horiz Pipe (flat), Horiz Pipe (shaded), Horizontal Button Box, Horizontal Fill Slide (classic), Horizontal Fill Slide (modern), Horizontal Gradient Oval, Horizontal Gradient Rectangle, Horizontal Gradient Rounded Rectangle, Horizontal Graduated Bar, Horizontal Pointer Slide (classic), Horizontal Pointer Slide (modern), Horizontal Pointer Slide (system), Horizontal Progress Bar (modern), Horizontal Progress Bar (system), Horizontal Scrollbar, Horizontal Slide (classic), Horizontal Slide (system), Horizontal Smooth Box, Horizontal Splitter Bar, Horizontal Splitter Bar (Classic), Horizontal Splitter Bar (NXG Style), Horizontal Splitter Bar (System), Horizontal Switch, Horizontal Tank, Horizontal Toggle Switch (classic), Horizontal Toggle Switch (modern), Hyperbolic Cosecant, Hyperbolic Cosine, Hyperbolic Cotangent, Hyperbolic Secant, Hyperbolic Sine, Hyperbolic Tangent, IMAQ Session, Implies, In Place Element Structure, In Range and Coerce, Include Fixed-Point Overflow Status, Increment, Index & Bundle Cluster Array, Index Array, Index String Array, Initialize Array, Inline C Node, Insert Into Array, Insert Into Map, Insert Into Set, Insert Menu Items, Integer to Fixed-Point Cast, Intensity Chart (classic), Intensity Chart (modern), Intensity Graph (classic), Intensity Graph (modern), Interleave 1D Arrays, Interpolate 1D Array, Inverse Cosecant, Inverse Cosine, Inverse Cotangent, Inverse Hyperbolic Cosecant, Inverse Hyperbolic Cosine, Inverse Hyperbolic Cotangent, Inverse Hyperbolic Secant, Inverse Hyperbolic Sine, Inverse Hyperbolic Tangent, Inverse Secant, Inverse Sine, Inverse Tangent, Inverse Tangent (2 Input), Invoke Node, IP To String, IrDA Close Connection, IrDA Create Listener, IrDA Discover, IrDA Network Connection Refnum, IrDA Open Connection, IrDA Read, IrDA Wait On Listener, IrDA Write, IsDebuggingActive, IVI Delete Session, IVI Logical Name (block diagram constant), IVI Logical Name (classic), IVI Logical Name (modern), IVI New Session, Join, Join Numbers, Junction, Knob (classic), Knob (modern), Label (modern), Label (system), Labeled Oblong Button, Labeled Rectangular Button, Labeled Round Button, Labeled Square Button, LabVIEW Object, Leak Variant Value Reference, LED Button, Left Arrow, Left Bow Valve (flat), Left Bow Valve (outline), Left Bow Valve (shaded), Left Down Elbow (flat), Left Down Elbow (shaded), Left Pump (flat), Left Pump (shaded), Left Rect Valve (flat), Left Rect Valve (outline), Left Rect Valve (shaded), Left Tee (flat), Left Tee (shaded), Left Up Elbow (flat), Left Up Elbow (shaded), Less Or Equal To 0?, Less Or Equal?, Less Than 0?, Less?, Lexical Class, Line (chiseled, system), Line (chiseled, thick), Line (chiseled, thin), Line (thick), Line (thin), Line Feed Constant, Line with Arrow (thick), Line with Arrow (thin), List Directory, List Folder, Listbox (classic), Listbox (modern), Listbox (system), Listbox Symbol Ring Constant, Load Certificates Into Memory, Load Private Key Into Memory, Local Variable, Lock Range, Logarithm Base 10, Logarithm Base 2, Logarithm Base X, Logical Shift, Look In Map, Lookup Channel Probe, Lossy Enqueue Element, Lowered Box (thick), Lowered Rounded Box, Machine Epsilon, Make TLS Configuration Immutable, MakeAddr, Mantissa & Exponent, Map, Map Constant, Match First String, Match Pattern, Match True/False String, MathScript Call By Reference, MathScript Node, MATLAB script, MATLAB Session Refnum, Matrix Size, Max & Min, Menu Refnum, Menu Ring (classic), Menu Ring (modern), Menu-Popup Ring, Merge Errors, Merge Signals, Meter (classic), Meter (modern), Mixed Checkbox (system), Mixed Signal Graph, Molar Gas Constant (J/(mol K)), Motion Resource (block diagram constant), Motion Resource (classic), Motion Resource (modern), Motor (flat), Motor (shaded), Move, Move (deprecated), Multi-Segment Pipe, Multicolumn Listbox (classic), Multicolumn Listbox (modern), Multicolumn Listbox (system), Multiply, Multiply (with error terminals), Multiply Array Elements, Multirate Structure, Natural Logarithm, Natural Logarithm (Arg +1), Natural Logarithm Base, Natural Logarithm Of 10, Natural Logarithm Of 2, Natural Logarithm Of Pi, Negate, Negative Infinity, New Data Value Reference, New Directory, New File, New TLS Configuration, New VI, New VI Object, Not, Not A Number/Path/Refnum?, Not A Path Constant, Not a Refnum Constant, Not a Shared Variable, Not And, Not Equal To 0?, Not Equal?, Not Exclusive Or, Not Or, Notifier Refnum, Number of Cache Levels, Number To Boolean Array, Number To Decimal String, Number To Engineering String, Number To Exponential String, Number To Fractional String, Number To Hexadecimal String, Number To Octal String, Numeric Constant, Numeric Control (classic), Numeric Control (modern), Numeric Control (system), Numeric Indicator (classic), Numeric Indicator (modern), Obtain Notifier, Obtain Queue, Occurrence Refnum, Octal Digit?, Octal String To Number, OK Button (modern), OK Button (system), Old VISA Open, OLE Variant, One Button Dialog, Open and Verify Variable Connection, Open Application Reference, Open Device, Open Dynamic Bitfile Reference, Open File, Open MATLAB Session, Open Python Session, Open Tank (flat classic), Open Tank (shaded classic), Open Variable Connection, Open Variable Connection in Background, Open VI Object Reference, Open VI Reference, Open/Create/Replace Datalog, Open/Create/Replace File, Or, Or Array Elements, Oval with Shadow, Package Matrix, PassControl, Path Constant, Path to Array of Strings, Path To String, Path Type, Pi, Pi Divided By 2, Pi Multiplied By 2, Pick Line, Pict Ring (classic), Pict Ring (modern), Pict Ring (system), PixMap, PixMap (warning: dangerous), Planck's Constant (J/Hz), Platform Flat Square Button, Plug-In Control, Polar To Complex, Polar To Re/Im, Positive Infinity, Power Of 10, Power Of 2, Power Of X, PPoll, PPollConfig, PPollUnconfig, Preallocated Read from Binary File, Preserve Run-Time Class, Pressure Tank (flat), Pressure Tank (shaded), Preview Queue Element, Printable?, Property Node, Pulldown Menu Ring, Push Button, Python Node, Python Session Refnum, Queue Refnum, Quit LabVIEW, Quotient & Remainder, Race Structure, Radio Button (system), Radio Buttons (classic), Radio Buttons (modern), Radio Buttons (system), Raised Box (classic), Raised Box (modern), Raised Circle, Raised Down Triangle, Raised Frame, Raised Left Triangle, Raised Right Triangle, Raised Rounded Box, Raised Up Triangle, Random Number (0-1), RcvRespMsg, Re-accept TLS, Re/Im To Complex, Re/Im To Polar, Read Datalog, Read Device, Read File, Read from Binary File, Read from Text File, Read Map Max & Min Keys, Read Multiple Elements from Stream, Read Set Max & Min, Read Single Element from Stream, Read Variable, Read Variable with Timeout, ReadStatus, Receive, ReceiveSetup, Recessed Box, Recessed Circle, Recessed Down Triangle, Recessed Frame (modern), Recessed Frame (system), Recessed Left Triangle, Recessed Menu Ring, Recessed Right Triangle, Recessed Rounded Box, Recessed Up Triangle, Reciprocal, Reciprocal Of e, Reciprocal Of Pi, RecomposeUnlockDataValRef (warning: dangerous), RecomposeVariant (warning: dangerous), Rectangular Stop Button, Refnum to Path, Refnum to Session, Region, Register Event Callback, Register For Events, Register Session, Release Notifier, Release Queue, Remove Fixed-Point Overflow Status, Remove From Map, Remove From Set, Replace Array Subset, Replace Substring, Request Deallocation, ResetSys, Reshape Array, Resize Matrix, Resource Index, Reverse 1D Array, Reverse String, Right Arrow, Right Bow Valve (flat), Right Bow Valve (outline), Right Bow Valve (shaded), Right Down Elbow (flat), Right Down Elbow (shaded), Right Pump (flat), Right Pump (shaded), Right Rect Valve (flat), Right Rect Valve (outline), Right Rect Valve (shaded), Right Tee (flat), Right Tee (shaded), Right Up Elbow (flat), Right Up Elbow (shaded), Rocker, Rotary Feeder, Rotate, Rotate 1D Array, Rotate Left With Carry, Rotate Right With Carry, Rotate String, Round Button, Round LED (classic), Round LED (modern), Round Light, Round Push Button, Round Push Button (profile), Round Radio Button, Round Stop Button, Round To Nearest, Round Toward +Infinity, Round Toward -Infinity, Rounded Rectangle with Shadow, RT FIFO Create, RT FIFO Delete, RT FIFO Read, RT FIFO Write, Rydberg Constant (1/m), Scale By Power Of 2, Scan From File, Scan From String, Scan String For Tokens, Scan Value, Scanned Variable Read, Scanned Variable Write, Search 1D Array, Search and Replace String, Search Variable Container, Search/Split String, Secant, Seconds To Date/Time, Seek, Select, Send, Send Notification, SendCmds, SendDataBytes, SendIFC, SendList, SendLLO, SendSetup, Session to Refnum, Set, Set Constant, Set Control Values by Index, Set Datalog Position, Set File Position, Set File Size, Set Matrix Diagonal, Set Matrix Elements, Set Menu Item Info, Set Number of Records, Set Occurrence, Set Permissions, Set Submatrix, Set Type and Creator, Set Variant Attribute, Set Waveform Attribute, SetRWLS, SetTimeOut, Shared Variable, Shared Variable Constant, Shared Variable Control (classic), Shared Variable Control (modern), Shared Variable to String, Sign, Simple Horizontal Slide, Simple Numeric, Simple String, Simple Vertical Slide, Sinc, Sine, Sine & Cosine, Size Handle, Slide Switch, Smoothed Oval, Smoothed Rounded Rectangle, Sort 1D Array, Sort Array of String, Speed Of Light In Vacuum (m/sec), Spin Control (system), Split 1D Array, Split Button, Split Number, Split Signals, Spreadsheet String To Array, Square, Square Button, Square LED (classic), Square LED (modern), Square Light, Square Push Button, Square Push Button (profile), Square Radio Button, Square Root, Stacked Sequence Structure, Start TLS, State, State Diagram, Static VI Reference, Stop, Stop Button, String Constant, String Control (classic), String Control (modern), String Control (system), String Indicator (classic), String Indicator (modern), String Length, String Subset, String To Byte Array, String To IP, String To Path, String to Shared Variable, Strip Path, SubPanel, SubPanel (Classic), SubPanel (NXG Style), SubPanel (System), Subtract, Subtract (with error terminals), Swap Bytes, Swap Values, Swap Vector Element, Swap Words, Tab Constant, Tab Control (classic), Tab Control (modern), Tab Control (NXG Style), Tab Control (system), Table (classic), Table (modern), Table (system), Tag Attribute Ring, Tangent, Tank (classic), Tank (modern), Target Structure, TCP Close Connection, TCP Create Listener, TCP Flattened Read, TCP Flattened Write, TCP Flex Read, TCP Flex Write, TCP Network Connection Refnum, TCP Open Connection, TCP Read, TCP Wait On Listener, TCP Write, TDMS Advanced Asynchronous Read (Data Ref), TDMS Advanced Asynchronous Write (Data Ref), TDMS Close, TDMS Configure Asynchronous Reads (Data Ref), TDMS Configure Asynchronous Writes (Data Ref), TDMS Defragment, TDMS Delete Data, TDMS File, TDMS Flush, TDMS Get Asynchronous Read Status (Data Ref), TDMS Get Asynchronous Write Status (Data Ref), TDMS Get Properties, TDMS In Memory Close, TDMS In Memory Open, TDMS In Memory Read Bytes, TDMS List Contents, TDMS Open, TDMS Read, TDMS Refnum To File ID, TDMS Set Properties, TDMS Write, TDMS Write IP, Temporary Directory, TestSRQ, TestSys, Text & Pict Ring (classic), Text & Pict Ring (modern), Text Button, Text Ring (block diagram constant), Text Ring (classic), Text Ring (modern), Text Ring (system), Text to UTF-8, Thermometer (classic), Thermometer (modern), Threshold 1D Array, Tick Count (ms), Time Stamp (block diagram constant), Time Stamp Control (classic), Time Stamp Control (modern), Time Stamp Control (system), Time Stamp Indicator (classic), Time Stamp Indicator (modern), Timed Loop, Timed Sequence, TLS configuration, TLS Connection?, To Byte Integer, To Double Precision Complex, To Double Precision Float, To Extended Precision Complex, To Extended Precision Float, To Fixed-Point, To Long Integer, To Lower Case, To More Generic Class, To More Specific Class, To OLE Variant, To Probe String, To Quad Integer, To Single Precision Complex, To Single Precision Float, To Time Stamp, To Unsigned Byte Integer, To Unsigned Long Integer, To Unsigned Quad Integer, To Unsigned Word Integer, To Upper Case, To Variant, To Word Integer, Traditional DAQ Channel (block diagram constant), Traditional DAQ Channel (classic), Traditional DAQ Channel (modern), Transpose 1D Array, Transpose 2D Array, Transpose Matrix, Tree (classic), Tree (modern), Tree (system), Trigger, TriggerList, Two Button Dialog, Type and Creator, Type Cast, Type Error, Type Must Be Array, Type Must Be Cluster, Type Of, Type Specialization Structure, UDP Close, UDP Multicast Open, UDP Network Connection Refnum, UDP Open, UDP Read, UDP Write, Unbitpack from Array, Unbundle, Unbundle By Name, Unflatten From JSON, Unflatten From String, Unflatten From XML, Unleak Variant Value Reference, Unpackage Matrix, Unregister For Events, Unregister Session, Up Arrow, Up Bow Valve (flat), Up Bow Valve (outline), Up Bow Valve (shaded), Up Rect Valve (flat), Up Rect Valve (outline), Up Rect Valve (shaded), Up Tee (flat), Up Tee (shaded), User Defined Refnum, User Defined Refnum Tag (block diagram constant), User Defined Refnum Tag (classic), User Defined Refnum Tag (modern), User Defined Refnum Tag Flatten (classic), User Defined Refnum Tag Flatten (modern), User Defined Tag (block diagram constant), User Defined Tag (classic), User Defined Tag (modern), User Item, UTF-8 String To Byte Array, UTF-8 to Text, Variable Class Specifier Constant, Variable Name Constant, Variant, Variant To Data, Variant To Flattened String, Vert Line, Vert Pipe (flat), Vert Pipe (shaded), Vert Rocker, Vertical Fill Slide (classic), Vertical Fill Slide (modern), Vertical Gradient Oval, Vertical Gradient Rectangle, Vertical Gradient Rounded Rectangle, Vertical Graduated Bar, Vertical Pointer Slide (classic), Vertical Pointer Slide (modern), Vertical Pointer Slide (system), Vertical Progress Bar (modern), Vertical Progress Bar (system), Vertical Scrollbar, Vertical Slide (system), Vertical Slide Switch (classic), Vertical Slide Switch (modern), Vertical Smooth Box, Vertical Splitter Bar, Vertical Splitter Bar (Classic), Vertical Splitter Bar (NXG Style), Vertical Splitter Bar (System), Vertical Switch, Vertical Toggle Switch (classic), Vertical Toggle Switch (modern), VI Library, VI Refnum, VI Server Reference, VISA Assert Interrupt Signal, VISA Assert Trigger, VISA Assert Utility Signal, VISA Clear, VISA Close, VISA Disable Event, VISA Discard Events, VISA Enable Event, VISA Find Resource, VISA Flush I/O Buffer, VISA GPIB Command, VISA GPIB Control ATN, VISA GPIB Control REN, VISA GPIB Pass Control, VISA GPIB Send IFC, VISA In 16, VISA In 32, VISA In 64, VISA In 8, VISA Lock, VISA Map Address, VISA Map Trigger, VISA Memory Allocation, VISA Memory Allocation Ex, VISA Memory Free, VISA Move, VISA Move In 16, VISA Move In 32, VISA Move In 64, VISA Move In 8, VISA Move Out 16, VISA Move Out 32, VISA Move Out 64, VISA Move Out 8, VISA Open, VISA Out 16, VISA Out 32, VISA Out 64, VISA Out 8, VISA Peek 16, VISA Peek 32, VISA Peek 64, VISA Peek 8, VISA Poke 16, VISA Poke 32, VISA Poke 64, VISA Poke 8, VISA Read, VISA Read STB, VISA Read To File, VISA Refnum to Session, VISA Resource Name, VISA resource name (classic), VISA resource name (modern), VISA Set I/O Buffer Size, VISA Status Description, VISA Unlock, VISA Unmap Address, VISA Unmap Trigger, VISA USB Control In, VISA USB Control Out, VISA VXI Cmd or Query, VISA Wait on Event, VISA Write, VISA Write From File, Volume Info, Wait (ms), Wait For Activity, Wait For Front Panel Activity, Wait for GPIB RQS, Wait on Notification, Wait on Notification from Multiple, Wait on Notification from Multiple with Notifier History, Wait on Notification with Notifier History, Wait on Occurrence, Wait Until Next ms Multiple, WaitSRQ, Waveform Chart, Waveform Chart (classic), Waveform Chart (modern), Waveform Graph (classic), Waveform Graph (modern), While Loop #1, While Loop #2, White Space?, Write Datalog, Write Device, Write File, Write Multiple Elements to Stream, Write Single Element to Stream, Write to Binary File, Write to Text File, Write Variable, Write Variable with Timeout, XY Graph (classic), XY Graph (modern), Y-th Root of X") -> (w830:T63)
            n346 = Merge Errors(w836) -> (w828:errorcluster)
            n347 = case "DQMH_FIRE_NOTIFIER" shown="True" w831 {
              tunnel: w832 -> [_ w840]
              tunnel: w830 -> [_ w839]
              frame False {
              }
              frame True {
                n348 = Send Notification(notification=w839, notifier=w840) -> ()  [unwired: 1 in, 2 out]
              }
            }
          }
          frame "Get open VIs" {
            # "Returns a list of currently open VIs."
            n349 = Variant To Data(error in=w848, type=T37 {"Wait Notifier"=refnum, "wait for reply"=FALSE} ("Get open VIs Argument"), Variant=w846) -> (data=w841:T37, error out=w847:errorcluster)
            n350 = call "Do Get Open VIs.vi"("error in (no error)"=w847, "Get open VIs Argument"=w841, "Data Cluster 2"=w842) -> ("error out"=w844:errorcluster, "Data Cluster"=w843:T3)  [unwired: 7 in]
          }
          frame "Get VI Blockdiagram" {
            # "Returns a picture of the block diagram of a VI"
            n351 = Variant To Data(error in=w856, type=T38 {"VI ID"=0, "Wait Notifier"=refnum, "wait for reply"=FALSE} ("Get VI Blockdiagram Argument"), Variant=w853) -> (data=w851:T38, error out=w854:errorcluster)
            n352 = call "Do Get VI Blockdiagram.vi"("error in (no error)"=w854, "Get VI Blockdiagram Argument"=w851, "Data Cluster in"=w855) -> ("error out"=w850:errorcluster, "Data Cluster out"=w849:T3)  [unwired: 7 in]
          }
          frame "Get VI Frontpanel Picture" {
            # "returns a picture of the VIs frontpanel specified by ID."
            n353 = Variant To Data(error in=w864, type=T39 {"VI ID"=0, "Wait Notifier"=refnum, "wait for reply"=FALSE} ("Get VI Frontpanel Picture Argument"), Variant=w861) -> (data=w859:T39, error out=w862:errorcluster)
            n354 = call "Do Get VI Frontpanel Picture.vi"("error in (no error)"=w862, "Get VI Frontpanel Picture Argument"=w859, "Data Cluster in"=w863) -> ("error out"=w858:errorcluster, "Data Cluster out"=w857:T3)  [unwired: 7 in]
          }
          frame "Get Library" {
            # "Returns the xml-content of a LabVIEW Project of Library file specified by full file-path. To get a full projects multiple calls may be necessary to get all nested libraries."
            n355 = Variant To Data(error in=w875, type=T40 {"Library Path"="", "Wait Notifier"=refnum, "wait for reply"=FALSE} ("Get Library Argument"), Variant=w873) -> (data=w868:T40, error out=w874:errorcluster)
            n356 = Unbundle By Name(w868) -> ("Wait Notifier"=w871:refnum<notifier>, "wait for reply"=w870:bool)
            n357 = call "Do Get Library.vi"("error in (no error)"=w874, "Get Library Argument"=w868, "Data Cluster"=w866) -> ("error out"=w869:errorcluster, "Get Library (Reply Payload)"=w867:T70, "Data Cluster 2"=w865:T3)  [unwired: 6 in]
            n358 = case "DQMH_FIRE_NOTIFIER" shown="True" w870 {
              tunnel: w871 -> [_ w877]
              tunnel: w867 -> [_ w876]
              frame False {
              }
              frame True {
                n359 = Send Notification(notification=w876, notifier=w877) -> ()  [unwired: 1 in, 2 out]
              }
            }
          }
          frame "---Copy This Frame---" {
            # "Duplicate this frame when creating new messages.  Change this comment in the duplicated frame to describe this message."
            n360 = Merge Errors(w880) -> (w879:errorcluster)
          }
          frame "---Exit and Error Handling---" {
            # "Separator - The following cases handle errors and exit messages."
          }
          frame "Simulate MHL Error" {
            # "#DQMH_HowTo The 'Simulate MHL Error' button  illustrates how the MHL handles errors. This event is instructional in nature and can be removed."
            # "Simulate an error occurring at the MHL"
            n361 = call "Module Name--constant.vi"() -> ("Module Name"=w884:string)  [unwired: 11 in]
            n362 = Format Into String(format string="Simulated error originating at Message Handling Loop in %s", w884) -> (resulting string=w885:string)  [unwired: 2 in, 1 out]
            n363 = call <vilib>:"Error Cluster From Error Code.vi"("show call chain? (False)"=TRUE, "error message (\"\")"=w885, "error code (0)"=5001) -> ("error out"=w889:errorcluster)  [unwired: 6 in]
            n364 = Merge Errors(w891, w889) -> (w890:errorcluster)
          }
          frame "Error" {
            # "#DQMH_CodeRecommended - If the module is running in standalone mode (External Launch = FALSE), this code will pop up an error dialog and call the 'Exit' message if an error occurs. Add more fine-grained error management here."
            # "Error - Check the error message data and respond accordingly. This message is sent by the \"Error Handler\" VIs at the end of each loop in this application."
            n365 = Variant To Data(error in=w902, type=errorcluster {"status"=FALSE, "code"=0, "source"=""} ("error constant"), Variant=w896) -> (data=w892:errorcluster, error out=w900:errorcluster)
            n366 = property on="Property Node" class="Module Admin"(reference=w894) -> ("Accessors:External Launch"=w893:bool)  [unwired: 1 in, 2 out]
            n367 = local write "error out"(w892) -> ()
            n368 = call "Error Reported.vi"("Error"=w892) -> ()  [unwired: 10 in, 1 out]
            n369 = case shown="False" w893 {
              tunnel: [w907 _] -> w899
              tunnel: w895 -> [w905 _]
              tunnel: w892 -> [w906 _]
              frame False {
                n370 = disable-structure shown="Default" {
                  disable-tunnel: w906 -> [w908 _]
                  frame condition #0 (active) {
                    # "If the module is running standalone, then pop up an error dialog and call the \"Exit\" message."
                    n371 = call <vilib>:"Simple Error Handler.vi"("error in (no error)"=w908) -> ()  [unwired: 4 in, 5 out]
                  }
                  frame condition #1 {
                    # "To prevent the Simple Error Handler VI from being loaded (e.g. when deploying to a Real-Time target), add the Conditional Disable Symbol \"DQMH_Disable_SEH\" to your project and set it to TRUE."
                  }
                }
                n372 = call-poly <vilib>:"Delacor_lib_QMH_Enqueue Message (poly).vi"("Priority Message? (F)"=TRUE, "Message"="Exit", "Message Queue in"=w905) -> ("error out"=w907:errorcluster)  [unwired: 7 in, 1 out]
              }
              frame True {
                # "If the module was launched externally, calling the Error Reported broadcast VI is the only action performed by the \"Error\" message. The module's caller can then process the error appropriately."
              }
            }
            n373 = Merge Errors(w900, w899) -> (w898:errorcluster)
          }
          frame "Exit" {
            w917 = 91  # 91: not all Exit messages will have an argument
            w919 = TRUE  # Stop the VI
            # "Release the message queue reference"
            # "Exit - Exit the application."
            n374 = Variant To Data(error in=w925, type=T6 {"Origin"="", "Exit via Stop Module Req?"=FALSE, "Wait for Module to stop?"=FALSE} ("Stop Argument"), Variant=w918) -> (data=w915:T6, error out=w922:errorcluster)
            n375 = call <vilib>:"Clear Errors.vi"("error in (no error)"=w922, "specific error code to clear (0: all)"=w917) -> ("error out"=w924:errorcluster)  [unwired: 4 in, 1 out]
            n376 = control-ref of="This VI"() -> (w914:refnum<vi>)
            n377 = call-dynamic "Delacor_lib_QMH_Release Message Queue.vi"("error in"=w924, "Message Queue"=w920) -> ("error out"=w923:errorcluster)  [unwired: 9 in]
            n378 = call "Handle Exit.vi"("Stop Argument"=w915, "Admin in"=w913, "VI reference"=w914) -> ("error out"=w921:errorcluster)  [unwired: 7 in, 1 out]
            n379 = Merge Errors(w923, w921) -> (w910:errorcluster)
            n380 = call "Error Reported.vi"("Error"=w910) -> ()  [unwired: 10 in, 1 out]
            n381 = Unbundle By Name(w912) -> ("MCP id"=w911:i32)
            n382 = call <vilib>:"Stop.vi"("error in (no error)"=w910, "id"=w911) -> ("error out"=w909:errorcluster)  [unwired: 9 in]
          }
          frame Default {
            # "'Default' case only runs if there is a message that isn't defined in any of the other cases.  Output a programming error."
            n383 = call "Module Name--constant.vi"() -> ("Module Name"=w930:string)  [unwired: 11 in]
            n384 = Format Into String(format string="The invalid message string \"%s\" was received in the Message Handling Loop for module \"%s\".", w931, w930) -> (resulting string=w926:string)  [unwired: 2 in, 1 out]
            n385 = call <vilib>:"Error Cluster From Error Code.vi"("show call chain? (False)"=TRUE, "error message (\"\")"=w926, "error code (0)"=1) -> ("error out"=w933:errorcluster)  [unwired: 6 in]
            n386 = Merge Errors(w934, w933) -> (w935:errorcluster)
          }
        }
        n387 = Unbundle By Name(w381) -> ("Log"=→"Log":string)
        n388 = call-dynamic "Delacor_lib_QMH_Error Handler - Message Handling Loop.vi"("error in"=w384, "Message Queue in"=w383) -> ("dup error in"=w385:errorcluster)  [unwired: 8 in, 1 out]
      }
    }
    frame Error {
      # "Synchronize Caller Events.vi will inform Start Module.vi that the module has launched and will let the code calling Start Module.vi register for broadcasts and would permit the caller receive the broadcast that an error occurred at launch time."
      n389 = call-dynamic "Delacor_lib_QMH_Release Message Queue.vi"("error in"=w943, "Message Queue"=w936) -> ("error out"=w942:errorcluster)  [unwired: 9 in]
      n390 = call "Synchronize Caller Events.vi"("Singleton Module Admin in"=w937) -> ("error out"=w944:errorcluster)  [unwired: 9 in, 1 out]
      n391 = call "Module Name--constant.vi"() -> ("Module Name"=w940:string)  [unwired: 11 in]
      n392 = Format Into String(format string="An error occurred during initialization. %s is no longer running.", w940) -> (resulting string=w938:string)  [unwired: 2 in, 1 out]
      n393 = Merge Errors(w942, w944) -> (w945:errorcluster)
      n394 = call "Error Reported.vi"("Additional Information"=w938, "Error"=w945) -> ()  [unwired: 9 in, 1 out]
    }
  }
  n395 = Merge Errors(w15, w18) -> (w14:errorcluster)
  n396 = call "Close Module.vi"("error in"=w14, "Module Admin in"=w9) -> ("error out"=w16:errorcluster, "External Launch"=w2:bool, "Module Admin out"=w3:refnum<class "Delacor_lib_QMH_Module Admin.lvclass">)  [unwired: 7 in]
  n397 = Unregister For Events(event registration refnum=w8, error in=w16) -> (error out=w13:errorcluster)
  "error out" <- w13
  n398 = case "External Launch?" shown="True" w2 {
    tunnel: w13 -> [_ w946]
    frame False {
    }
    frame True {
      n399 = case shown="No Error" w946 {
        frame No Error {
          n400 = invoke on="Invoke Node" class="VI" method="FP.Close"() -> ()  [unwired: 3 in, 3 out]
        }
        frame Error {
          n401 = disable-structure shown="Default" {
            frame condition #0 (active) {
              n402 = invoke class="VI" method="FP.Open"("Activate"=TRUE ("Activate?")) -> ()  [unwired: 4 in, 5 out]
            }
            frame condition #1 {
              # "Don't show panel on error if running inside a built EXE."
            }
          }
        }
      }
    }
  }
  n403 = local write "Module Admin"(w3) -> ()
